vi "Main_Marvin Remake.vi"() -> ()   [LabVIEW 2017]
uses:
  PCAN_Driver/ControlCAN.llb/DevType.ctl
  PCAN_Driver/ControlCAN.llb/CAN Channel.ctl
  PCAN_Driver/ControlCAN.llb/VCI_INIT_CONFIG.ctl
  PCAN_Driver/ControlCAN.llb/InitFlag.ctl
  PCAN_Driver/ControlCAN.llb/Fliter.ctl
  PCAN_Driver/ControlCAN.llb/Mode.ctl
  <vilib>/Utility/miscctls.llb/LVRowAndColumnTypeDef.ctl
  <vilib>/Utility/sysdir.llb/System Directory Type.ctl
  <vilib>/Utility/config.llb/Read Key (String).vi
  <vilib>/Utility/config.llb/Write Key (String).vi
  <vilib>/Utility/cursorutil.llb/Set Cursor (Icon Pict).vi
  PCAN_Driver/ControlCAN.lvlib
  <vilib>/Utility/config.llb/NI_LVConfig.lvlib
panel:
  out "DSP Board S/N":string
  out "POWER Board S/N":string caption="DRIVER Board S/N"
  out "BurnInSpeed":u16
  out "SpeedCommandSpeed":u16
  out "VenableSpeed":u16
  out "CurrentTest":T1(ring)
  out "TesterVersion":string
  out "ClosePanel":bool=TRUE
  out "UUT SN Report":string
  out "Automation":bool
  out "Test Failed":bool
  out "AuxiOFFResult":bool
  out "AuxiONResult":bool
  out "SensCalResult":bool
  out "VisualInspectionResult":bool
  out "BurnResult":bool
  out "BurnSpeed":bool
  out "BurnTemp":bool
  out "BurnDC":bool
  out "TempControlResult":bool
  out "MotorTempResult":bool
  out "StopTimeResult":bool
  out "SpeedResult":bool=TRUE
  out "VenableDirectionResult":bool
  out "VenableResult":bool
  out "ComTestResult":bool=TRUE
  out "UUT SoftwareVer":string
  out "Next SN":i32
  in  "SetSN":bool
  out "Current SN":i32
  out "Cal":dbl
  out "AO[1]Meas":dbl
  out "FullSpeed2 Speed":dbl
  out "FullSpeed2 Current":dbl
  out "FullSpeed1 Current":dbl
  out "FullSpeed1 Speed":dbl
  out "MaxBurnInTempVal":dbl
  in  "Stop Burn-in":bool
  out "VISA Tester":refnum<visa-resource-name>
  out "UUT":u8
  out "CAN Status":bool
  in  "Channel 2":T2 caption="Channel" items=["Channel 1", "Channel 2"]
  out "Config_CANAT":T8 {"DevType" items=["USB-CAN"=3, "USB-CAN2"=4]; "CanIndex" items=["通道1", "通道2"]; "VCI_INIT_CONFIG"."Fliter" items=["接收所有类型"=3, "只接收标准帧"=4, "只接收扩展帧"=7]; "VCI_INIT_CONFIG"."Mode" items=["正常工作", "自测模式（环回）", "仅侦听模式"]; "VCI_INIT_CONFIG"."InitFlag" items=["使用Flash参数", "使用界面设置参数"]}
  out "Array":u64[][](array[numeric]) format="%016x"
  out "Motor Phase Current RMS":dbl
  out "Ambient Temperature":dbl
  out "Speed error":bool
  out "Commutation err":bool
  out "Under voltage/Over voltage":bool
  out "Derated drive temp":bool
  out "Motor Over temperature":bool
  out "Motor Sensor temp Fauilre":bool
  out "Drive Over temperature":bool
  out "Drive Sensor temp Failure":bool
  out "Ambient Over temp":bool
  out "Ambient Sensor temp":bool
  out "DC Voltage":dbl
  out "DC Current":dbl
  out "Power transistor Heat sink Temp.":dbl
  out "Motor Stator Temp.":dbl
  out "Motor Speed RPM":dbl
  out "ECS State":u16
  out "UUT":string="EBAY"
  in  "Logger Path":path
  in  "Report":bool
  in  "Start":bool
  in  "ATR":string[][](table)=[["Test Communication", "-", "-", "-", "-", ""], ["Set S/N", "-", "-", "-", "-", ""], ["Set Board Number", "-", "-", "-", "-", ""], [" ", "", "", "", "", ""], ["Test Communication", "-", "-", "-", "-", ""], ["Get S/N", "-", "-", "-", "", ""], ["Get Board Number", "-", "-", "-", "", ""], ["Get FW", "-", "-", "-", "", ""], ["Enable Motor", "", "", "", "", ""], ["Small position command", "", "", "", "", ""], ["Measure delta", "", "", "", "", ""], ["Velocity command", "", "", "", "", ""]]
  in  "Settings":bool
  in  "Refresh Button":bool
  out "Status":bool
  in  "VISA Marvin":refnum<visa-resource-name>="COM6"
  in  "Serial Com":bool
  in  "Help Button":bool
  out "Pannel User Message":string
  in  "Stop Button":bool
  # "Marvin"
  # "REDLER TECHNOLOGIES LTD"
  # "ver 1.2p"
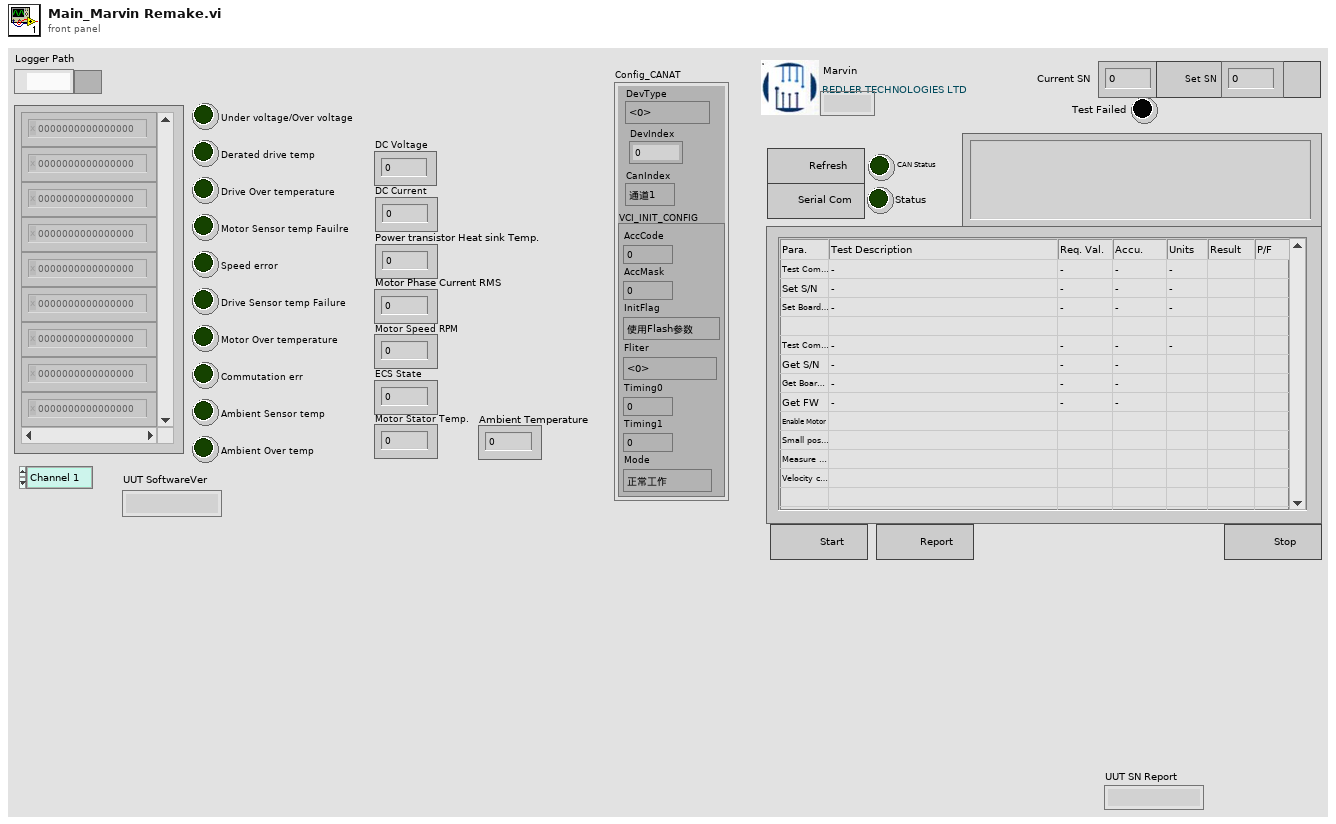
[diagram p1: front panel]
types:
  T1 = enum16{"Auxiliary", "Temp Sens Cal", "Com Test", "Enable Test", "Speed Command", "Stop Time", "Temp Control", "Burn in", "Visual Inspec", "Empty"}
  T2 = typedef "ControlCAN.lvlib/CAN Channel.ctl" = u32
  T3 = typedef "ControlCAN.lvlib/DevType.ctl" = u32
  T4 = typedef "ControlCAN.lvlib/VCI_INIT_CONFIG.ctl" = cluster{"AccCode":u32, "AccMask":u32, "InitFlag":T5, "Fliter":T6, "Timing0":u8, "Timing1":u8, "Mode":T7}
  T5 = typedef "ControlCAN.lvlib/InitFlag.ctl" = u32
  T6 = typedef "ControlCAN.lvlib/Fliter.ctl" = u8
  T7 = typedef "ControlCAN.lvlib/Mode.ctl" = u8
  T8 = cluster{"DevType":T3, "DevIndex":u32, "CanIndex":T2, "VCI_INIT_CONFIG":T4}
  T9 = cluster{"VISA":refnum<visa-resource-name>, "Array Test":enum16{"Auxiliary", "Temp Sens Cal", "Com Test", "Enable Test", "Speed Command", "Stop Time", "Temp Control", "Burn in", "Visual Inspec", "Empty"}[]}
  T10 = cluster{"ID":u32, "MSGTYPE":u8, "LEN":u8, "aDATA":u8[]}[]
  T11 = enum16{"Erase ATR Table", "Stop", "MainProgram", "Initialize"}
  T12 = typedef "NI_LVConfig.lvlib/Config Data RefNum.ctl" = refnum<k1>
  T13 = enum16{"K15", "K16", "K17", "Venable", "Firmeware", "Fan", "Power", "120C", "110C", "100C", "90C", "80C", "70C", "60C", "50C", "40C", "30C", "25C", "20C", "10C", "0C"}
  T14 = enum16{"Stop", "Result", "FullSpeed2", "MD[1]=1", "FullSpeed1", "MD[1]=0"}
  T15 = enum8{"Term1", "Term2", "Current", "Fan", "TempCPU"}
  T16 = enum16{"Stop", "AO[1]=Meas.", "TA[5]", "AO[1]=0", "Start"}
  T17 = enum16{"Stop", "BurnIn", "Ambient Temp", "MotorSpeed", "DC Current Measure", "Start"}
  T18 = enum16{"Auxiliary", "Temp Sens Cal", "Com Test", "Enable Test", "Speed Command", "Stop Time", "Temp Control", "Burn in", "Visual Inspec", "Empty"}[]
  T19 = enum16{"K15", "K16", "K17", "Venable", "Firmeware", "Fan", "Power", "120C", "110C", "100C", "90C", "80C", "70C", "60C", "50C", "40C", "30C", "25C", "20C", "10C", "0C"}[]
  T20 = enum32{"6000", "11500", "15100", "11500-2", "6000-2"}[]
  T21 = enum8{"Enabled", "Disabled", "Disabled and Grayed Out"}
  T22 = typedef "LVRowAndColumnTypeDef.ctl" = cluster{"Row":i32, "Column":i32}
  T23 = enum32{"Invalid", "Standard", "Closed", "Hidden", "Minimized", "Maximized"}
  T24 = cluster{"ID":u32, "MSGTYPE":u8, "LEN":u8, "aDATA":u8[]}
  T25 = enum16{"open", "replace", "create", "open or create", "replace or create", "replace or create with confirmation"}
  T26 = typedef "ControlCAN.lvlib/VCI_CAN_OBJ.ctl" = cluster{"ID":u32, "TimeStamp":u32, "TimeFlag":u8, "SendType":u8, "RemoteFlag":u8, "ExternFlag":u8, "DataLen":u8, "Data":u8[], "Reserved":u8[]}
  T27 = cluster{"Type":enum16{"接收", "发送"}, "Channel":T2, "Time":timestamp, "VCI_CAN_OBJ":T26}[]
  T28 = cluster{"Type":enum16{"接收", "发送"}, "Channel":T2, "Time":timestamp, "VCI_CAN_OBJ":T26}
  T29 = typedef "LVPoint32TypeDef.ctl" = cluster{"Horizontal":i32, "Vertical":i32}
  T30 = enum8{"Term1", "Term2", "Current", "Fan", "TempCPU"}[]
  T31 = typedef "System Directory Type.ctl" = i32
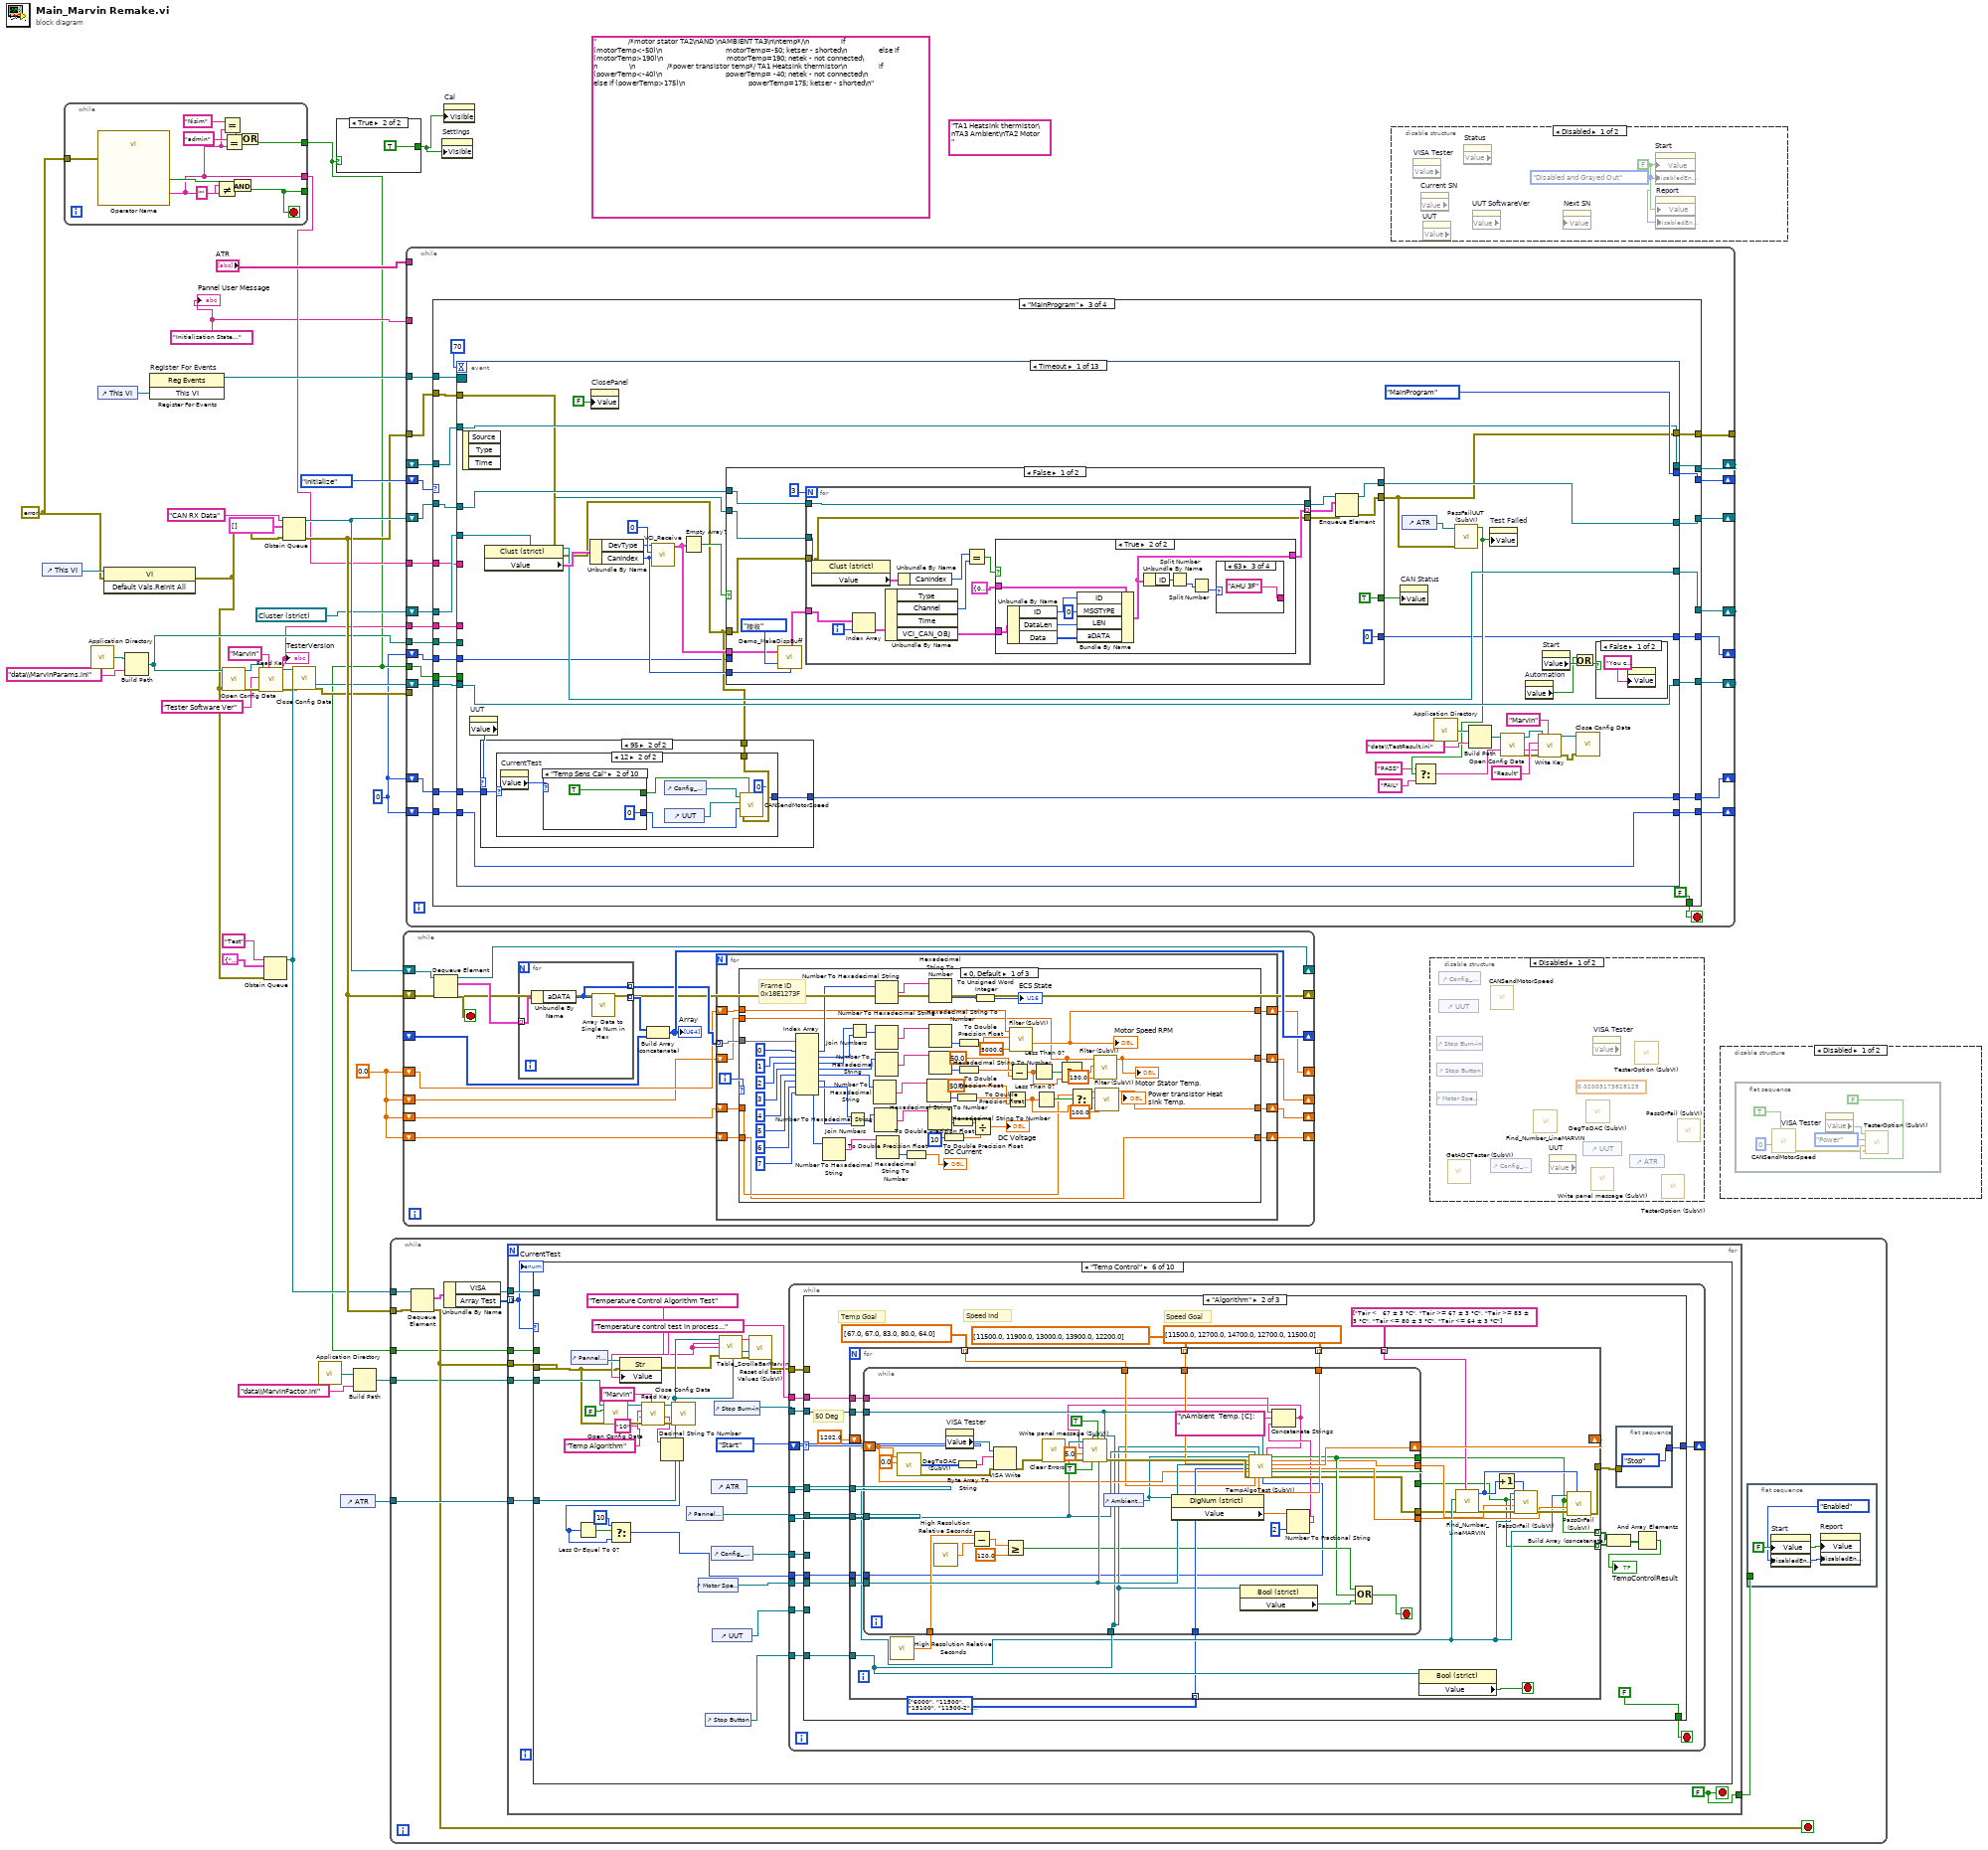
[diagram p0: block diagram]
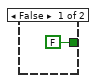
[diagram p2: hidden frame]
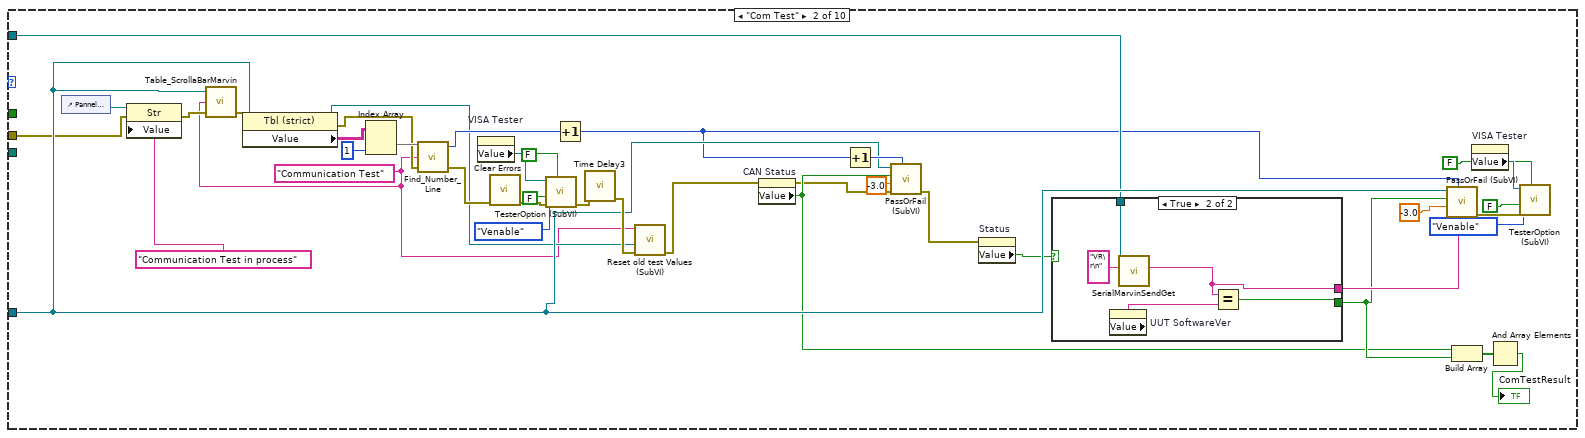
[diagram p7: hidden frame]
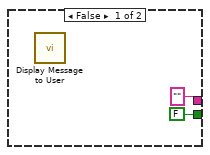
[diagram p8: hidden frame]
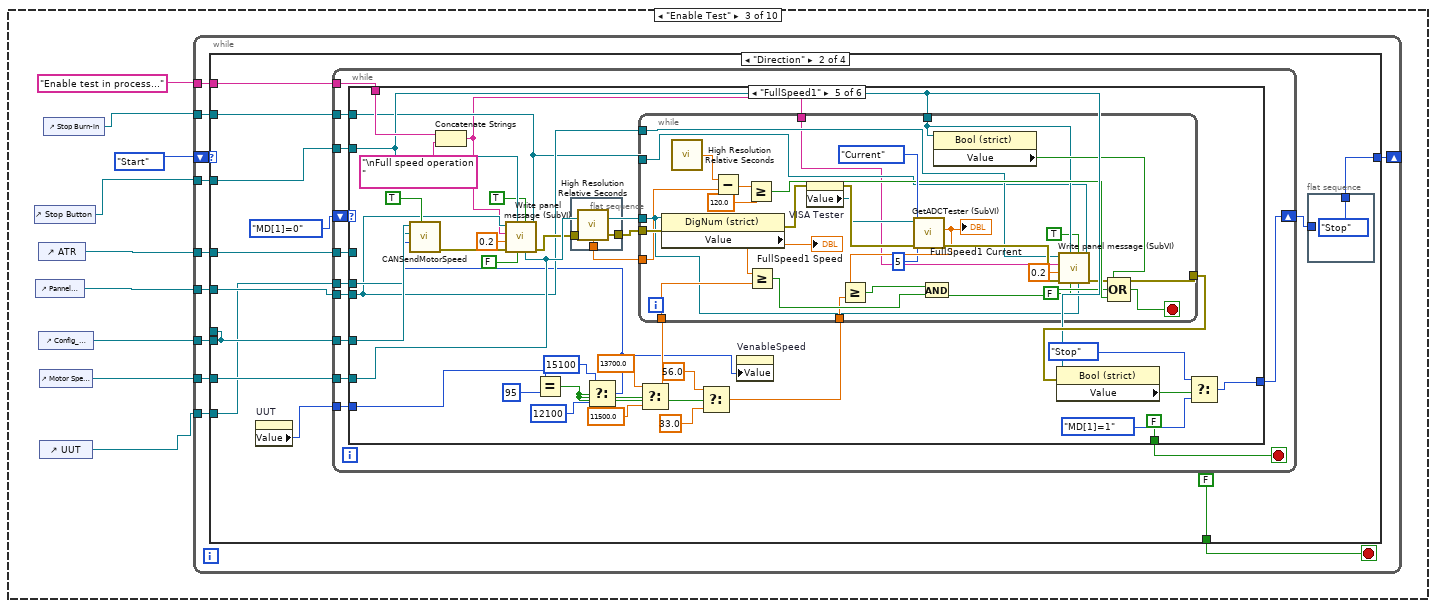
[diagram p9: hidden frame]
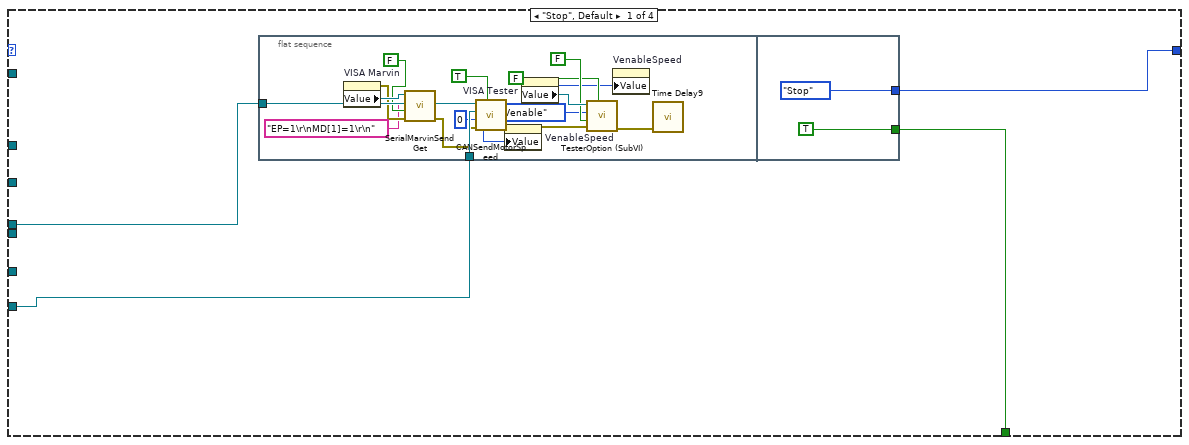
[diagram p10: hidden frame]
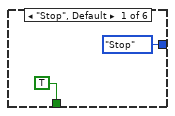
[diagram p11: hidden frame]
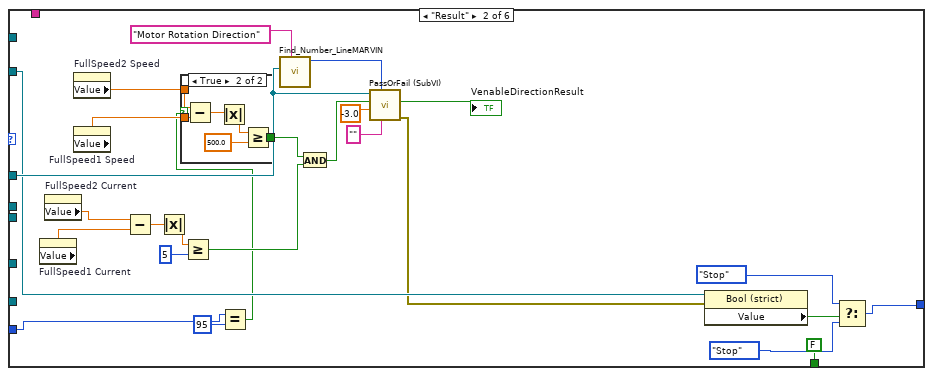
[diagram p12: hidden frame]
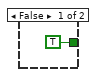
[diagram p13: hidden frame]
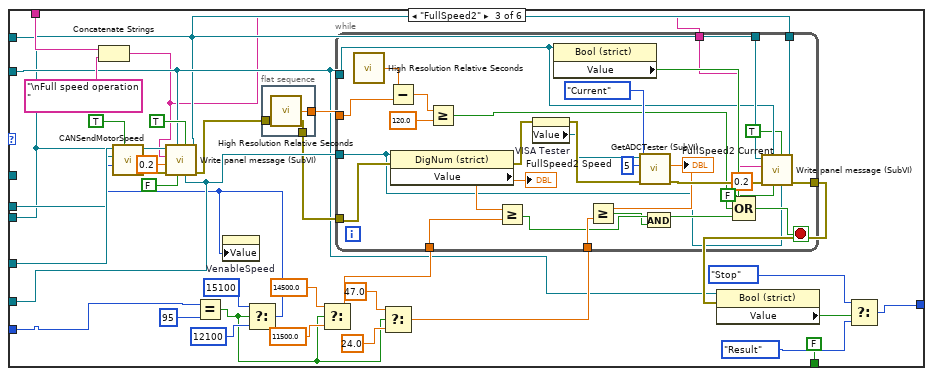
[diagram p14: hidden frame]
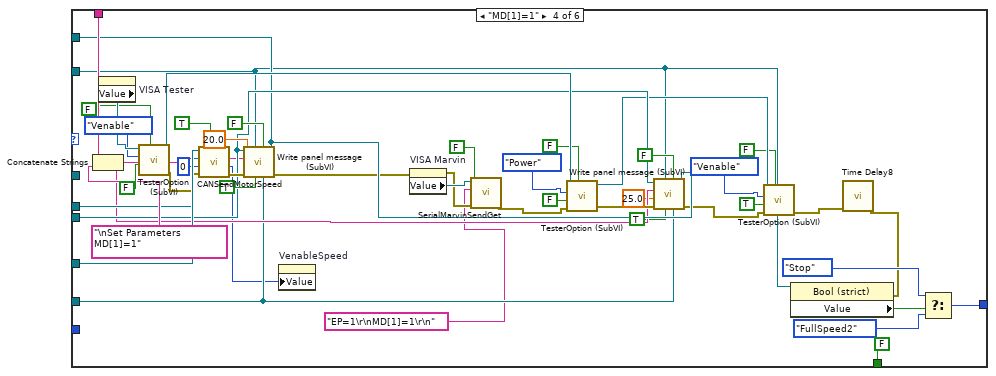
[diagram p15: hidden frame]
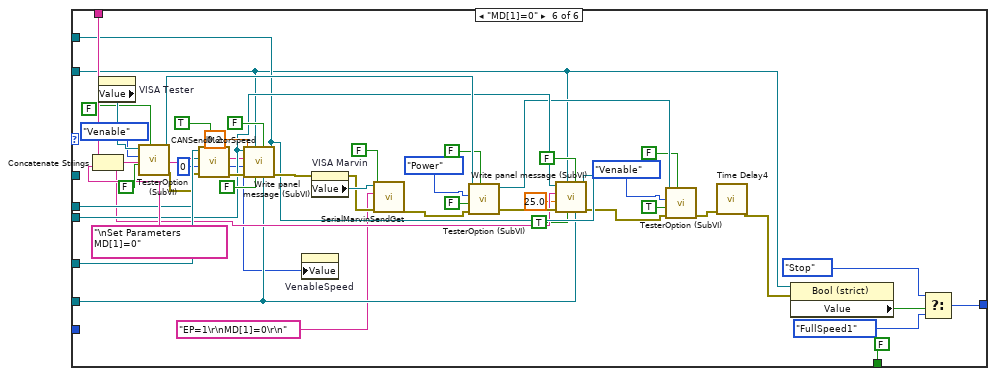
[diagram p16: hidden frame]
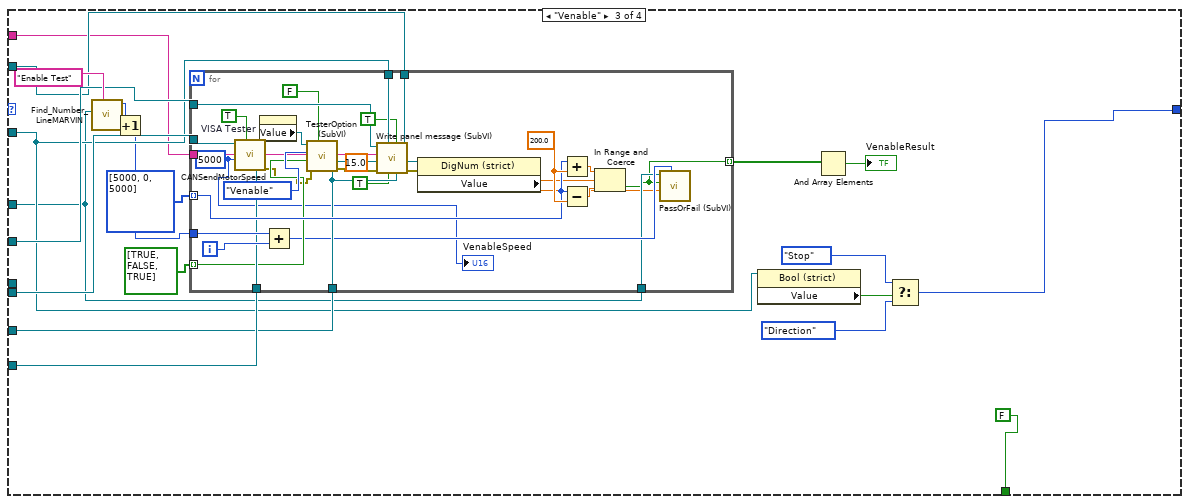
[diagram p17: hidden frame]
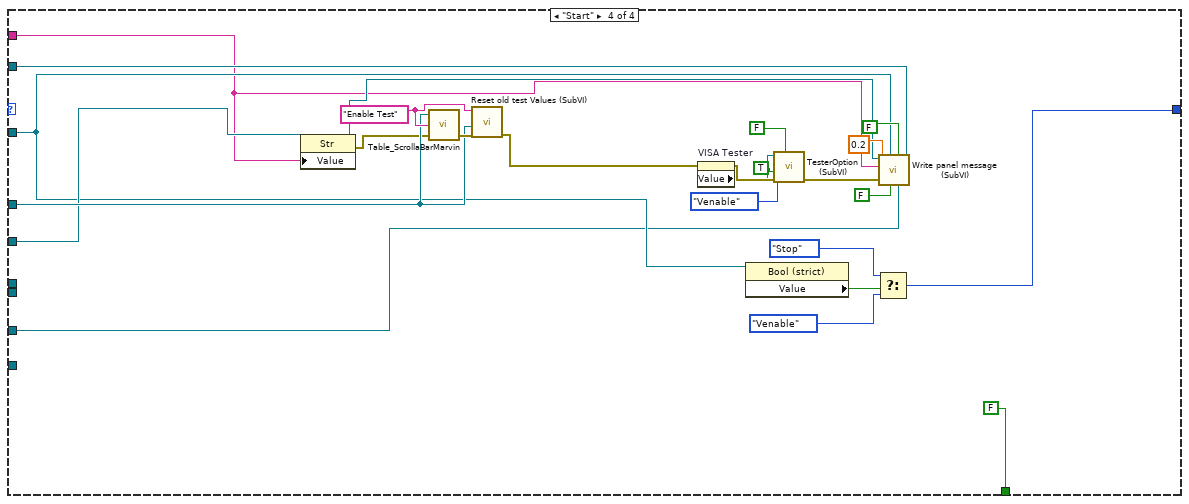
[diagram p18: hidden frame]
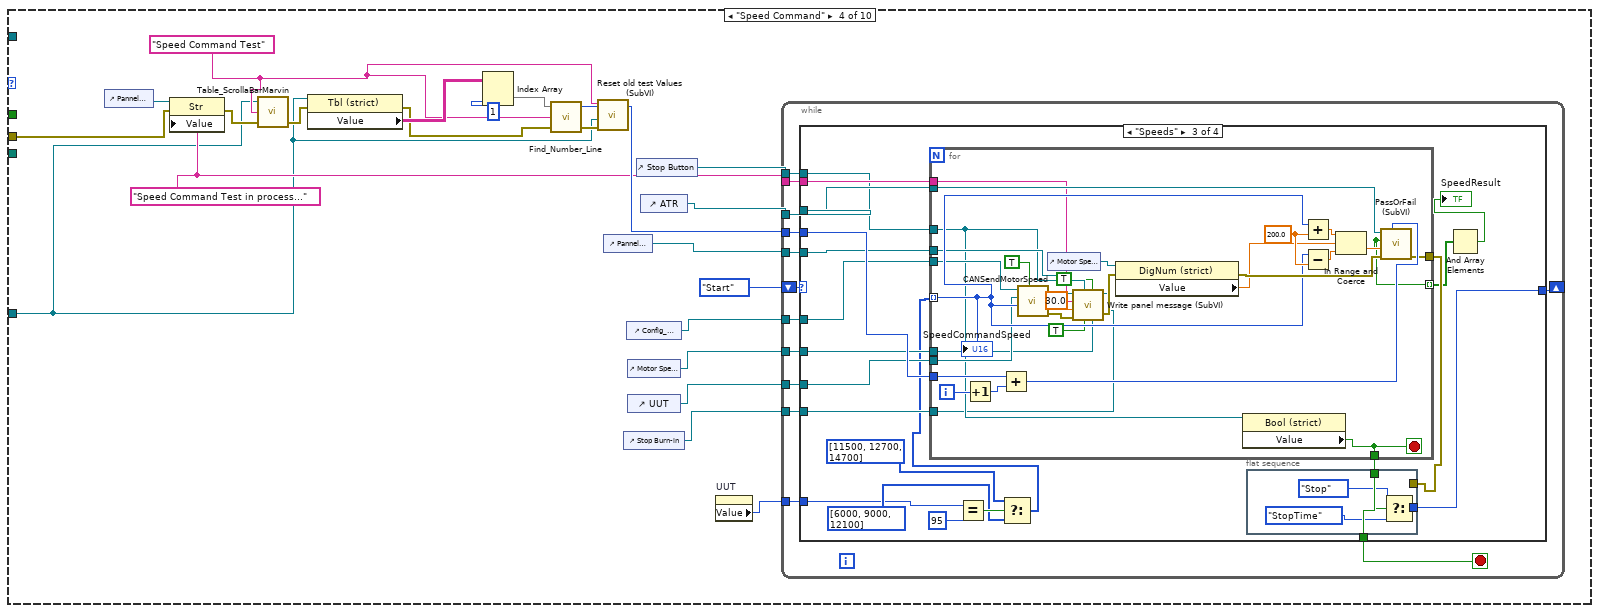
[diagram p19: hidden frame]
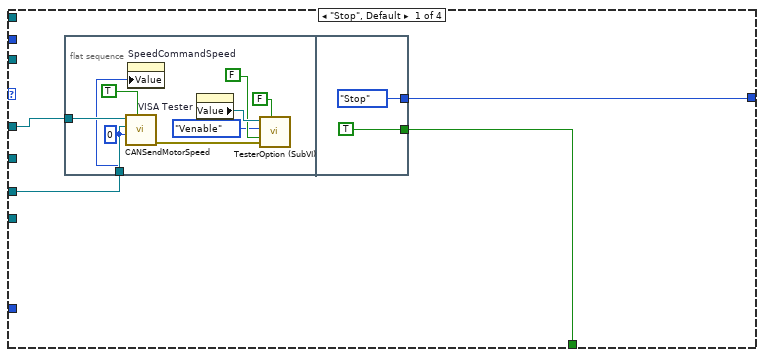
[diagram p20: hidden frame]
diagram:
  (unwired) "TA1 Heatsink thermistor\nTA3 Ambient\nTA2 Motor "
  (unwired) "                /*motor stator TA2\nAND \nAMBIENT TA3\n\ntemp*/\n                if (motorTemp<-50)\n                                motorTemp=-50; ketser - shorted\n                else if (motorTemp>190)\n                                motorTemp=190; netek - not connected\n                \n                /*power transistor temp*/ TA1 Heatsink thermistor\n                if (powerTemp<-40)\n                                powerTemp= -40; netek - not connected\n                else if (powerTemp>175)\n                                powerTemp=175; ketser - shorted\n"
  w19 = "Initialization State..."
  w1 = 0
  w26 = 0.0
  w4 = errorcluster {"status"=FALSE, "code"=0, "source"=""} ("error in (no error)")
  n1 = control-ref of="This VI"() -> (w5:refnum<vi>)
  n2 = while {
    tunnel: [w44] -> _
    tunnel: [w40] -> w21
    tunnel: [w41] -> w2
    tunnel: w4 -> [w37]
    stop <- w44 stop-if-true
    n3 = call "Operator Name"("error in (no error)"=w37) -> ("Operator Name"=w40:string, "OK"=w45:bool)  [unwired: 16 in, 1 out]
    n4 = Not Equal?(x=w40, y="") -> (x != y?=w46:bool)
    n5 = Equal?(x="Nisim", y=w40) -> (x = y?=w38:bool)
    n6 = Equal?(x="admin", y=w40) -> (x = y?=w42:bool)
    n7 = And(x=w45, y=w46) -> (x .and. y?=w44:bool)
    n8 = Or(x=w38, y=w42) -> (x .or. y?=w41:bool)
  }
  n9 = call <vilib>:"Application Directory.vi"() -> ("Application Directory"=w25:path)
  n10 = control-ref of="This VI"() -> (w23:refnum<vi>)
  n11 = invoke class="VI" method="Default Vals.Reinit All"(reference=w5, error in=w4) -> (error out=w3:errorcluster)  [unwired: 1 in, 2 out]
  n12 = Build Path(base path=w25, name or relative path="data\\MarvinParams.ini") -> (appended path=w8:path)
  n13 = register-events "Register For Events"(w23) -> (reference out=w22:refnum<event-registration>)  [unwired: 2 in, 1 out]
  n14 = call <vilib>:"Open Config Data.vi"("error in (no error)"=w3, "configuration file path"=w8) -> ("error out"=w14:errorcluster, "refnum"=w13:T12)  [unwired: 1 in, 7 out]
  n15 = call-poly <vilib>:"Read Key.vi"("section"="Marvin", "error in (no error)"=w14, "key"="Tester Software Ver", "refnum"=w13) -> ("error out"=w11:errorcluster, "value"=w6:string, "refnum out"=w10:T12)  [unwired: 2 in, 3 out]
  "TesterVersion" <- w6
  n16 = Obtain Queue(name (unnamed)="Test", element data type=T9 {"VISA"="COM1", "Array Test"=[]}, error in (no error)=w3) -> (queue out=w30:refnum<queue>)  [unwired: 2 in, 2 out]
  n17 = Obtain Queue(name (unnamed)="CAN RX Data", element data type=T10 [], error in (no error)=w3) -> (queue out=w33:refnum<queue>, error out=w31:errorcluster)  [unwired: 2 in, 1 out]
  n18 = call <vilib>:"Close Config Data.vi"("error in (no error)"=w11, "refnum"=w10) -> ("error out"=w9:errorcluster)  [unwired: 8 in, 1 out]
  n19 = call <vilib>:"Application Directory.vi"() -> ("Application Directory"=w16:path)
  n20 = case shown="True" w2 {
    tunnel: [FALSE TRUE] -> w20
    frame False {
    }
    frame True {
    }
  }
  n21 = control-ref of="ATR"() -> (w18:refnum<vi>)
  n22 = Build Path(base path=w16, name or relative path="data\\MarvinFactor.ini") -> (appended path=w15:path)
  n23 = while {
    tunnel: w18 -> [w59]
    tunnel: w31 -> [w57]
    tunnel: w30 -> [w58]
    tunnel: w15 -> [w51]
    tunnel: w2 -> [w50]
    stop <- w53 stop-if-true
    n24 = Dequeue Element(queue=w58, error in (no error)=w57) -> (element=w56:T9, error out=w53:errorcluster)  [unwired: 1 in, 2 out]
    n25 = Unbundle By Name(w56) -> ("VISA"=w55:refnum<visa-resource-name>, "Array Test"=w54:T18)
    n26 = for {
      tunnel: w54 -> [w65] mode=indexing
      tunnel: w55 -> [w68]
      tunnel: w59 -> [w67]
      tunnel: w53 -> [w66]
      tunnel: [w64] -> w52
      tunnel: w51 -> [w63]
      tunnel: w50 -> [w62]
      stop <- w64 stop-if-true
      w64 = FALSE
      n27 = case shown="\"Temp Control\"" w65 {
        tunnel: w68 -> [_ w93 _ _ w682 _ _ _ w1289 w1496]
        tunnel: w67 -> [_ w100 _ w517 w678 w855 _ w1249 w1296 w1509]
        tunnel: w66 -> [_ w97 _ w532 w688 w837 _ w1247 w1294 w1508]
        tunnel: w63 -> [_ _ _ _ _ w839 _ _ _ _]
        tunnel: w62 -> [_ _ _ _ _ _ w1007 _ _ _]
        frame "Empty", Default {
        }
        frame "Com Test" {
          w76 = "Communication Test" ("Test Paragraph")
          n28 = control-ref of="Pannel User Message"() -> (w98:refnum<vi>)
          n29 = property class="Str"(reference=w98, error in=w97, "Value"="Communication Test in process") -> (error out=w96:errorcluster)  [unwired: 1 out]
          n30 = call "Table_ScrollaBarMarvin.vi"("error in"=w96, "Line to focus"=w76, "reference in"=w100) -> ("error out"=w99:errorcluster)  [unwired: 2 out]
          n31 = property class="Tbl (strict)"(reference=w100, error in=w99) -> (reference out=w77:refnum<vi>, error out=w106:errorcluster, "Value"=w107:string[][])
          n32 = Index Array(array=w107, index (col)=1 ("disabled index (col)")) -> (element=w108:string[])  [unwired: 1 in]
          n33 = call "Find_Number_Line.vi"("error in"=w106, "Test Paragraph"=w76, "Row Headers[]"=w108) -> ("error out"=w104:errorcluster, "Line number"=w103:i32)  [unwired: 1 out]
          n34 = property on="VISA Tester" class="VISAName"() -> ("Value"=w87:refnum<visa-resource-name>)  [unwired: 2 in, 2 out]
          n35 = call <vilib>:"Clear Errors.vi"("error in (no error)"=w104) -> ("error out"=w89:errorcluster)  [unwired: 5 in, 1 out]
          n36 = call "TesterOption (SubVI).vi"("2 Options"=FALSE, "error in (no error)"=w89, "On/Off"=FALSE, "Tester Option"=T13."Venable", "VISA Refnum in"=w87) -> ("error out"=w88:errorcluster)  [unwired: 5 in, 1 out]
          n37 = Increment(x=w103) -> (x+1=w69:i32)
          n38 = call "Time Delay3"("error in (no error)"=w88) -> ("error out"=w101:errorcluster)  [unwired: 10 in]
          n39 = call "Reset old test Values (SubVI).vi"("error in"=w101, "Atr in"=w77, "Test Paragraph"=w76) -> ("error out"=w71:errorcluster)  [unwired: 8 in]
          n40 = property on="CAN Status" class="Bool (strict)"(error in=w71) -> (error out=w70:errorcluster, "Value"=w72:bool)  [unwired: 1 in, 1 out]
          n41 = Increment(x=w69) -> (x+1=w102:i32)
          n42 = call "PassOrFail (SubVI).vi"("index (row)"=w102, "error in (no error)"=w70, "Data in"=-3.0, "Pass?Fail"=w72, "Table in"=w100) -> ("error out"=w92:errorcluster)  [unwired: 6 in]
          n43 = property on="Status" class="Bool (strict)"(error in=w92) -> ("Value"=w94:bool)  [unwired: 1 in, 2 out]
          n44 = case shown="True" w94 {
            tunnel: w93 -> [_ w115]
            tunnel: [FALSE w112] -> w74
            tunnel: ["" ("read buffer") w111] -> w91
            frame False {
              n45 = call "Display Message to User"() -> ()  [unwired: 10 in, 2 out]
            }
            frame True {
              n46 = property on="UUT SoftwareVer" class="Str"() -> ("Value"=w113:string)  [unwired: 2 in, 2 out]
              n47 = call "SerialMarvinSendGet.vi"("write buffer"="VR\r\n", "VISA resource name"=w115) -> ("read buffer"=w111:string)  [unwired: 8 in, 1 out]
              n48 = Equal?(x=w111, y=w113) -> (x = y?=w112:bool)
            }
          }
          n49 = call "PassOrFail (SubVI).vi"("String Res"=w91, "index (row)"=w69, "Data in"=-3.0, "Pass?Fail"=w74, "Table in"=w100) -> ("error out"=w83:errorcluster)  [unwired: 6 in]
          n50 = Build Array(w72, w74) -> (w75:bool[])
          n51 = property on="VISA Tester" class="VISAName"() -> ("Value"=w82:refnum<visa-resource-name>)  [unwired: 2 in, 2 out]
          n52 = And Array Elements(Boolean array=w75) -> (logical AND=→"ComTestResult":bool)
          n53 = call "TesterOption (SubVI).vi"("2 Options"=FALSE, "error in (no error)"=w83, "On/Off"=FALSE, "Tester Option"=T13."Venable", "VISA Refnum in"=w82) -> ()  [unwired: 5 in, 2 out]
        }
        frame "Enable Test" {
          n54 = control-ref of="Stop Button"() -> (w118:refnum<vi>)
          n55 = control-ref of="Pannel User Message"() -> (w120:refnum<vi>)
          n56 = control-ref of="ATR"() -> (w119:refnum<vi>)
          n57 = control-ref of="Config_CANAT"() -> (w121:refnum<vi>)
          n58 = control-ref of="Motor Speed RPM"() -> (w122:refnum<vi>)
          n59 = control-ref of="UUT"() -> (w123:refnum<vi>)
          n60 = control-ref of="Stop Burn-in"() -> (w124:refnum<vi>)
          n61 = while {
            shift-right: [w129] -> _
            shift-left: enum16{"Stop", "Direction", "Venable", "Start"}."Start" -> [w135]
            tunnel: w118 -> [w134]
            tunnel: w119 -> [w133]
            tunnel: w120 -> [w132]
            tunnel: w121 -> [w125]
            tunnel: w122 -> [w131]
            tunnel: w123 -> [w126]
            tunnel: w124 -> [w128]
            tunnel: "Enable test in process..." ("Strin") -> [w127]
            stop <- w130 stop-if-true
            n62 = case shown="\"Direction\"" w135 {
              tunnel: w134 -> [_ w167 w449 w496]
              tunnel: w133 -> [_ w162 w447 w503]
              tunnel: w132 -> [_ w165 w451 w502]
              tunnel: w125 -> [_ w168 w454 _]
              tunnel: w131 -> [_ w164 w452 w494]
              tunnel: w126 -> [w136 w158 w453 _]
              tunnel: [w139 FALSE FALSE FALSE] -> w130
              tunnel: [w137 w161 w448 w500] -> w129
              tunnel: w128 -> [_ w166 w450 w495]
              tunnel: w127 -> [_ w163 w446 w493]
              tunnel: w125 -> [w138 _ _ _]
              frame "Stop", Default {
                n63 = flat-sequence {
                  tunnel: w136 -> [w151]
                  tunnel: w138 -> [w150]
                  tunnel: [TRUE] -> w139
                  tunnel: [enum16{"Stop", "Direction", "Venable", "Start"}."Stop"] -> w137
                  frame #0 {
                    w140 = u16 0 ("Motor Speed RPM")
                    n64 = property on="VISA Marvin" class="VISAName"() -> (error out=w144:errorcluster, "Value"=w145:refnum<visa-resource-name>)  [unwired: 2 in, 1 out]
                    n65 = call "SerialMarvinSendGet.vi"("error in (no error)"=w144, "Clear Log"=FALSE, "write buffer"="EP=1\r\nMD[1]=1\r\n", "VISA resource name"=w145) -> ("error out"=w141:errorcluster)  [unwired: 6 in, 1 out]
                    n66 = call "CANSendMotorSpeed.vi"("Remote"=TRUE, "error in (no error)"=w141, "Motor Speed RPM"=w140, "UUT"=w151, "CAN Cluster in"=w150) -> ("error out"=w153:errorcluster)  [unwired: 6 in]
                    n67 = property on="VenableSpeed" class="DigNum (strict)"("Value"=w140) -> ()  [unwired: 2 in, 2 out]
                    n68 = property on="VISA Tester" class="VISAName"() -> ("Value"=w154:refnum<visa-resource-name>)  [unwired: 2 in, 2 out]
                    n69 = call "TesterOption (SubVI).vi"("2 Options"=FALSE, "error in (no error)"=w153, "On/Off"=FALSE, "Tester Option"=T13."Venable", "VISA Refnum in"=w154) -> ("error out"=w146:errorcluster)  [unwired: 5 in, 1 out]
                    n70 = property on="VenableSpeed" class="DigNum (strict)"("Value"=w140) -> ()  [unwired: 2 in, 2 out]
                    n71 = call "Time Delay9"("error in (no error)"=w146) -> ()  [unwired: 10 in, 1 out]
                  }
                  frame #1 {
                  }
                }
              }
              frame "Direction" {
                n72 = property on="UUT" class="DigNum (strict)"() -> ("Value"=w157:u8)  [unwired: 2 in, 2 out]
                n73 = while {
                  shift-right: [w181] -> w160
                  shift-left: T14."MD[1]=0" -> [w182]
                  tunnel: w168 -> [w179]
                  tunnel: w158 -> [w178]
                  tunnel: w167 -> [w177]
                  tunnel: w166 -> [w176]
                  tunnel: w165 -> [w175]
                  tunnel: w164 -> [w174]
                  tunnel: w163 -> [w173]
                  tunnel: w162 -> [w172]
                  tunnel: w157 -> [w171]
                  stop <- w180 stop-if-true
                  n74 = case shown="\"FullSpeed1\"" w182 {
                    tunnel: [T14."Stop" w206 w248 w328 w361 w441] -> w181
                    tunnel: [TRUE FALSE FALSE FALSE FALSE FALSE] -> w180
                    tunnel: w179 -> [_ _ w246 w322 w359 w435]
                    tunnel: w178 -> [_ _ w242 w302 w355 w414]
                    tunnel: w177 -> [_ w193 w222 w293 w338 w404]
                    tunnel: w176 -> [_ _ w220 w303 w336 w415]
                    tunnel: w175 -> [_ _ w221 w304 w337 w416]
                    tunnel: w174 -> [_ _ w238 w291 w352 w410]
                    tunnel: w173 -> [_ _ w233 w312 w350 w424]
                    tunnel: w172 -> [_ w197 _ _ _ _]
                    tunnel: w171 -> [_ w185 w218 _ w331 _]
                    frame "Stop", Default {
                    }
                    frame "Result" {
                      n75 = property on="FullSpeed1 Current" class="DigNum (strict)"() -> ("Value"=w201:dbl)  [unwired: 2 in, 2 out]
                      n76 = property on="FullSpeed2 Current" class="DigNum (strict)"() -> ("Value"=w202:dbl)  [unwired: 2 in, 2 out]
                      n77 = property on="FullSpeed2 Speed" class="DigNum (strict)"() -> ("Value"=w204:dbl)  [unwired: 2 in, 2 out]
                      n78 = property on="FullSpeed1 Speed" class="DigNum (strict)"() -> ("Value"=w203:dbl)  [unwired: 2 in, 2 out]
                      n79 = Subtract(x=w202, y=w201) -> (x-y=w200:dbl)
                      n80 = Absolute Value(x=w200) -> (abs(x)=w189:dbl)
                      n81 = Greater Or Equal?(x=w189, y=u32 5) -> (x >= y?=w195:bool)
                      n82 = Equal?(x=w185, y=u8 95) -> (x = y?=w187:bool)
                      n83 = case shown="True" w187 {
                        tunnel: w204 -> [_ w215]
                        tunnel: w203 -> [_ w214]
                        tunnel: [TRUE w211] -> w196
                        frame False {
                        }
                        frame True {
                          n84 = Subtract(x=w215, y=w214) -> (x-y=w216:dbl)
                          n85 = Absolute Value(x=w216) -> (abs(x)=w213:dbl)
                          n86 = Greater Or Equal?(x=w213, y=500.0) -> (x >= y?=w211:bool)
                        }
                      }
                      n87 = call "Find_Number_LineMARVIN.vi"("Test Paragraph"="Motor Rotation Direction", "TableIn"=w197) -> ("Line number"=w194:i32)  [unwired: 3 in, 3 out]
                      n88 = And(x=w196, y=w195) -> (x .and. y?=w186:bool)
                      "VenableDirectionResult" <- w186
                      n89 = call "PassOrFail (SubVI).vi"("String Res"="", "index (row)"=w194, "Data in"=-3.0, "Pass?Fail"=w186, "Table in"=w197) -> ("error out"=w192:errorcluster)  [unwired: 6 in]
                      n90 = property class="Bool (strict)"(reference=w193, error in=w192) -> ("Value"=w209:bool)  [unwired: 2 out]
                      n91 = Select(t=T14."Stop", s=w209, f=T14."Stop") -> (s? t:f=w206:T14)
                    }
                    frame "FullSpeed2" {
                      n92 = Concatenate Strings(w233, "\nFull speed operation " ("string")) -> (w219:string)
                      n93 = Equal?(x=w218, y=u8 95) -> (x = y?=w228:bool)
                      n94 = Select(t=u16 15100, s=w228, f=u16 12100 ("y")) -> (s? t:f=w217:u16)
                      n95 = call "CANSendMotorSpeed.vi"("Remote"=TRUE, "Motor Speed RPM"=w217, "UUT"=w242, "CAN Cluster in"=w246) -> ("error out"=w240:errorcluster)  [unwired: 7 in]
                      n96 = call "Write panel message (SubVI).vi"("Stop BurnIn"=w220, 4:"rpm"=w238, 5:"rpm"=TRUE ("rpm"), "PrintTime"=FALSE, "Stop"=w222, "error in (no error)"=w240, "Time to wait"=0.2, "Strin"=w219, "String in"=w221) -> ("error out"=w225:errorcluster)  [unwired: 2 in]
                      n97 = property on="VenableSpeed" class="DigNum (strict)"("Value"=w217) -> ()  [unwired: 2 in, 2 out]
                      n98 = flat-sequence {
                        tunnel: w225 -> [w253]
                        tunnel: [w253] -> w224
                        tunnel: [w252] -> w223
                        frame #0 {
                          n99 = call <vilib>:"High Resolution Relative Seconds.vi"() -> ("relative seconds"=w252:dbl)
                        }
                      }
                      n100 = Select(t=14500.0, s=w228, f=11500.0) -> (s? t:f=w227:dbl)
                      n101 = Select(t=47.0, s=w228, f=24.0) -> (s? t:f=w226:dbl)
                      n102 = while {
                        tunnel: w238 -> [w255]
                        tunnel: w224 -> [w283]
                        tunnel: [w263] -> w235
                        tunnel: w227 -> [w276]
                        tunnel: w226 -> [w275]
                        tunnel: w223 -> [w271]
                        tunnel: w222 -> [w261]
                        tunnel: w221 -> [w262]
                        tunnel: w220 -> [w259]
                        tunnel: w219 -> [w258]
                        stop <- w273 stop-if-true
                        n103 = call <vilib>:"High Resolution Relative Seconds.vi"() -> ("relative seconds"=w272:dbl)
                        n104 = Subtract(x=w272, y=w271) -> (x-y=w270:dbl)
                        n105 = property class="DigNum (strict)"(reference=w255, error in=w283) -> (error out=w282:errorcluster, "Value"=w277:dbl)  [unwired: 1 out]
                        "FullSpeed2 Speed" <- w277
                        n106 = Greater Or Equal?(x=w270, y=120.0) -> (x >= y?=w268:bool)
                        n107 = Greater Or Equal?(x=w277, y=w276) -> (x >= y?=w267:bool)
                        n108 = property on="VISA Tester" class="VISAName"(error in=w282) -> (error out=w281:errorcluster, "Value"=w280:refnum<visa-resource-name>)  [unwired: 1 in, 1 out]
                        n109 = property class="Bool (strict)"(reference=w261) -> ("Value"=w266:bool)  [unwired: 1 in, 2 out]
                        n110 = call "GetADCTester (SubVI).vi"("error in (no error)"=w281, "GetADCTester"=T15."Current", "TimeToGet"=5, "VISA Refnum in"=w280) -> ("error out"=w278:errorcluster, "ADCValOutput Single"=w274:dbl)  [unwired: 5 in, 1 out]
                        "FullSpeed2 Current" <- w274
                        n111 = Greater Or Equal?(x=w274, y=w275) -> (x >= y?=w264:bool)
                        n112 = And(x=w267, y=w264) -> (x .and. y?=w265:bool)
                        n113 = Compound Arithmetic op=OR(w266, w268, w265) -> (w273:bool)
                        n114 = call "Write panel message (SubVI).vi"("Stop BurnIn"=w259, 4:"rpm"=w255, 5:"rpm"=TRUE ("rpm"), "PrintTime"=FALSE, "Stop"=w261, "error in (no error)"=w278, "Time to wait"=0.2, "Strin"=w258, "String in"=w262) -> ("error out"=w263:errorcluster)  [unwired: 2 in]
                      }
                      n115 = property class="Bool (strict)"(reference=w222, error in=w235) -> ("Value"=w251:bool)  [unwired: 2 out]
                      n116 = Select(t=T14."Stop", s=w251, f=T14."Result") -> (s? t:f=w248:T14)
                    }
                    frame "MD[1]=1" {
                      w284 = u16 0 ("Motor Speed RPM")
                      n117 = Concatenate Strings(w312, "\nSet Parameters MD[1]=1" ("Strin")) -> (w301:string)
                      n118 = property on="VISA Tester" class="VISAName"() -> ("Value"=w317:refnum<visa-resource-name>)  [unwired: 2 in, 2 out]
                      n119 = call "TesterOption (SubVI).vi"("2 Options"=FALSE, "On/Off"=FALSE, "Tester Option"=T13."Venable", "VISA Refnum in"=w317) -> ("error out"=w318:errorcluster, "VISA Refnum out"=w308:refnum<visa-resource-name>)  [unwired: 6 in]
                      n120 = call "CANSendMotorSpeed.vi"("Remote"=TRUE, "error in (no error)"=w318, "Motor Speed RPM"=w284, "UUT"=w302, "CAN Cluster in"=w322) -> ("error out"=w320:errorcluster)  [unwired: 6 in]
                      n121 = call "Write panel message (SubVI).vi"("Stop BurnIn"=w303, 4:"rpm"=w291, 5:"rpm"=FALSE ("rpm"), "PrintTime"=TRUE, "Stop"=w293, "error in (no error)"=w320, "Time to wait"=20.0, "Strin"=w301, "String in"=w304) -> ("error out"=w290:errorcluster)  [unwired: 2 in]
                      n122 = property on="VenableSpeed" class="DigNum (strict)"("Value"=w284) -> ()  [unwired: 2 in, 2 out]
                      n123 = property on="VISA Marvin" class="VISAName"(error in=w290) -> (error out=w319:errorcluster, "Value"=w324:refnum<visa-resource-name>)  [unwired: 1 in, 1 out]
                      n124 = call "SerialMarvinSendGet.vi"("error in (no error)"=w319, "Clear Log"=FALSE, "write buffer"="EP=1\r\nMD[1]=1\r\n", "VISA resource name"=w324) -> ("error out"=w307:errorcluster)  [unwired: 6 in, 1 out]
                      n125 = call "TesterOption (SubVI).vi"("2 Options"=FALSE, "error in (no error)"=w307, "On/Off"=FALSE, "Tester Option"=T13."Power", "VISA Refnum in"=w308) -> ("error out"=w305:errorcluster, "VISA Refnum out"=w294:refnum<visa-resource-name>)  [unwired: 5 in]
                      n126 = call "Write panel message (SubVI).vi"("Stop BurnIn"=w303, 4:"rpm"=w291, 5:"rpm"=FALSE ("rpm"), "PrintTime"=TRUE, "Stop"=w293, "error in (no error)"=w305, "Time to wait"=25.0, "Strin"=w301, "String in"=w304) -> ("error out"=w295:errorcluster)  [unwired: 2 in]
                      n127 = call "TesterOption (SubVI).vi"("2 Options"=FALSE, "error in (no error)"=w295, "On/Off"=TRUE, "Tester Option"=T13."Venable", "VISA Refnum in"=w294) -> ("error out"=w292:errorcluster)  [unwired: 5 in, 1 out]
                      n128 = call "Time Delay8"("error in (no error)"=w292) -> ("error out"=w288:errorcluster)  [unwired: 10 in]
                      n129 = property class="Bool (strict)"(reference=w293, error in=w288) -> ("Value"=w329:bool)  [unwired: 2 out]
                      n130 = Select(t=T14."Stop", s=w329, f=T14."FullSpeed2") -> (s? t:f=w328:T14)
                    }
                    frame "FullSpeed1" {
                      n131 = Concatenate Strings(w350, "\nFull speed operation " ("string")) -> (w335:string)
                      n132 = Equal?(x=w331, y=u8 95) -> (x = y?=w348:bool)
                      n133 = flat-sequence {
                        tunnel: w341 -> [w366]
                        tunnel: [w366] -> w340
                        tunnel: [w365] -> w339
                        frame #0 {
                          n134 = call <vilib>:"High Resolution Relative Seconds.vi"() -> ("relative seconds"=w365:dbl)
                        }
                      }
                      n135 = Select(t=u16 15100, s=w348, f=u16 12100 ("y")) -> (s? t:f=w330:u16)
                      n136 = call "CANSendMotorSpeed.vi"("Remote"=TRUE, "Motor Speed RPM"=w330, "UUT"=w355, "CAN Cluster in"=w359) -> ("error out"=w353:errorcluster)  [unwired: 7 in]
                      n137 = call "Write panel message (SubVI).vi"("Stop BurnIn"=w336, 4:"rpm"=w352, 5:"rpm"=TRUE ("rpm"), "PrintTime"=FALSE, "Stop"=w338, "error in (no error)"=w353, "Time to wait"=0.2, "Strin"=w335, "String in"=w337) -> ("error out"=w341:errorcluster)  [unwired: 2 in]
                      n138 = Select(t=13700.0, s=w348, f=11500.0) -> (s? t:f=w343:dbl)
                      n139 = Select(t=56.0, s=w348, f=33.0) -> (s? t:f=w342:dbl)
                      n140 = while {
                        tunnel: w352 -> [w368]
                        tunnel: w340 -> [w396]
                        tunnel: [w376] -> w351
                        tunnel: w343 -> [w388]
                        tunnel: w342 -> [w385]
                        tunnel: w339 -> [w383]
                        tunnel: w338 -> [w374]
                        tunnel: w337 -> [w375]
                        tunnel: w336 -> [w372]
                        tunnel: w335 -> [w371]
                        stop <- w390 stop-if-true
                        n141 = property class="DigNum (strict)"(reference=w368, error in=w396) -> (error out=w395:errorcluster, "Value"=w389:dbl)  [unwired: 1 out]
                        "FullSpeed1 Speed" <- w389
                        n142 = call <vilib>:"High Resolution Relative Seconds.vi"() -> ("relative seconds"=w384:dbl)
                        n143 = Subtract(x=w384, y=w383) -> (x-y=w382:dbl)
                        n144 = Greater Or Equal?(x=w382, y=120.0) -> (x >= y?=w380:bool)
                        n145 = Greater Or Equal?(x=w389, y=w388) -> (x >= y?=w387:bool)
                        n146 = property on="VISA Tester" class="VISAName"(error in=w395) -> (error out=w394:errorcluster, "Value"=w393:refnum<visa-resource-name>)  [unwired: 1 in, 1 out]
                        n147 = call "GetADCTester (SubVI).vi"("error in (no error)"=w394, "GetADCTester"=T15."Current", "TimeToGet"=5, "VISA Refnum in"=w393) -> ("error out"=w391:errorcluster, "ADCValOutput Single"=w386:dbl)  [unwired: 5 in, 1 out]
                        "FullSpeed1 Current" <- w386
                        n148 = Greater Or Equal?(x=w386, y=w385) -> (x >= y?=w377:bool)
                        n149 = And(x=w377, y=w387) -> (x .and. y?=w378:bool)
                        n150 = property class="Bool (strict)"(reference=w374) -> ("Value"=w379:bool)  [unwired: 1 in, 2 out]
                        n151 = call "Write panel message (SubVI).vi"("Stop BurnIn"=w372, 4:"rpm"=w368, 5:"rpm"=TRUE ("rpm"), "PrintTime"=FALSE, "Stop"=w374, "error in (no error)"=w391, "Time to wait"=0.2, "Strin"=w371, "String in"=w375) -> ("error out"=w376:errorcluster)  [unwired: 2 in]
                        n152 = Compound Arithmetic op=OR(w379, w378, w380) -> (w390:bool)
                      }
                      n153 = property on="VenableSpeed" class="DigNum (strict)"("Value"=w330) -> ()  [unwired: 2 in, 2 out]
                      n154 = property class="Bool (strict)"(reference=w338, error in=w351) -> ("Value"=w364:bool)  [unwired: 2 out]
                      n155 = Select(t=T14."Stop", s=w364, f=T14."MD[1]=1") -> (s? t:f=w361:T14)
                    }
                    frame "MD[1]=0" {
                      w397 = u16 0 ("Motor Speed RPM")
                      n156 = Concatenate Strings(w424, "\nSet Parameters MD[1]=0" ("Strin")) -> (w413:string)
                      n157 = property on="VISA Tester" class="VISAName"() -> ("Value"=w430:refnum<visa-resource-name>)  [unwired: 2 in, 2 out]
                      n158 = call "TesterOption (SubVI).vi"("2 Options"=FALSE, "On/Off"=FALSE, "Tester Option"=T13."Venable", "VISA Refnum in"=w430) -> ("error out"=w431:errorcluster, "VISA Refnum out"=w420:refnum<visa-resource-name>)  [unwired: 6 in]
                      n159 = call "CANSendMotorSpeed.vi"("Remote"=TRUE, "error in (no error)"=w431, "Motor Speed RPM"=w397, "UUT"=w414, "CAN Cluster in"=w435) -> ("error out"=w433:errorcluster)  [unwired: 6 in]
                      n160 = call "Write panel message (SubVI).vi"("Stop BurnIn"=w415, 4:"rpm"=w410, 5:"rpm"=FALSE ("rpm"), "PrintTime"=FALSE, "Stop"=w404, "error in (no error)"=w433, "Time to wait"=0.2, "Strin"=w413, "String in"=w416) -> ("error out"=w427:errorcluster)  [unwired: 2 in]
                      n161 = property on="VenableSpeed" class="DigNum (strict)"("Value"=w397) -> ()  [unwired: 2 in, 2 out]
                      n162 = property on="VISA Marvin" class="VISAName"(error in=w427) -> (error out=w432:errorcluster, "Value"=w437:refnum<visa-resource-name>)  [unwired: 1 in, 1 out]
                      n163 = call "SerialMarvinSendGet.vi"("error in (no error)"=w432, "Clear Log"=FALSE, "write buffer"="EP=1\r\nMD[1]=0\r\n", "VISA resource name"=w437) -> ("error out"=w419:errorcluster)  [unwired: 6 in, 1 out]
                      n164 = call "TesterOption (SubVI).vi"("2 Options"=FALSE, "error in (no error)"=w419, "On/Off"=FALSE, "Tester Option"=T13."Power", "VISA Refnum in"=w420) -> ("error out"=w417:errorcluster, "VISA Refnum out"=w405:refnum<visa-resource-name>)  [unwired: 5 in]
                      n165 = call "Write panel message (SubVI).vi"("Stop BurnIn"=w415, 4:"rpm"=w410, 5:"rpm"=FALSE ("rpm"), "PrintTime"=TRUE, "Stop"=w404, "error in (no error)"=w417, "Time to wait"=25.0, "Strin"=w413, "String in"=w416) -> ("error out"=w406:errorcluster)  [unwired: 2 in]
                      n166 = call "TesterOption (SubVI).vi"("2 Options"=FALSE, "error in (no error)"=w406, "On/Off"=TRUE, "Tester Option"=T13."Venable", "VISA Refnum in"=w405) -> ("error out"=w403:errorcluster)  [unwired: 5 in, 1 out]
                      n167 = call "Time Delay4"("error in (no error)"=w403) -> ("error out"=w399:errorcluster)  [unwired: 10 in]
                      n168 = property class="Bool (strict)"(reference=w404, error in=w399) -> ("Value"=w442:bool)  [unwired: 2 out]
                      n169 = Select(t=T14."Stop", s=w442, f=T14."FullSpeed1") -> (s? t:f=w441:T14)
                    }
                  }
                }
                n170 = flat-sequence {
                  tunnel: [enum16{"Stop", "Direction", "Venable", "Start"}."Stop"] -> w161
                  tunnel: w160 -> [_]
                  frame #0 {
                  }
                }
              }
              frame "Venable" {
                n171 = call "Find_Number_LineMARVIN.vi"("Test Paragraph"="Enable Test", "TableIn"=w447) -> ("Line number"=w455:i32)  [unwired: 3 in, 3 out]
                n172 = Increment(x=w455) -> (x+1=w443:i32)
                n173 = for {
                  tunnel: u16[] [5000, 0, 5000] -> [w485] mode=indexing
                  tunnel: bool[] [TRUE, FALSE, TRUE] -> [w481] mode=indexing
                  tunnel: w443 -> [w486]
                  tunnel: w454 -> [w484]
                  tunnel: w453 -> [w483]
                  tunnel: w452 -> [w472]
                  tunnel: w451 -> [w476]
                  tunnel: w449 -> [w475]
                  tunnel: w450 -> [w474]
                  tunnel: w447 -> [w468]
                  tunnel: w446 -> [w466]
                  tunnel: [w465] -> w445 mode=indexing
                  i -> [w487]
                  w463 = u16 5000 ("Motor Speed RPM")
                  w489 = 200.0 ("y")
                  n174 = call "CANSendMotorSpeed.vi"("Remote"=TRUE, "Motor Speed RPM"=w463, "UUT"=w483, "CAN Cluster in"=w484) -> ("error out"=w480:errorcluster)  [unwired: 7 in]
                  n175 = property on="VISA Tester" class="VISAName"() -> ("Value"=w479:refnum<visa-resource-name>)  [unwired: 2 in, 2 out]
                  n176 = Add(x=w486, y=w487) -> (x+y=w469:i32)
                  n177 = call "TesterOption (SubVI).vi"("2 Options"=FALSE, "error in (no error)"=w480, "On/Off"=w481, "Tester Option"=T13."Venable", "VISA Refnum in"=w479) -> ("error out"=w478:errorcluster)  [unwired: 5 in, 1 out]
                  n178 = call "Write panel message (SubVI).vi"("Stop BurnIn"=w474, 4:"rpm"=w472, 5:"rpm"=TRUE ("rpm"), "PrintTime"=TRUE, "Stop"=w475, "error in (no error)"=w478, "Time to wait"=15.0, "Strin"=w466, "String in"=w476) -> ("error out"=w477:errorcluster)  [unwired: 2 in]
                  n179 = property class="DigNum (strict)"(reference=w472, error in=w477) -> ("Value"=w467:dbl)  [unwired: 2 out]
                  n180 = Add(x=w485, y=w489) -> (x+y=w491:dbl)
                  n181 = Subtract(x=w485, y=w489) -> (x-y=w490:dbl)
                  n182 = In Range and Coerce(upper limit=w491, x=w467, lower limit=w490) -> (In Range?=w465:bool)  [unwired: 1 out]
                  n183 = call "PassOrFail (SubVI).vi"("index (row)"=w469, "Data in"=w467, "Pass?Fail"=w465, "Table in"=w468) -> ()  [unwired: 7 in, 1 out]
                  "VenableSpeed" <- w463
                }
                n184 = property class="Bool (strict)"(reference=w449) -> ("Value"=w462:bool)  [unwired: 1 in, 2 out]
                n185 = And Array Elements(Boolean array=w445) -> (logical AND=→"VenableResult":bool)
                n186 = Select(t=enum16{"Stop", "Direction", "Venable", "Start"}."Stop", s=w462, f=enum16{"Stop", "Direction", "Venable", "Start"}."Direction") -> (s? t:f=w448:enum16{"Stop", "Direction", "Venable", "Start"})
              }
              frame "Start" {
                w511 = "Enable Test" ("Test Paragraph")
                n187 = property class="Str"(reference=w502, "Value"=w493) -> (reference out=w512:refnum<vi>, error out=w499:errorcluster)  [unwired: 1 in]
                n188 = call "Table_ScrollaBarMarvin.vi"("error in"=w499, "Line to focus"=w511, "reference in"=w503) -> ("error out"=w508:errorcluster)  [unwired: 2 out]
                n189 = call "Reset old test Values (SubVI).vi"("error in"=w508, "Atr in"=w503, "Test Paragraph"=w511) -> ("error out"=w507:errorcluster)  [unwired: 8 in]
                n190 = property on="VISA Tester" class="VISAName"(error in=w507) -> (error out=w506:errorcluster, "Value"=w505:refnum<visa-resource-name>)  [unwired: 1 in, 1 out]
                n191 = property class="Bool (strict)"(reference=w496) -> ("Value"=w516:bool)  [unwired: 1 in, 2 out]
                n192 = call "TesterOption (SubVI).vi"("2 Options"=FALSE, "error in (no error)"=w506, "On/Off"=TRUE, "Tester Option"=T13."Venable", "VISA Refnum in"=w505) -> ("error out"=w504:errorcluster)  [unwired: 5 in, 1 out]
                n193 = Select(t=enum16{"Stop", "Direction", "Venable", "Start"}."Stop", s=w516, f=enum16{"Stop", "Direction", "Venable", "Start"}."Venable") -> (s? t:f=w500:enum16{"Stop", "Direction", "Venable", "Start"})
                n194 = call "Write panel message (SubVI).vi"("Stop BurnIn"=w495, 4:"rpm"=w494, 5:"rpm"=FALSE ("rpm"), "PrintTime"=FALSE, "Stop"=w496, "error in (no error)"=w504, "Time to wait"=0.2, "Strin"=w493, "String in"=w512) -> ()  [unwired: 2 in, 1 out]
              }
            }
          }
        }
        frame "Speed Command" {
          w521 = "Speed Command Test in process..." ("Value")
          w518 = "Speed Command Test" ("Test Paragraph")
          n195 = control-ref of="Pannel User Message"() -> (w533:refnum<vi>)
          n196 = property class="Str"(reference=w533, error in=w532, "Value"=w521) -> (error out=w531:errorcluster)  [unwired: 1 out]
          n197 = call "Table_ScrollaBarMarvin.vi"("error in"=w531, "Line to focus"=w518, "reference in"=w517) -> ("error out"=w534:errorcluster)  [unwired: 2 out]
          n198 = property class="Tbl (strict)"(reference=w517, error in=w534) -> (error out=w536:errorcluster, "Value"=w537:string[][])  [unwired: 1 out]
          n199 = Index Array(array=w537, index (col)=1 ("disabled index (col)")) -> (element=w538:string[])  [unwired: 1 in]
          n200 = call "Find_Number_Line.vi"("error in"=w536, "Test Paragraph"=w518, "Row Headers[]"=w538) -> ("error out"=w519:errorcluster, "Line number"=w522:i32)  [unwired: 1 out]
          n201 = call "Reset old test Values (SubVI).vi"("error in"=w519, "Atr in"=w517, "Test Paragraph"=w518) -> ()  [unwired: 8 in, 1 out]
          n202 = control-ref of="Pannel User Message"() -> (w526:refnum<vi>)
          n203 = control-ref of="Stop Burn-in"() -> (w530:refnum<vi>)
          n204 = control-ref of="Config_CANAT"() -> (w527:refnum<vi>)
          n205 = control-ref of="Motor Speed RPM"() -> (w528:refnum<vi>)
          n206 = control-ref of="UUT"() -> (w529:refnum<vi>)
          n207 = control-ref of="Stop Button"() -> (w524:refnum<vi>)
          n208 = control-ref of="ATR"() -> (w525:refnum<vi>)
          n209 = property on="UUT" class="DigNum (strict)"() -> ("Value"=w520:u8)  [unwired: 2 in, 2 out]
          n210 = while {
            shift-right: [w550] -> _
            shift-left: enum16{"Stop", "StopTime", "Speeds", "Start"}."Start" -> [w551]
            tunnel: w524 -> [w549]
            tunnel: w525 -> [w548]
            tunnel: w526 -> [w547]
            tunnel: w527 -> [w546]
            tunnel: w528 -> [w545]
            tunnel: w529 -> [w544]
            tunnel: w530 -> [w543]
            tunnel: w522 -> [w542]
            tunnel: w521 -> [w541]
            tunnel: w520 -> [w539]
            stop <- w540 stop-if-true
            n211 = case shown="\"Speeds\"" w551 {
              tunnel: [w555 w585 w625 w669] -> w550
              tunnel: w549 -> [_ w580 w629 w667]
              tunnel: w548 -> [_ w570 w633 _]
              tunnel: w547 -> [_ w581 w630 _]
              tunnel: w546 -> [w553 w583 w632 _]
              tunnel: w545 -> [_ w578 w627 _]
              tunnel: w544 -> [w554 w582 w624 _]
              tunnel: w543 -> [_ w579 w628 _]
              tunnel: w542 -> [_ _ w634 _]
              tunnel: w541 -> [_ _ w631 _]
              tunnel: [w552 w584 w626 FALSE ("Value")] -> w540
              tunnel: w539 -> [_ _ w617 _]
              frame "Stop", Default {
                n212 = flat-sequence {
                  tunnel: w554 -> [w559]
                  tunnel: w553 -> [w558]
                  tunnel: [enum16{"Stop", "StopTime", "Speeds", "Start"}."Stop"] -> w555
                  tunnel: [TRUE] -> w552
                  frame #0 {
                    w556 = u16 0 ("Motor Speed RPM")
                    n213 = call "CANSendMotorSpeed.vi"("Remote"=TRUE, "Motor Speed RPM"=w556, "UUT"=w559, "CAN Cluster in"=w558) -> ("error out"=w563:errorcluster)  [unwired: 7 in]
                    n214 = property on="SpeedCommandSpeed" class="DigNum (strict)"("Value"=w556) -> ()  [unwired: 2 in, 2 out]
                    n215 = property on="VISA Tester" class="VISAName"() -> ("Value"=w564:refnum<visa-resource-name>)  [unwired: 2 in, 2 out]
                    n216 = call "TesterOption (SubVI).vi"("2 Options"=FALSE, "error in (no error)"=w563, "On/Off"=FALSE, "Tester Option"=T13."Venable", "VISA Refnum in"=w564) -> ()  [unwired: 5 in, 2 out]
                  }
                  frame #1 {
                  }
                }
              }
              frame "StopTime" {
                w567 = u16 0 ("Motor Speed RPM")
                n217 = call "Table_ScrollaBarMarvin.vi"("Line to focus"="Motor Stop time", "reference in"=w570) -> ("error out"=w571:errorcluster)  [unwired: 1 in, 2 out]
                n218 = property on="SpeedCommandSpeed" class="DigNum (strict)"("Value"=w567) -> ()  [unwired: 2 in, 2 out]
                n219 = call "CANSendMotorSpeed.vi"("Remote"=TRUE, "error in (no error)"=w571, "Motor Speed RPM"=w567, "UUT"=w582, "CAN Cluster in"=w583) -> ("error out"=w588:errorcluster)  [unwired: 6 in]
                n220 = flat-sequence {
                  tunnel: [w614] -> w587
                  tunnel: w588 -> [w613]
                  tunnel: [w613] -> w589
                  frame #0 {
                    n221 = call <vilib>:"High Resolution Relative Seconds.vi"() -> ("relative seconds"=w614:dbl)
                  }
                }
                n222 = while {
                  tunnel: [w609] -> w584
                  tunnel: w581 -> [w607]
                  tunnel: w580 -> [w606]
                  tunnel: w579 -> [w604]
                  tunnel: w578 -> [w603]
                  tunnel: "Stop Time Test in process..." ("Value") -> [w591]
                  tunnel: [w599] -> w568
                  tunnel: w589 -> [w611]
                  tunnel: [w600] -> w576
                  tunnel: w587 -> [w610]
                  tunnel: [w598] -> w572
                  stop <- w590 stop-if-true
                  n223 = call "Write panel message (SubVI).vi"("Stop BurnIn"=w604, 4:"rpm"=w603, 5:"rpm"=TRUE ("rpm"), "PrintTime"=FALSE, "Stop"=w606, "error in (no error)"=w611, "Time to wait"=0.1, "Strin"=w591, "String in"=w607) -> ("error out"=w608:errorcluster)  [unwired: 2 in]
                  n224 = control-ref of="Motor Speed RPM"() -> (w597:refnum<vi>)
                  n225 = property class="DigNum (strict)"(reference=w597, error in=w608) -> (error out=w600:errorcluster, "Value"=w596:dbl)  [unwired: 1 out]
                  n226 = call <vilib>:"High Resolution Relative Seconds.vi"() -> ("relative seconds"=w594:dbl)
                  n227 = property class="Bool (strict)"(reference=w606) -> ("Value"=w609:bool)  [unwired: 1 in, 2 out]
                  n228 = Subtract(x=w594, y=w610) -> (x-y=w598:dbl)
                  n229 = Greater Or Equal?(x=w598, y=50.0) -> (x >= y?=w592:bool)
                  n230 = Less Or Equal?(x=w596, y=0.0) -> (x <= y?=w599:bool)
                  n231 = Compound Arithmetic op=OR(w599, w592, w609) -> (w590:bool)
                }
                "StopTimeResult" <- w568
                n232 = call "Find_Number_LineMARVIN.vi"("Test Paragraph"="Motor Stop time", "TableIn"=w570) -> ("Line number"=w573:i32)  [unwired: 3 in, 3 out]
                n233 = call "PassOrFail (SubVI).vi"("index (row)"=w573, "error in (no error)"=w576, "Data in"=w572, "Pass?Fail"=w568, "Table in"=w570) -> ("error out"=w575:errorcluster)  [unwired: 6 in]
                n234 = flat-sequence {
                  tunnel: [enum16{"Stop", "StopTime", "Speeds", "Start"}."Stop"] -> w585
                  tunnel: w575 -> [_]
                  frame #0 {
                  }
                }
              }
              frame "Speeds" {
                n235 = Equal?(x=w617, y=u8 95) -> (x = y?=w622:bool)
                n236 = Select(t=u16[] [11500, 12700, 14700], s=w622, f=u16[] [6000, 9000, 12100]) -> (s? t:f=w619:u16[])
                n237 = for {
                  tunnel: w619 -> [w660] mode=indexing
                  tunnel: w634 -> [w653]
                  tunnel: w633 -> [w652]
                  tunnel: w624 -> [w651]
                  tunnel: w632 -> [w650]
                  tunnel: w631 -> [w649]
                  tunnel: w630 -> [w648]
                  tunnel: w629 -> [w647]
                  tunnel: w628 -> [w645]
                  tunnel: w627 -> [w643]
                  tunnel: [w641] -> w626
                  tunnel: [w640] -> w618
                  tunnel: [w639] -> w616 mode=indexing
                  i -> [w659]
                  stop <- w641 stop-if-true
                  w661 = 200.0 ("y")
                  n238 = Increment(x=w659) -> (x+1=w658:i32)
                  n239 = Add(x=w653, y=w658) -> (x+y=w654:i32)
                  n240 = call "CANSendMotorSpeed.vi"("Remote"=TRUE, "Motor Speed RPM"=w660, "UUT"=w651, "CAN Cluster in"=w650) -> ("error out"=w665:errorcluster)  [unwired: 7 in]
                  n241 = control-ref of="Motor Speed RPM"() -> (w666:refnum<vi>)
                  n242 = call "Write panel message (SubVI).vi"("Stop BurnIn"=w645, 4:"rpm"=w643, 5:"rpm"=TRUE ("rpm"), "PrintTime"=TRUE, "Stop"=w647, "error in (no error)"=w665, "Time to wait"=30.0 ("Delay Time (sec)"), "Strin"=w649, "String in"=w648) -> ("error out"=w657:errorcluster)  [unwired: 2 in]
                  n243 = property class="DigNum (strict)"(reference=w666, error in=w657) -> (error out=w664:errorcluster, "Value"=w642:dbl)  [unwired: 1 out]
                  n244 = property class="Bool (strict)"(reference=w647) -> ("Value"=w641:bool)  [unwired: 1 in, 2 out]
                  n245 = Add(x=w660, y=w661) -> (x+y=w663:dbl)
                  n246 = Subtract(x=w660, y=w661) -> (x-y=w662:dbl)
                  n247 = In Range and Coerce(upper limit=w663, x=w642, lower limit=w662) -> (In Range?=w639:bool)  [unwired: 1 out]
                  n248 = call "PassOrFail (SubVI).vi"("index (row)"=w654, "error in (no error)"=w664, "Data in"=w642, "Pass?Fail"=w639, "Table in"=w652) -> ("error out"=w640:errorcluster)  [unwired: 6 in]
                  "SpeedCommandSpeed" <- w660
                }
                n249 = flat-sequence {
                  tunnel: w626 -> [w638]
                  tunnel: [w636] -> w625
                  tunnel: w618 -> [_]
                  frame #0 {
                    n250 = Select(t=enum16{"Stop", "StopTime", "Speeds", "Start"}."Stop", s=w638, f=enum16{"Stop", "StopTime", "Speeds", "Start"}."StopTime") -> (s? t:f=w636:enum16{"Stop", "StopTime", "Speeds", "Start"})
                  }
                }
                n251 = And Array Elements(Boolean array=w616) -> (logical AND=→"SpeedResult":bool)
              }
              frame "Start" {
                n252 = property on="VISA Tester" class="VISAName"() -> ("Value"=w677:refnum<visa-resource-name>)  [unwired: 2 in, 2 out]
                n253 = call "TesterOption (SubVI).vi"("2 Options"=FALSE, "On/Off"=TRUE, "Tester Option"=T13."Venable", "VISA Refnum in"=w677) -> ("error out"=w668:errorcluster)  [unwired: 6 in, 1 out]
                n254 = property class="Bool (strict)"(reference=w667, error in=w668) -> ("Value"=w673:bool)  [unwired: 2 out]
                n255 = Select(t=enum16{"Stop", "StopTime", "Speeds", "Start"}."Stop", s=w673, f=enum16{"Stop", "StopTime", "Speeds", "Start"}."Speeds") -> (s? t:f=w669:enum16{"Stop", "StopTime", "Speeds", "Start"})
              }
            }
          }
        }
        frame "Stop Time" {
          w681 = "Motor Temperature test in process..." ("Value")
          w679 = "Motor Termistor Input Test" ("Test Paragraph")
          n256 = control-ref of="Pannel User Message"() -> (w689:refnum<vi>)
          n257 = property class="Str"(reference=w689, error in=w688, "Value"=w681) -> (error out=w687:errorcluster)  [unwired: 1 out]
          n258 = call "Table_ScrollaBarMarvin.vi"("error in"=w687, "Line to focus"=w679, "reference in"=w678) -> ("error out"=w691:errorcluster)  [unwired: 2 out]
          n259 = property class="Tbl (strict)"(reference=w678, error in=w691) -> (reference out=w684:refnum<vi>, error out=w693:errorcluster, "Value"=w694:string[][])
          n260 = Index Array(array=w694, index (col)=1 ("disabled index (col)")) -> (element=w695:string[])  [unwired: 1 in]
          n261 = call "Find_Number_LineMARVIN.vi"("Test Paragraph"=w679, "error in"=w693, "TableIn"=w678, "Row Headers[]"=w695) -> ("error out"=w690:errorcluster, "Line number"=w683:i32)  [unwired: 1 in, 2 out]
          n262 = call "Reset old test Values (SubVI).vi"("error in"=w690, "Atr in"=w678, "Test Paragraph"=w679) -> ("error out"=w680:errorcluster)  [unwired: 8 in]
          n263 = property on="Status" class="Bool (strict)"(error in=w680) -> (error out=w685:errorcluster, "Value"=w686:bool)  [unwired: 1 in, 1 out]
          n264 = case shown="True" w686 {
            selector: w686 -> [w699 _]
            tunnel: w685 -> [w701 _]
            tunnel: w684 -> [w698 _]
            tunnel: w683 -> [w697 w704]
            tunnel: w682 -> [_ w709]
            tunnel: w681 -> [_ w705]
            frame False {
              n265 = flat-sequence {
                tunnel: w701 -> [w702]
                tunnel: [w702] -> w700
                frame #0 {
                  n266 = One Button Dialog(message="Please establish RS connection.") -> ()  [unwired: 1 in, 1 out]
                }
              }
              n267 = Increment(x=w697) -> (x+1=w696:i32)
              n268 = call "PassOrFail (SubVI).vi"("index (row)"=w696, "error in (no error)"=w700, "Pass?Fail"=w699, "Table in"=w698) -> ()  [unwired: 7 in, 1 out]
            }
            frame True {
              n269 = control-ref of="Stop Burn-in"() -> (w711:refnum<vi>)
              n270 = control-ref of="Pannel User Message"() -> (w713:refnum<vi>)
              n271 = control-ref of="Config_CANAT"() -> (w707:refnum<vi>)
              n272 = control-ref of="ATR"() -> (w714:refnum<vi>)
              n273 = control-ref of="Motor Speed RPM"() -> (w715:refnum<vi>)
              n274 = control-ref of="UUT"() -> (w706:refnum<vi>)
              n275 = control-ref of="Stop Button"() -> (w712:refnum<vi>)
              n276 = property on="VISA Tester" class="VISAName"() -> ("Value"=w708:refnum<visa-resource-name>)  [unwired: 2 in, 2 out]
              n277 = while {
                shift-right: [w719] -> _
                shift-left: T16."Start" -> [w729]
                tunnel: w711 -> [w728]
                tunnel: w712 -> [w727]
                tunnel: w713 -> [w726]
                tunnel: w714 -> [w725]
                tunnel: w715 -> [w724]
                tunnel: w709 -> [w723]
                tunnel: w708 -> [w722]
                tunnel: w707 -> [w721]
                tunnel: w706 -> [w720]
                tunnel: w705 -> [w717]
                tunnel: w704 -> [w716]
                stop <- w718 stop-if-true
                n278 = case shown="\"Start\"" w729 {
                  tunnel: w728 -> [_ w752 w811]
                  tunnel: w727 -> [_ w744 w813]
                  tunnel: w726 -> [_ w753 w815]
                  tunnel: w725 -> [_ w742 _]
                  tunnel: w724 -> [_ w751 w810]
                  tunnel: w723 -> [_ w756 _]
                  tunnel: w722 -> [w732 w755 w804]
                  tunnel: w721 -> [_ _ w821]
                  tunnel: w720 -> [_ _ w820]
                  tunnel: [w730 w745 w806] -> w719
                  tunnel: [w731 FALSE FALSE] -> w718
                  tunnel: w717 -> [_ w754 _]
                  tunnel: w716 -> [_ w741 _]
                  frame "Stop", Default {
                    n279 = flat-sequence {
                      tunnel: w732 -> [w733]
                      tunnel: [TRUE] -> w731
                      tunnel: [T16."Stop"] -> w730
                      frame #0 {
                        n280 = call "TesterOption (SubVI).vi"("2 Options"=FALSE, "On/Off"=FALSE, "Tester Option"=T13."Venable", "VISA Refnum in"=w733) -> ()  [unwired: 6 in, 2 out]
                      }
                      frame #1 {
                      }
                    }
                  }
                  frame "TA[5]" {
                    w757 = T19 [enum."60C", enum."90C", enum."120C"] items=["K15", "K16", "K17", "Venable", "Firmeware", "Fan", "Power", "120C", "110C", "100C", "90C", "80C", "70C", "60C", "50C", "40C", "30C", "25C", "20C", "10C", "0C"]
                    n281 = for {
                      tunnel: w757 -> [w781] mode=indexing
                      tunnel: w756 -> [w780]
                      tunnel: w755 -> [w779]
                      tunnel: w754 -> [w778]
                      tunnel: w753 -> [w777]
                      tunnel: w744 -> [w776]
                      tunnel: w752 -> [w775]
                      tunnel: w751 -> [w774]
                      tunnel: dbl[] [60.0, 90.0, 120.0] -> [w764] mode=indexing
                      tunnel: [w763] -> w743
                      tunnel: w742 -> [w770]
                      tunnel: w741 -> [w769]
                      tunnel: [w758] -> w740 mode=indexing
                      i -> [w767]
                      w762 = 3.0 ("y")
                      n282 = for {
                        N: 5 -> [_]
                        tunnel: w781 -> [w783]
                        tunnel: w780 -> [w799]
                        tunnel: w779 -> [w795]
                        tunnel: w778 -> [w793]
                        tunnel: w777 -> [w792]
                        tunnel: w776 -> [w791]
                        tunnel: w775 -> [w789]
                        tunnel: w774 -> [w786]
                        tunnel: [w785] -> w773 mode=indexing
                        tunnel: [w784] -> w771
                        n283 = call "TesterOption (SubVI).vi"("2 Options"=FALSE, "On/Off"=TRUE, "Tester Option"=w783, "VISA Refnum in"=w795) -> ("error out"=w796:errorcluster)  [unwired: 6 in, 1 out]
                        n284 = call "Write panel message (SubVI).vi"("Stop BurnIn"=w789, 4:"rpm"=w786, 5:"rpm"=FALSE ("rpm"), "PrintTime"=FALSE, "Stop"=w791, "error in (no error)"=w796, "Time to wait"=1.0, "Strin"=w793, "String in"=w792) -> ("error out"=w794:errorcluster)  [unwired: 2 in]
                        n285 = call "SerialMarvinSendGet.vi"("error in (no error)"=w794, "write buffer"="TA[2]\r\n", "VISA resource name"=w799) -> ("error out"=w784:errorcluster, "read buffer"=w797:string)  [unwired: 7 in]
                        n286 = Fract/Exp String To Number(string=w797) -> (number=w785:dbl)  [unwired: 3 in, 1 out]
                      }
                      n287 = Increment(x=w767) -> (x+1=w766:i32)
                      n288 = Add Array Elements(numeric array=w773) -> (sum=w772:dbl)
                      n289 = Add(x=w764, y=w762) -> (x+y=w761:dbl)
                      n290 = Subtract(x=w764, y=w762) -> (x-y=w760:dbl)
                      n291 = Divide(x=w772, y=5.0) -> (x/y=w759:dbl)
                      n292 = In Range and Coerce(upper limit=w761, x=w759, lower limit=w760) -> (In Range?=w758:bool)  [unwired: 1 out]
                      n293 = Add(x=w769, y=w766) -> (x+y=w768:i32)
                      n294 = call "PassOrFail (SubVI).vi"("index (row)"=w768, "error in (no error)"=w771, "Data in"=w759, "Pass?Fail"=w758, "Table in"=w770) -> ("error out"=w763:errorcluster)  [unwired: 6 in]
                    }
                    n295 = property class="Bool (strict)"(reference=w744, error in=w743) -> ("Value"=w749:bool)  [unwired: 2 out]
                    n296 = Select(t=T16."Stop", s=w749, f=T16."Stop") -> (s? t:f=w745:T16)
                    n297 = And Array Elements(Boolean array=w740) -> (logical AND=→"MotorTempResult":bool)
                  }
                  frame "Start" {
                    n298 = call "Write panel message (SubVI).vi"("Stop BurnIn"=w811, 4:"rpm"=w810, 5:"rpm"=FALSE ("rpm"), "PrintTime"=FALSE, "Stop"=w813, "Time to wait"=0.1, "Strin"="Motor Temperature test in process...\nInitialization state...", "String in"=w815) -> ("error out"=w816:errorcluster)  [unwired: 3 in]
                    n299 = call "TesterOption (SubVI).vi"("2 Options"=FALSE, "error in (no error)"=w816, "On/Off"=FALSE, "Tester Option"=T13."Venable", "VISA Refnum in"=w804) -> ("error out"=w818:errorcluster)  [unwired: 5 in, 1 out]
                    n300 = call "CANSendMotorSpeed.vi"("Remote"=TRUE, "error in (no error)"=w818, "Motor Speed RPM"=u16 0, "UUT"=w820, "CAN Cluster in"=w821) -> ("error out"=w803:errorcluster)  [unwired: 6 in]
                    n301 = property class="Bool (strict)"(reference=w813, error in=w803) -> ("Value"=w825:bool)  [unwired: 2 out]
                    n302 = Select(t=T16."Stop", s=w825, f=T16."TA[5]") -> (s? t:f=w806:T16)
                  }
                }
              }
            }
          }
        }
        frame "Temp Control" {
          w843 = "Temperature control test in process..." ("Value")
          w841 = "Temperature Control Algorithm Test" ("Test Paragraph")
          n303 = control-ref of="Pannel User Message"() -> (w854:refnum<vi>)
          n304 = call <vilib>:"Open Config Data.vi"("error in (no error)"=w837, "create file if necessary (T)"=FALSE, "configuration file path"=w839) -> ("error out"=w840:errorcluster, "refnum"=w836:T12)  [unwired: 7 out]
          n305 = property class="Str"(reference=w854, error in=w837, "Value"=w843) -> (error out=w853:errorcluster)  [unwired: 1 out]
          n306 = call-poly <vilib>:"Read Key.vi"("section"="Marvin", "error in (no error)"=w840, "default value"="10", "key"="Temp Algorithm", "refnum"=w836) -> ("error out"=w832:errorcluster, "value"=w830:string, "refnum out"=w831:T12)  [unwired: 1 in, 3 out]
          n307 = Decimal String To Number(string=w830) -> (number=w828:i32)  [unwired: 2 in, 1 out]
          n308 = Less Or Equal To 0?(x=w828) -> (x <= 0?=w829:bool)
          n309 = Select(t=10, s=w829, f=w828) -> (s? t:f=w827:i32)
          n310 = call <vilib>:"Close Config Data.vi"("error in (no error)"=w832, "refnum"=w831) -> ()  [unwired: 8 in, 2 out]
          n311 = control-ref of="Pannel User Message"() -> (w848:refnum<vi>)
          n312 = control-ref of="Motor Speed RPM"() -> (w846:refnum<vi>)
          n313 = control-ref of="Stop Button"() -> (w850:refnum<vi>)
          n314 = control-ref of="ATR"() -> (w849:refnum<vi>)
          n315 = control-ref of="Config_CANAT"() -> (w847:refnum<vi>)
          n316 = control-ref of="UUT"() -> (w845:refnum<vi>)
          n317 = control-ref of="Stop Burn-in"() -> (w844:refnum<vi>)
          n318 = call "Table_ScrollaBarMarvin.vi"("error in"=w853, "Line to focus"=w841, "reference in"=w855) -> ("error out"=w852:errorcluster)  [unwired: 2 out]
          n319 = call "Reset old test Values (SubVI).vi"("error in"=w852, "Atr in"=w855, "Test Paragraph"=w841) -> ("error out"=w842:errorcluster)  [unwired: 8 in]
          n320 = while {
            tunnel: w842 -> [w868]
            shift-right: [w866] -> _
            shift-left: enum16{"Stop", "Algorithm", "Start"}."Start" -> [w867]
            tunnel: w850 -> [w865]
            tunnel: w849 -> [w864]
            tunnel: w848 -> [w863]
            tunnel: w847 -> [w862]
            tunnel: w846 -> [w861]
            tunnel: w845 -> [w860]
            tunnel: w844 -> [w858]
            tunnel: w843 -> [w857]
            tunnel: w827 -> [w856]
            stop <- w859 stop-if-true
            n321 = case shown="\"Algorithm\"" w867 {
              tunnel: w868 -> [_ _ w1005]
              tunnel: [w869 w890 w994] -> w866
              tunnel: w865 -> [_ w901 w998]
              tunnel: w864 -> [_ w897 _]
              tunnel: w863 -> [_ w902 _]
              tunnel: w862 -> [w872 _ w979]
              tunnel: w861 -> [_ w898 _]
              tunnel: w860 -> [w871 _ w978]
              tunnel: [w870 FALSE FALSE] -> w859
              tunnel: w858 -> [_ w900 _]
              tunnel: w857 -> [_ w899 _]
              tunnel: w856 -> [_ w884 _]
              frame "Stop", Default {
                n322 = flat-sequence {
                  tunnel: w872 -> [w877]
                  tunnel: w871 -> [w875]
                  tunnel: [TRUE] -> w870
                  tunnel: [enum16{"Stop", "Algorithm", "Start"}."Stop"] -> w869
                  frame #0 {
                    n323 = call "CANSendMotorSpeed.vi"("Remote"=TRUE, "Motor Speed RPM"=u16 0, "UUT"=w875, "CAN Cluster in"=w877) -> ("error out"=w873:errorcluster)  [unwired: 7 in]
                    n324 = property on="VISA Tester" class="VISAName"() -> ("Value"=w881:refnum<visa-resource-name>)  [unwired: 2 in, 2 out]
                    n325 = call "TesterOption (SubVI).vi"("2 Options"=FALSE, "error in (no error)"=w873, "On/Off"=FALSE, "Tester Option"=T13."Venable", "VISA Refnum in"=w881) -> ()  [unwired: 5 in, 2 out]
                  }
                  frame #1 {
                  }
                  frame #2 {
                  }
                }
              }
              frame "Algorithm" {
                w885 = T20 [enum."6000", enum."11500", enum."15100", enum."11500-2", enum."6000-2"] items=["6000", "11500", "15100", "11500-2", "6000-2"]
                # "Speed Goal"
                # "Speed Ind"
                # "Temp Goal"
                # "50 Deg"
                n326 = for {
                  tunnel: w902 -> [w930]
                  tunnel: w901 -> [w929]
                  tunnel: w900 -> [w928]
                  tunnel: w899 -> [w927]
                  tunnel: w898 -> [w926]
                  tunnel: w897 -> [w913]
                  tunnel: string[] ["Tair <   67 ± 3 °C", "Tair >= 67 ± 3 °C", "Tair >= 83 ± 3 °C", "Tair <= 80 ± 3 °C", "Tair <= 64 ± 3 °C"] -> [w911] mode=indexing
                  shift-right: [w923] -> _
                  shift-left: 1202.0 ("Rt") -> [w924]
                  tunnel: dbl[] [67.0, 67.0, 83.0, 80.0, 64.0] -> [w922] mode=indexing
                  tunnel: dbl[] [11500.0, 12700.0, 14700.0, 12700.0, 11500.0] -> [w921] mode=indexing
                  tunnel: dbl[] [11500.0, 11900.0, 13000.0, 13900.0, 12200.0] -> [w920] mode=indexing
                  tunnel: [w909] -> w891
                  tunnel: [w908] -> w887 mode=indexing
                  tunnel: [w907] -> w888 mode=indexing
                  tunnel: w885 -> [w906] mode=indexing
                  tunnel: w884 -> [w905]
                  stop <- w925 stop-if-true
                  n327 = call <vilib>:"High Resolution Relative Seconds.vi"() -> ("relative seconds"=w919:dbl)
                  n328 = while {
                    tunnel: w930 -> [w959]
                    tunnel: w929 -> [w951]
                    tunnel: w928 -> [w958]
                    tunnel: w927 -> [w937]
                    tunnel: w926 -> [w960]
                    shift-right: [w956] -> w923
                    shift-left: w924 -> [w955]
                    tunnel: w906 -> [w957]
                    tunnel: w922 -> [w954]
                    tunnel: w921 -> [w953]
                    tunnel: w920 -> [w952]
                    tunnel: w919 -> [w948]
                    tunnel: [w943] -> w914
                    tunnel: [w942] -> w907
                    tunnel: [w941] -> w912
                    tunnel: [w940] -> w908
                    tunnel: [w939] -> w910
                    tunnel: w905 -> [w931]
                    stop <- w949 stop-if-true
                    n329 = call "DegToDAC (SubVI).vi"("R2"=0.0, "Rt"=w955) -> ("error out"=w967:errorcluster, "output array"=w968:u8[])  [unwired: 8 in]
                    n330 = call <vilib>:"High Resolution Relative Seconds.vi"() -> ("relative seconds"=w947:dbl)
                    n331 = property on="VISA Tester" class="VISAName"() -> ("Value"=w970:refnum<visa-resource-name>)  [unwired: 2 in, 2 out]
                    n332 = Byte Array To String(unsigned byte array=w968) -> (string=w969:string)
                    n333 = Subtract(x=w948, y=w947) -> (x-y=w946:dbl)
                    n334 = VISA Write(VISA resource name=w970, write buffer=w969, error in (no error)=w967) -> (error out=w966:errorcluster)  [unwired: 2 out]
                    n335 = Greater Or Equal?(x=w946, y=120.0) -> (x >= y?=w944:bool)
                    n336 = call <vilib>:"Clear Errors.vi"("error in (no error)"=w966) -> ("error out"=w965:errorcluster)  [unwired: 5 in, 1 out]
                    n337 = control-ref of="Ambient Temperature"() -> (w938:refnum<vi>)
                    n338 = property class="DigNum (strict)"(reference=w938) -> ("Value"=w936:dbl)  [unwired: 1 in, 2 out]
                    n339 = property class="Bool (strict)"(reference=w951) -> ("Value"=w950:bool)  [unwired: 1 in, 2 out]
                    n340 = Number To Fractional String(number=w936, precision (6)=i16 2) -> (F-format string=w933:string)  [unwired: 2 in]
                    n341 = Concatenate Strings(w937, "\nAmbient  Temp. [C]: " ("string"), w933) -> (w932:string)
                    n342 = call "Write panel message (SubVI).vi"("Stop BurnIn"=w958, 4:"rpm"=w960, 5:"rpm"=TRUE ("rpm"), "PrintTime"=TRUE, "Stop"=w951, "error in (no error)"=w965, "Time to wait"=5.0, "Strin"=w932, "String in"=w959) -> ("error out"=w964:errorcluster)  [unwired: 2 in]
                    n343 = call "TempAlgoTest (SubVI).vi"("Temp"=w938, "Speed Ind"=w952, "Motor Speed RPM"=w960, "Round"=w957, "Temp Up In"=w955, "error in (no error)"=w964, "String in"=w959, "Temp Goal"=w954, "Stop"=w951, "Speed Goal"=w953, "Stop BurnIn"=w958, "AD Resistor Step"=w931, "Strin"=w932) -> (14:"Speed Pass/Fail"=w942:bool, "Temp  Pass/Fail"=w941:dbl, "Temp Up Out"=w956:dbl, 17:"Speed Pass/Fail"=w943:dbl, "Temp Pass/Fail"=w940:bool, "error out"=w939:errorcluster)  [unwired: 1 in]
                    n344 = Compound Arithmetic op=OR(w944, w942, w950) -> (w949:bool)
                  }
                  n345 = property class="Bool (strict)"(reference=w929) -> ("Value"=w925:bool)  [unwired: 1 in, 2 out]
                  n346 = call "Find_Number_LineMARVIN.vi"("Test Paragraph"=w911, "error in"=w910, "TableIn"=w913) -> ("error out"=w915:errorcluster, "Line number"=w918:i32)  [unwired: 2 in, 2 out]
                  n347 = Increment(x=w918) -> (x+1=w917:i32)
                  n348 = call "PassOrFail (SubVI).vi"("index (row)"=w917, "error in (no error)"=w915, "Data in"=w912, "Pass?Fail"=w908, "Table in"=w913) -> ("error out"=w916:errorcluster)  [unwired: 6 in]
                  n349 = call "PassOrFail (SubVI).vi"("index (row)"=w918, "error in (no error)"=w916, "Data in"=w914, "Pass?Fail"=w907, "Table in"=w913) -> ("error out"=w909:errorcluster)  [unwired: 6 in]
                }
                n350 = Build Array (concatenate)(w888, w887) -> (w889:bool[])
                n351 = flat-sequence {
                  tunnel: w891 -> [_]
                  tunnel: [enum16{"Stop", "Algorithm", "Start"}."Stop"] -> w890
                  frame #0 {
                  }
                }
                n352 = And Array Elements(Boolean array=w889) -> (logical AND=→"TempControlResult":bool)
              }
              frame "Start" {
                n353 = call <vilib>:"Clear Errors.vi"("error in (no error)"=w1005) -> ("error out"=w980:errorcluster)  [unwired: 5 in, 1 out]
                n354 = call "CANSendMotorSpeed.vi"("Remote"=TRUE, "error in (no error)"=w980, "Motor Speed RPM"=u16 0, "UUT"=w978, "CAN Cluster in"=w979) -> ("error out"=w975:errorcluster)  [unwired: 6 in]
                n355 = call "Time Delay15"("error in (no error)"=w975) -> ("error out"=w974:errorcluster)  [unwired: 10 in]
                n356 = call "DegToDAC (SubVI).vi"("error in (no error)"=w974, "R2"=0.0, "Rt"=1202.0) -> ("error out"=w985:errorcluster, "output array"=w986:u8[])  [unwired: 7 in]
                n357 = property on="VISA Tester" class="VISAName"() -> ("Value"=w988:refnum<visa-resource-name>)  [unwired: 2 in, 2 out]
                n358 = Byte Array To String(unsigned byte array=w986) -> (string=w987:string)
                n359 = VISA Write(VISA resource name=w988, write buffer=w987, error in (no error)=w985) -> (error out=w977:errorcluster)  [unwired: 2 out]
                n360 = call "Time Delay16"("error in (no error)"=w977) -> ("error out"=w976:errorcluster)  [unwired: 10 in]
                n361 = property on="VISA Tester" class="VISAName"() -> ("Value"=w1004:refnum<visa-resource-name>)  [unwired: 2 in, 2 out]
                n362 = call "TesterOption (SubVI).vi"("On/Off 2"=TRUE, "Tester Option 2"=T13."Venable", "2 Options"=TRUE, "error in (no error)"=w976, "On/Off"=TRUE, "Tester Option"=T13."K16", "VISA Refnum in"=w1004) -> ("error out"=w990:errorcluster)  [unwired: 3 in, 1 out]
                n363 = call "Time Delay12"("error in (no error)"=w990) -> ("error out"=w989:errorcluster)  [unwired: 10 in]
                n364 = call "CANSendMotorSpeed.vi"("Remote"=FALSE, "error in (no error)"=w989, "Motor Speed RPM"=u16 0, "UUT"=w978, "CAN Cluster in"=w979) -> ("error out"=w973:errorcluster)  [unwired: 6 in]
                n365 = call "Time Delay17"("error in (no error)"=w973) -> ("error out"=w972:errorcluster)  [unwired: 10 in]
                n366 = property class="Bool (strict)"(reference=w998, error in=w972) -> ("Value"=w997:bool)  [unwired: 2 out]
                n367 = Select(t=enum16{"Stop", "Algorithm", "Start"}."Stop", s=w997, f=enum16{"Stop", "Algorithm", "Start"}."Algorithm") -> (s? t:f=w994:enum16{"Stop", "Algorithm", "Start"})
              }
            }
          }
        }
        frame "Burn in" {
          n368 = control-ref of="Stop Button"() -> (w1011:refnum<vi>)
          n369 = control-ref of="Pannel User Message"() -> (w1014:refnum<vi>)
          n370 = control-ref of="ATR"() -> (w1010:refnum<vi>)
          n371 = control-ref of="Config_CANAT"() -> (w1013:refnum<vi>)
          n372 = control-ref of="UUT"() -> (w1012:refnum<vi>)
          n373 = control-ref of="Stop Burn-in"() -> (w1009:refnum<vi>)
          n374 = property on="UUT" class="DigNum (strict)"() -> ("Value"=w1008:u8)  [unwired: 2 in, 2 out]
          n375 = while {
            tunnel: w1014 -> [w1028]
            tunnel: w1010 -> [w1027]
            tunnel: w1013 -> [w1026]
            tunnel: w1012 -> [w1025]
            tunnel: w1011 -> [w1024]
            shift-right: [w1023] -> _
            shift-left: T17."Start" -> [w1030]
            shift-right: [w1029] -> _
            shift-left: _ -> [w1021]
            tunnel: w1009 -> [w1020]
            tunnel: w1008 -> [w1019]
            tunnel: w1007 -> [w1018]
            shift-right: [w1017] -> _
            shift-left: FALSE -> [w1016]
            stop <- w1022 stop-if-true
            n376 = case shown="\"DC Current Measure\"" w1030 {
              tunnel: [w1036 w1072 w1140 w1167 w1197 w1231] -> w1029
              tunnel: w1028 -> [_ w1064 _ _ _ w1230]
              tunnel: w1027 -> [_ w1067 w1113 w1154 w1183 w1217]
              tunnel: w1026 -> [w1032 w1063 _ _ _ w1229]
              tunnel: w1025 -> [w1031 w1060 _ _ _ w1210]
              tunnel: w1024 -> [_ _ w1142 w1169 w1201 w1223]
              tunnel: [w1034 T17."Stop" w1143 w1170 w1202 w1219] -> w1023
              tunnel: [w1035 FALSE FALSE FALSE FALSE FALSE] -> w1022
              tunnel: w1021 -> [w1036 w1072 w1140 w1167 w1197 _]
              tunnel: w1020 -> [_ _ _ _ _ w1213]
              tunnel: w1019 -> [_ w1056 w1107 w1149 w1178 w1209]
              tunnel: w1018 -> [_ w1052 _ _ _ _]
              tunnel: [FALSE ("Stop Burn-in") w1051 FALSE w1147 w1175 FALSE ("Stop Burn-in")] -> w1017
              tunnel: w1016 -> [_ _ w1102 _ _ _]
              frame "Stop", Default {
                n377 = flat-sequence {
                  tunnel: w1032 -> [w1039]
                  tunnel: w1031 -> [w1038]
                  tunnel: [TRUE] -> w1035
                  tunnel: [T17."Stop"] -> w1034
                  frame #0 {
                    w1037 = u16 0 ("Motor Speed RPM")
                    n378 = call "CANSendMotorSpeed.vi"("Remote"=TRUE, "Motor Speed RPM"=w1037, "UUT"=w1038, "CAN Cluster in"=w1039) -> ("error out"=w1041:errorcluster)  [unwired: 7 in]
                    n379 = property on="BurnInSpeed" class="DigNum (strict)"("Value"=w1037) -> ()  [unwired: 2 in, 2 out]
                    n380 = property on="VISA Tester" class="VISAName"() -> ("Value"=w1046:refnum<visa-resource-name>)  [unwired: 2 in, 2 out]
                    n381 = call "TesterOption (SubVI).vi"("2 Options"=FALSE, "error in (no error)"=w1041, "On/Off"=FALSE, "Tester Option"=T13."Venable", "VISA Refnum in"=w1046) -> ("error out"=w1043:errorcluster)  [unwired: 5 in, 1 out]
                    n382 = property on="Stop Burn-in" class="Bool (strict)"(error in=w1043, "Visible"=FALSE) -> ()  [unwired: 1 in, 2 out]
                  }
                  frame #1 {
                  }
                }
              }
              frame "BurnIn" {
                w1051 = FALSE ("Stop Burn-in")
                n383 = control-ref of="Motor Speed RPM"() -> (w1066:refnum<vi>)
                n384 = control-ref of="Stop Button"() -> (w1065:refnum<vi>)
                n385 = property on="Stop Burn-in" class="Bool (strict)"("Visible"=w1052) -> (error out=w1068:errorcluster)  [unwired: 2 in, 1 out]
                n386 = Equal?(x=w1056, y=u8 95) -> (x = y?=w1055:bool)
                n387 = call "Find_Number_LineMARVIN.vi"("Test Paragraph"="After 10 min of operation", "error in"=w1068, "TableIn"=w1067) -> ("error out"=w1070:errorcluster, "Line number"=w1071:i32)  [unwired: 2 in, 2 out]
                n388 = Select(t=u16 14700, s=w1055, f=u16 12100 ("y")) -> (s? t:f=w1058:u16)
                n389 = for {
                  tunnel: w1070 -> [w1089]
                  tunnel: dbl[] [600.0, 600.0, 600.0] -> [w1093] mode=indexing
                  tunnel: w1071 -> [w1098]
                  tunnel: w1067 -> [w1088]
                  tunnel: w1066 -> [w1087]
                  tunnel: w1065 -> [w1086]
                  tunnel: w1064 -> [w1085]
                  tunnel: w1063 -> [w1081]
                  tunnel: w1060 -> [w1080]
                  tunnel: w1058 -> [w1076]
                  tunnel: [w1078] -> w1057
                  tunnel: [w1077] -> w1054 mode=indexing
                  i -> [w1095]
                  n390 = call "CANSendMotorSpeed.vi"("Remote"=TRUE, "error in (no error)"=w1089, "Motor Speed RPM"=w1076, "UUT"=w1080, "CAN Cluster in"=w1081) -> ("error out"=w1083:errorcluster)  [unwired: 6 in]
                  n391 = control-ref of="Stop Burn-in"() -> (w1084:refnum<vi>)
                  n392 = Add(x=w1098, y=w1095) -> (x+y=w1094:i32)
                  n393 = call "Write panel message (SubVI).vi"("Stop BurnIn"=w1084, 4:"rpm"=w1087, 5:"rpm"=TRUE ("rpm"), "PrintTime"=TRUE, "Stop"=w1086, "error in (no error)"=w1083, "Time to wait"=w1093, "Strin"="Burn-in test in process...", "String in"=w1085) -> ("error out"=w1090:errorcluster)  [unwired: 2 in]
                  n394 = control-ref of="Power transistor Heat sink Temp."() -> (w1099:refnum<vi>)
                  n395 = property on="MaxBurnInTempVal" class="DigNum (strict)"() -> ("Value"=w1097:dbl)  [unwired: 2 in, 2 out]
                  n396 = property class="DigNum (strict)"(reference=w1099, error in=w1090) -> (error out=w1079:errorcluster, "Value"=w1096:dbl)  [unwired: 1 out]
                  n397 = property on="BurnInSpeed" class="DigNum (strict)"("Value"=w1076) -> ()  [unwired: 2 in, 2 out]
                  n398 = Less Or Equal?(x=w1096, y=w1097) -> (x <= y?=w1077:bool)
                  n399 = call "PassOrFail (SubVI).vi"("index (row)"=w1094, "error in (no error)"=w1079, "Data in"=w1096, "Pass?Fail"=w1077, "Table in"=w1088) -> ("error out"=w1078:errorcluster)  [unwired: 6 in]
                }
                n400 = And Array Elements(Boolean array=w1054) -> (logical AND=→"BurnResult":bool)
                n401 = property on="Stop Burn-in" class="Bool (strict)"(error in=w1057, "Value"=w1051, "Visible"=w1051) -> ()  [unwired: 1 in, 2 out]
              }
              frame "Ambient Temp" {
                w1118 = 2 ("disabled index (col)")
                n402 = control-ref of="Power transistor Heat sink Temp."() -> (w1128:refnum<vi>)
                n403 = call "Find_Number_LineMARVIN.vi"("Test Paragraph"="Ambient Temperature", "TableIn"=w1113) -> ("error out"=w1139:errorcluster, "Line number"=w1119:i32)  [unwired: 3 in, 2 out]
                n404 = Equal?(x=w1107, y=u8 95) -> (x = y?=w1108:bool)
                n405 = property class="DigNum (strict)"(reference=w1128, error in=w1139) -> (error out=w1130:errorcluster, "Value"=w1120:dbl)  [unwired: 1 out]
                n406 = Select(t=25.0 ("y"), s=w1108, f=25.0 ("y")) -> (s? t:f=w1129:dbl)
                n407 = Select(t=13.0 ("y"), s=w1108, f=13.0) -> (s? t:f=w1131:dbl)
                n408 = Add(x=w1129, y=w1131) -> (x+y=w1138:dbl)
                n409 = Subtract(x=w1129, y=w1131) -> (x-y=w1137:dbl)
                n410 = In Range and Coerce(upper limit=w1138, x=w1120, lower limit=w1137) -> (In Range?=w1104:bool)  [unwired: 1 out]
                "BurnTemp" <- w1104
                n411 = call "PassOrFail (SubVI).vi"("index (row)"=w1119, "error in (no error)"=w1130, "Data in"=w1120, "Pass?Fail"=w1104, "Table in"=w1113) -> ("error out"=w1110:errorcluster)  [unwired: 6 in]
                n412 = property class="Tbl (strict)"(reference=w1113, error in=w1110) -> (reference out=w1112:refnum<vi>, error out=w1127:errorcluster, "Value"=w1126:string[][])
                n413 = Add(x=w1120, y=25.0) -> (x+y=w1111:dbl)
                "MaxBurnInTempVal" <- w1111
                n414 = Number To Fractional String(number=w1111, precision (6)=i16 0) -> (F-format string=w1125:string)  [unwired: 2 in]
                n415 = Concatenate Strings("< " ("string"), w1125) -> (w1114:string)
                n416 = Increment(x=w1119) -> (x+1=w1117:i32)
                n417 = Increment(x=w1117) -> (x+1=w1116:i32)
                n418 = Increment(x=w1116) -> (x+1=w1115:i32)
                n419 = Replace Array Subset(array=w1126, new element #1=w1114, index (row) #1=w1117, index (col) #1=w1118, new element #2=w1114, index (row) #2=w1116, index (col) #2=w1118, new element #3=w1114, index (row) #3=w1115, index (col) #3=w1118) -> (w1124:string[][])
                n420 = Not(x=w1104) -> (.not. x?=w1103:bool)
                n421 = property class="Tbl (strict)"(reference=w1112, error in=w1127, "Value"=w1124) -> (error out=w1109:errorcluster)  [unwired: 1 out]
                n422 = property class="Bool (strict)"(reference=w1142, error in=w1109) -> ("Value"=w1105:bool)  [unwired: 2 out]
                n423 = Compound Arithmetic op=OR(w1103, w1102, w1105) -> (w1106:bool)
                n424 = Select(t=T17."Stop", s=w1106, f=T17."BurnIn") -> (s? t:f=w1143:T17)
              }
              frame "MotorSpeed" {
                n425 = control-ref of="Motor Speed RPM"() -> (w1152:refnum<vi>)
                n426 = Equal?(x=w1149, y=u8 95) -> (x = y?=w1150:bool)
                n427 = call "Find_Number_LineMARVIN.vi"("Test Paragraph"="Fan speed", "TableIn"=w1154) -> ("error out"=w1166:errorcluster, "Line number"=w1157:i32)  [unwired: 3 in, 2 out]
                n428 = property class="DigNum (strict)"(reference=w1152, error in=w1166) -> (error out=w1155:errorcluster, "Value"=w1156:dbl)  [unwired: 1 out]
                n429 = Select(t=14700.0 ("y"), s=w1150, f=12100.0 ("y")) -> (s? t:f=w1153:dbl)
                n430 = Select(t=200.0 ("y"), s=w1150, f=200.0) -> (s? t:f=w1158:dbl)
                n431 = Add(x=w1153, y=w1158) -> (x+y=w1165:dbl)
                n432 = Subtract(x=w1153, y=w1158) -> (x-y=w1164:dbl)
                n433 = In Range and Coerce(upper limit=w1165, x=w1156, lower limit=w1164) -> (In Range?=w1148:bool)  [unwired: 1 out]
                "BurnSpeed" <- w1148
                n434 = call "PassOrFail (SubVI).vi"("index (row)"=w1157, "error in (no error)"=w1155, "Data in"=w1156, "Pass?Fail"=w1148, "Table in"=w1154) -> ("error out"=w1151:errorcluster)  [unwired: 6 in]
                n435 = property class="Bool (strict)"(reference=w1169, error in=w1151) -> ("Value"=w1173:bool)  [unwired: 2 out]
                n436 = Select(t=T17."Stop", s=w1173, f=T17."Ambient Temp") -> (s? t:f=w1170:T17)
                n437 = Not(x=w1148) -> (.not. x?=w1147:bool)
              }
              frame "DC Current Measure" {
                n438 = property on="VISA Tester" class="VISAName"() -> (error out=w1195:errorcluster, "Value"=w1199:refnum<visa-resource-name>)  [unwired: 2 in, 1 out]
                n439 = call "GetADCTester (SubVI).vi"("error in (no error)"=w1195, "GetADCTester"=T15."Current", "TimeToGet"=10, "VISA Refnum in"=w1199) -> ("error out"=w1196:errorcluster, "ADCValOutput Single"=w1182:dbl)  [unwired: 5 in, 1 out]
                n440 = Equal?(x=w1178, y=u8 95) -> (x = y?=w1179:bool)
                n441 = call "Find_Number_LineMARVIN.vi"("Test Paragraph"="DC Input Current", "error in"=w1196, "TableIn"=w1183) -> ("error out"=w1194:errorcluster, "Line number"=w1184:i32)  [unwired: 2 in, 2 out]
                n442 = Select(t=45.0 ("y"), s=w1179, f=28.0 ("y")) -> (s? t:f=w1186:dbl)
                n443 = Select(t=5.0 ("y"), s=w1179, f=3.0) -> (s? t:f=w1185:dbl)
                n444 = Add(x=w1186, y=w1185) -> (x+y=w1193:dbl)
                n445 = Subtract(x=w1186, y=w1185) -> (x-y=w1192:dbl)
                n446 = In Range and Coerce(upper limit=w1193, x=w1182, lower limit=w1192) -> (In Range?=w1177:bool)  [unwired: 1 out]
                "BurnDC" <- w1177
                n447 = call "PassOrFail (SubVI).vi"("index (row)"=w1184, "error in (no error)"=w1194, "Data in"=w1182, "Pass?Fail"=w1177, "Table in"=w1183) -> ("error out"=w1181:errorcluster)  [unwired: 6 in]
                n448 = property class="Bool (strict)"(reference=w1201, error in=w1181) -> ("Value"=w1176:bool)  [unwired: 2 out]
                n449 = Not(x=w1177) -> (.not. x?=w1175:bool)
                n450 = Select(t=T17."Stop", s=w1176, f=T17."MotorSpeed") -> (s? t:f=w1202:T17)
              }
              frame "Start" {
                w1205 = "Burn-in Test" ("Line to focus")
                w1207 = "Burn-in test in process...\nFull Speed Operation" ("Value")
                n451 = Equal?(x=w1209, y=u8 95) -> (x = y?=w1211:bool)
                n452 = property class="Str"(reference=w1230, "Value"=w1207) -> (reference out=w1227:refnum<vi>, error out=w1212:errorcluster)  [unwired: 1 in]
                n453 = call "Find_Number_LineMARVIN.vi"("Test Paragraph"=w1205, "error in"=w1212, "TableIn"=w1217) -> ("error out"=w1237:errorcluster, "Line number"=w1238:i32)  [unwired: 2 in, 2 out]
                n454 = Select(t=u16 14700 ("y"), s=w1211, f=u16 12100 ("y")) -> (s? t:f=w1244:u16)
                "BurnInSpeed" <- w1244
                n455 = call "Table_ScrollaBarMarvin.vi"("error in"=w1237, "Line to focus"=w1205, "reference in"=w1217) -> ("error out"=w1239:errorcluster)  [unwired: 2 out]
                n456 = call "Reset old test Values (SubVI).vi"("error in"=w1239, "Atr in"=w1217, "Test Paragraph"=w1205) -> ("error out"=w1240:errorcluster)  [unwired: 8 in]
                n457 = Increment(x=w1238) -> (x+1=w1231:i32)
                n458 = property on="VISA Tester" class="VISAName"(error in=w1240) -> (error out=w1241:errorcluster, "Value"=w1242:refnum<visa-resource-name>)  [unwired: 1 in, 1 out]
                n459 = call "TesterOption (SubVI).vi"("2 Options"=FALSE, "error in (no error)"=w1241, "On/Off"=TRUE, "Tester Option"=T13."Venable", "VISA Refnum in"=w1242) -> ("error out"=w1243:errorcluster)  [unwired: 5 in, 1 out]
                n460 = call "CANSendMotorSpeed.vi"("Remote"=TRUE, "error in (no error)"=w1243, "Motor Speed RPM"=w1244, "UUT"=w1210, "CAN Cluster in"=w1229) -> ("error out"=w1228:errorcluster)  [unwired: 6 in]
                n461 = control-ref of="Motor Speed RPM"() -> (w1216:refnum<vi>)
                n462 = call "Write panel message (SubVI).vi"("Stop BurnIn"=w1213, 4:"rpm"=w1216, 5:"rpm"=TRUE ("rpm"), "PrintTime"=TRUE, "Stop"=w1223, "error in (no error)"=w1228, "Time to wait"=50.0, "Strin"=w1207, "String in"=w1227) -> ("error out"=w1215:errorcluster)  [unwired: 2 in]
                n463 = property class="Bool (strict)"(reference=w1223, error in=w1215) -> ("Value"=w1222:bool)  [unwired: 2 out]
                n464 = Select(t=T17."Stop", s=w1222, f=T17."DC Current Measure") -> (s? t:f=w1219:T17)
              }
            }
          }
        }
        frame "Visual Inspec" {
          n465 = control-ref of="Stop Button"() -> (w1248:refnum<vi>)
          n466 = property class="Bool (strict)"(reference=w1248, error in=w1247) -> (error out=w1246:errorcluster, "Value"=w1245:bool)  [unwired: 1 out]
          n467 = case shown="False" w1245 {
            tunnel: w1249 -> [w1263 _]
            tunnel: w1246 -> [w1250 _]
            frame False {
              n468 = property on="VISA Tester" class="VISAName"() -> ("Value"=w1262:refnum<visa-resource-name>)  [unwired: 2 in, 2 out]
              n469 = call "TesterOption (SubVI).vi"("2 Options"=FALSE, "error in (no error)"=w1250, "On/Off"=FALSE, "Tester Option"=T13."Venable", "VISA Refnum in"=w1262) -> ("error out"=w1258:errorcluster)  [unwired: 5 in, 1 out]
              n470 = local read "UUT"() -> (w1254:u8)
              n471 = Equal?(x=w1254, y=u8 95) -> (x = y?=w1255:bool)
              n472 = case shown="True" w1255 {
                tunnel: w1263 -> [w1267 w1277]
                tunnel: w1258 -> [w1266 w1276]
                tunnel: [w1268 w1279] -> w1257
                tunnel: [w1269 w1278] -> w1253
                tunnel: string[] ["Verification of Components Not Installed", "Manufacturing Defects", "DC Input Current Drawn", "12V", "5V", "3.3V", "1.8V", "Reverse Polarity Test - DC Input Current", "Weight Check", "J3.B to Chassis", "J1.16 to Chassis", "J1 Body to Chassis", "J2  Body to Chassis", "J3  Body to Chassis", "J1.17 to J1.18", "Sealing Test", "Mounting Holes Test - Jig Fit"] ("deleted portion 3") -> [w1264 w1274]
                frame False {
                  # "AHU"
                  n473 = for {
                    tunnel: w1264 -> [w1273] mode=indexing
                    tunnel: w1267 -> [w1272]
                    tunnel: w1266 -> [w1271]
                    tunnel: [w1270] -> w1265
                    n474 = call "Reset old test Values (SubVI).vi"("error in"=w1271, "Atr in"=w1272, "Test Paragraph"=w1273) -> ("error out"=w1270:errorcluster)  [unwired: 8 in]
                  }
                  n475 = call "VisualInspectionAHUold.vi"("error in (no error)"=w1265, "TableRef"=w1267) -> ("error out"=w1269:errorcluster, "VisualInspectionResult"=w1268:bool)  [unwired: 8 in]
                }
                frame True {
                  # "EBAY"
                  n476 = for {
                    tunnel: w1277 -> [w1283]
                    tunnel: w1276 -> [w1282]
                    tunnel: [w1281] -> w1275
                    tunnel: w1274 -> [w1280] mode=indexing
                    n477 = call "Reset old test Values (SubVI).vi"("error in"=w1282, "Atr in"=w1283, "Test Paragraph"=w1280) -> ("error out"=w1281:errorcluster)  [unwired: 8 in]
                  }
                  n478 = call "VisualInspectionEBAYold.vi"("error in (no error)"=w1275, "TableRef"=w1277) -> ("error out"=w1278:errorcluster, "VisualInspectionResult"=w1279:bool)  [unwired: 8 in]
                }
              }
              "VisualInspectionResult" <- w1257
              n479 = property on="Automation" class="Bool (strict)"(error in=w1253) -> ("Value"=w1252:bool)  [unwired: 1 in, 2 out]
              n480 = case shown="True" w1252 {
                frame False {
                }
                frame True {
                  w1284 = TRUE ("Value (Signaling)")
                  n481 = property on="SetSN" class="Bool (strict)"("Val(Sgnl)"=w1284, "Value"=w1284) -> ()  [unwired: 2 in, 2 out]
                }
              }
            }
            frame True {
            }
          }
        }
        frame "Temp Sens Cal" {
          w1288 = "Temperature sensor calibration test in process..." ("Value")
          w1286 = "Temperature Sensor Calibration" ("Test Paragraph")
          n482 = control-ref of="Pannel User Message"() -> (w1295:refnum<vi>)
          n483 = property class="Str"(reference=w1295, error in=w1294, "Value"=w1288) -> (error out=w1293:errorcluster)  [unwired: 1 out]
          n484 = call "Table_ScrollaBarMarvin.vi"("error in"=w1293, "Line to focus"=w1286, "reference in"=w1296) -> ("error out"=w1298:errorcluster)  [unwired: 2 out]
          n485 = property class="Tbl (strict)"(reference=w1296, error in=w1298) -> (reference out=w1285:refnum<vi>, error out=w1300:errorcluster, "Value"=w1301:string[][])
          n486 = Index Array(array=w1301, index (col)=1 ("disabled index (col)")) -> (element=w1302:string[])  [unwired: 1 in]
          n487 = call "Find_Number_Line.vi"("error in"=w1300, "Test Paragraph"=w1286, "Row Headers[]"=w1302) -> ("error out"=w1297:errorcluster, "Line number"=w1290:i32)  [unwired: 1 out]
          n488 = property on="Status" class="Bool (strict)"(error in=w1297) -> (error out=w1291:errorcluster, "Value"=w1292:bool)  [unwired: 1 in, 1 out]
          n489 = call "Reset old test Values (SubVI).vi"("error in"=w1291, "Atr in"=w1285, "Test Paragraph"=w1286) -> ("error out"=w1287:errorcluster)  [unwired: 8 in]
          n490 = case shown="True" w1292 {
            selector: w1292 -> [w1306 _]
            tunnel: w1287 -> [w1308 _]
            tunnel: w1285 -> [w1305 _]
            tunnel: w1290 -> [w1304 _]
            tunnel: w1289 -> [_ w1315]
            tunnel: w1288 -> [_ w1311]
            frame False {
              n491 = flat-sequence {
                tunnel: w1308 -> [w1309]
                tunnel: [w1309] -> w1307
                frame #0 {
                  n492 = One Button Dialog(message="Please establish RS connection.") -> ()  [unwired: 1 in, 1 out]
                }
              }
              n493 = Increment(x=w1304) -> (x+1=w1303:i32)
              n494 = call "PassOrFail (SubVI).vi"("index (row)"=w1303, "error in (no error)"=w1307, "Pass?Fail"=w1306, "Table in"=w1305) -> ()  [unwired: 7 in, 1 out]
            }
            frame True {
              n495 = control-ref of="Stop Burn-in"() -> (w1317:refnum<vi>)
              n496 = control-ref of="Pannel User Message"() -> (w1319:refnum<vi>)
              n497 = control-ref of="Config_CANAT"() -> (w1313:refnum<vi>)
              n498 = control-ref of="ATR"() -> (w1320:refnum<vi>)
              n499 = control-ref of="Motor Speed RPM"() -> (w1321:refnum<vi>)
              n500 = control-ref of="UUT"() -> (w1312:refnum<vi>)
              n501 = control-ref of="Stop Button"() -> (w1318:refnum<vi>)
              n502 = property on="VISA Tester" class="VISAName"() -> ("Value"=w1314:refnum<visa-resource-name>)  [unwired: 2 in, 2 out]
              n503 = while {
                shift-right: [w1324] -> _
                shift-left: T16."Start" -> [w1334]
                tunnel: w1317 -> [w1333]
                tunnel: w1318 -> [w1332]
                tunnel: w1319 -> [w1331]
                tunnel: w1320 -> [w1330]
                tunnel: w1321 -> [w1329]
                tunnel: w1315 -> [w1328]
                tunnel: w1314 -> [w1327]
                tunnel: w1313 -> [w1326]
                tunnel: w1312 -> [w1325]
                tunnel: w1311 -> [w1322]
                stop <- w1323 stop-if-true
                n504 = case shown="\"Stop\", Default" w1334 {
                  tunnel: w1333 -> [_ w1369 w1396 w1451 w1481]
                  tunnel: w1332 -> [_ w1370 w1388 w1437 w1483]
                  tunnel: w1331 -> [_ w1367 w1397 w1449 w1485]
                  tunnel: w1330 -> [_ w1347 _ _ _]
                  tunnel: w1329 -> [_ w1371 w1395 w1452 w1480]
                  tunnel: w1328 -> [_ w1380 w1400 w1461 w1477]
                  tunnel: w1327 -> [w1337 w1376 w1399 w1457 w1465]
                  tunnel: w1326 -> [_ _ _ _ w1491]
                  tunnel: w1325 -> [_ _ _ _ w1490]
                  tunnel: [w1335 w1356 w1389 w1440 w1468] -> w1324
                  tunnel: [w1336 FALSE FALSE FALSE FALSE] -> w1323
                  tunnel: w1322 -> [_ _ w1398 _ _]
                  frame "Stop", Default {
                    n505 = flat-sequence {
                      tunnel: w1337 -> [w1338]
                      tunnel: [TRUE] -> w1336
                      tunnel: [T16."Stop"] -> w1335
                      frame #0 {
                        n506 = call "TesterOption (SubVI).vi"("2 Options"=FALSE, "On/Off"=FALSE, "Tester Option"=T13."Venable", "VISA Refnum in"=w1338) -> ()  [unwired: 6 in, 2 out]
                      }
                      frame #1 {
                      }
                    }
                  }
                  frame "AO[1]=Meas." {
                    n507 = property on="AO[1]Meas" class="DigNum (strict)"() -> ("Value"=w1350:dbl)  [unwired: 2 in, 2 out]
                    n508 = Number To Fractional String(number=w1350) -> (F-format string=w1358:string)  [unwired: 3 in]
                    n509 = Search and Replace String(input string="EP=1\r\nAO[1]=0\r\n" ("write buffer"), search string="0", replace string=w1358) -> (result string=w1357:string)  [unwired: 5 in, 3 out]
                    n510 = call "SerialMarvinSendGet.vi"("Clear Log"=FALSE, "write buffer"=w1357, "VISA resource name"=w1380) -> ("error out"=w1375:errorcluster)  [unwired: 7 in, 1 out]
                    n511 = call "TesterOption (SubVI).vi"("2 Options"=FALSE, "error in (no error)"=w1375, "On/Off"=FALSE, "Tester Option"=T13."Power", "VISA Refnum in"=w1376) -> ("error out"=w1374:errorcluster, "VISA Refnum out"=w1361:refnum<visa-resource-name>)  [unwired: 5 in]
                    n512 = call "Write panel message (SubVI).vi"("Stop BurnIn"=w1369, 4:"rpm"=w1371, 5:"rpm"=FALSE ("rpm"), "PrintTime"=TRUE, "Stop"=w1370, "error in (no error)"=w1374, "Time to wait"=20.0, "Strin"="Temperature sensor calibration test in process...\nSet Parameters...", "String in"=w1367) -> ("error out"=w1362:errorcluster)  [unwired: 2 in]
                    n513 = call "TesterOption (SubVI).vi"("2 Options"=FALSE, "error in (no error)"=w1362, "On/Off"=FALSE, "Tester Option"=T13."Venable", "VISA Refnum in"=w1361) -> ("error out"=w1355:errorcluster)  [unwired: 5 in, 1 out]
                    n514 = flat-sequence {
                      tunnel: [T16."Stop"] -> w1356
                      tunnel: w1348 -> [_]
                      frame #0 {
                      }
                    }
                    n515 = In Range and Coerce(upper limit=0.1, x=w1350, lower limit=-0.1) -> (In Range?=w1345:bool)  [unwired: 1 out]
                    "SensCalResult" <- w1345
                    n516 = call "Find_Number_LineMARVIN.vi"("Test Paragraph"="Sensor Reading Analog Offset", "error in"=w1355, "TableIn"=w1347) -> ("error out"=w1349:errorcluster, "Line number"=w1353:i32)  [unwired: 2 in, 2 out]
                    n517 = call "PassOrFail (SubVI).vi"("Test#"="2", "index (row)"=w1353, "error in (no error)"=w1349, "Data in"=w1350, "Pass?Fail"=w1345, "Table in"=w1347) -> ("error out"=w1348:errorcluster)  [unwired: 5 in]
                  }
                  frame "TA[5]" {
                    w1401 = T19 [enum."50C", enum."80C", enum."100C", enum."120C"] items=["K15", "K16", "K17", "Venable", "Firmeware", "Fan", "Power", "120C", "110C", "100C", "90C", "80C", "70C", "60C", "50C", "40C", "30C", "25C", "20C", "10C", "0C"]
                    n518 = for {
                      tunnel: w1401 -> [w1416] mode=indexing
                      tunnel: w1400 -> [w1415]
                      tunnel: w1399 -> [w1414]
                      tunnel: w1398 -> [w1413]
                      tunnel: w1397 -> [w1412]
                      tunnel: w1388 -> [w1411]
                      tunnel: w1396 -> [w1410]
                      tunnel: w1395 -> [w1409]
                      tunnel: dbl[] [0.59774, 0.65238, 0.68545, 0.71584] -> [w1404] mode=indexing
                      tunnel: [w1403] -> w1384 mode=indexing
                      tunnel: [w1402] -> w1387
                      n519 = for {
                        N: 5 -> [_]
                        tunnel: w1416 -> [w1434]
                        tunnel: w1415 -> [w1433]
                        tunnel: w1414 -> [w1429]
                        tunnel: w1413 -> [w1427]
                        tunnel: w1412 -> [w1426]
                        tunnel: w1411 -> [w1425]
                        tunnel: w1410 -> [w1423]
                        tunnel: w1409 -> [w1420]
                        tunnel: [w1419] -> w1408 mode=indexing
                        tunnel: [w1418] -> w1402
                        n520 = call "TesterOption (SubVI).vi"("2 Options"=FALSE, "On/Off"=TRUE, "Tester Option"=w1434, "VISA Refnum in"=w1429) -> ("error out"=w1430:errorcluster)  [unwired: 6 in, 1 out]
                        n521 = call "Write panel message (SubVI).vi"("Stop BurnIn"=w1423, 4:"rpm"=w1420, 5:"rpm"=FALSE ("rpm"), "PrintTime"=FALSE, "Stop"=w1425, "error in (no error)"=w1430, "Time to wait"=1.0, "Strin"=w1427, "String in"=w1426) -> ("error out"=w1428:errorcluster)  [unwired: 2 in]
                        n522 = call "SerialMarvinSendGet.vi"("error in (no error)"=w1428, "write buffer"="TA[5]\r\n", "VISA resource name"=w1433) -> ("error out"=w1418:errorcluster, "read buffer"=w1431:string)  [unwired: 7 in]
                        n523 = Fract/Exp String To Number(string=w1431) -> (number=w1419:dbl)  [unwired: 3 in, 1 out]
                      }
                      n524 = Add Array Elements(numeric array=w1408) -> (sum=w1407:dbl)
                      n525 = Divide(x=w1407, y=5.0) -> (x/y=w1405:dbl)
                      n526 = Subtract(x=w1405, y=w1404) -> (x-y=w1403:dbl)
                    }
                    n527 = property class="Bool (strict)"(reference=w1388, error in=w1387) -> ("Value"=w1393:bool)  [unwired: 2 out]
                    n528 = Select(t=T16."Stop", s=w1393, f=T16."AO[1]=Meas.") -> (s? t:f=w1389:T16)
                    n529 = Array Size(array=w1384) -> (size(s)=w1383:i32)
                    n530 = Add Array Elements(numeric array=w1384) -> (sum=w1386:dbl)
                    n531 = Divide(x=w1386, y=w1383) -> (x/y=→"AO[1]Meas":dbl)
                  }
                  frame "AO[1]=0" {
                    n532 = call "SerialMarvinSendGet.vi"("write buffer"="EP=1\r\nAO[1]=0\r\n", "VISA resource name"=w1461) -> ("error out"=w1456:errorcluster)  [unwired: 8 in, 1 out]
                    n533 = call "TesterOption (SubVI).vi"("2 Options"=FALSE, "error in (no error)"=w1456, "On/Off"=FALSE, "Tester Option"=T13."Power", "VISA Refnum in"=w1457) -> ("error out"=w1455:errorcluster, "VISA Refnum out"=w1443:refnum<visa-resource-name>)  [unwired: 5 in]
                    n534 = call "Write panel message (SubVI).vi"("Stop BurnIn"=w1451, 4:"rpm"=w1452, 5:"rpm"=FALSE ("rpm"), "PrintTime"=TRUE, "Stop"=w1437, "error in (no error)"=w1455, "Time to wait"=20.0, "Strin"="Temperature sensor calibration test in process...\nSet Parameters...", "String in"=w1449) -> ("error out"=w1444:errorcluster)  [unwired: 2 in]
                    n535 = call "TesterOption (SubVI).vi"("2 Options"=FALSE, "error in (no error)"=w1444, "On/Off"=FALSE, "Tester Option"=T13."Venable", "VISA Refnum in"=w1443) -> ("error out"=w1438:errorcluster)  [unwired: 5 in, 1 out]
                    n536 = property class="Bool (strict)"(reference=w1437, error in=w1438) -> ("Value"=w1442:bool)  [unwired: 2 out]
                    n537 = Select(t=T16."Stop", s=w1442, f=T16."TA[5]") -> (s? t:f=w1440:T16)
                  }
                  frame "Start" {
                    n538 = call "Write panel message (SubVI).vi"("Stop BurnIn"=w1481, 4:"rpm"=w1480, 5:"rpm"=FALSE ("rpm"), "PrintTime"=FALSE, "Stop"=w1483, "Time to wait"=0.1, "Strin"="Temperature sensor calibration test in process...\nInitialization state...", "String in"=w1485) -> ("error out"=w1486:errorcluster)  [unwired: 3 in]
                    n539 = call "TesterOption (SubVI).vi"("2 Options"=FALSE, "error in (no error)"=w1486, "On/Off"=FALSE, "Tester Option"=T13."Venable", "VISA Refnum in"=w1465) -> ("error out"=w1488:errorcluster)  [unwired: 5 in, 1 out]
                    n540 = call "CANSendMotorSpeed.vi"("Remote"=TRUE, "error in (no error)"=w1488, "Motor Speed RPM"=u16 0, "UUT"=w1490, "CAN Cluster in"=w1491) -> ("error out"=w1475:errorcluster)  [unwired: 6 in]
                    n541 = call "SerialMarvinSendGet.vi"("error in (no error)"=w1475, "write buffer"="AO[1]\r\n", "VISA resource name"=w1477) -> ("error out"=w1464:errorcluster, "read buffer"=w1474:string)  [unwired: 7 in]
                    n542 = Equal?(x=w1474, y="0.0") -> (x = y?=w1466:bool)
                    n543 = property class="Bool (strict)"(reference=w1483, error in=w1464) -> ("Value"=w1495:bool)  [unwired: 2 out]
                    n544 = Select(t=T16."TA[5]", s=w1466, f=T16."AO[1]=0") -> (s? t:f=w1470:T16)
                    n545 = Select(t=T16."Stop", s=w1495, f=w1470) -> (s? t:f=w1468:T16)
                  }
                }
              }
            }
          }
        }
        frame "Auxiliary" {
          w1500 = "Auxiliary test in process..." ("Value")
          w1512 = "Auxiliary Fan Test" ("Test Paragraph")
          n546 = control-ref of="Pannel User Message"() -> (w1511:refnum<vi>)
          n547 = property class="Str"(reference=w1511, error in=w1508, "Value"=w1500) -> (error out=w1510:errorcluster)  [unwired: 1 out]
          n548 = call "Table_ScrollaBarMarvin.vi"("error in"=w1510, "Line to focus"=w1512, "reference in"=w1509) -> ("error out"=w1518:errorcluster)  [unwired: 2 out]
          n549 = property class="Tbl (strict)"(reference=w1509, error in=w1518) -> (reference out=w1507:refnum<vi>, error out=w1517:errorcluster, "Value"=w1516:string[][])
          n550 = Index Array(array=w1516, index (col)=1 ("disabled index (col)")) -> (element=w1515:string[])  [unwired: 1 in]
          n551 = call "Find_Number_Line.vi"("error in"=w1517, "Test Paragraph"=w1512, "Row Headers[]"=w1515) -> ("error out"=w1513:errorcluster, "Line number"=w1498:i32)  [unwired: 1 out]
          n552 = call "Reset old test Values (SubVI).vi"("error in"=w1513, "Atr in"=w1507, "Test Paragraph"=w1512) -> ("error out"=w1505:errorcluster)  [unwired: 8 in]
          n553 = property on="VISA Tester" class="VISAName"() -> ("Value"=w1499:refnum<visa-resource-name>)  [unwired: 2 in, 2 out]
          n554 = control-ref of="Stop Burn-in"() -> (w1502:refnum<vi>)
          n555 = control-ref of="Stop Button"() -> (w1503:refnum<vi>)
          n556 = control-ref of="Pannel User Message"() -> (w1504:refnum<vi>)
          n557 = control-ref of="ATR"() -> (w1497:refnum<vi>)
          n558 = control-ref of="Config_CANAT"() -> ()  [unwired: 1 out]
          n559 = control-ref of="Motor Speed RPM"() -> (w1501:refnum<vi>)
          n560 = while {
            shift-right: [w1524] -> _
            shift-left: enum16{"Stop", "CoolingON", "HotGunON", "Start"}."Start" -> [w1531]
            tunnel: w1505 -> [w1522]
            tunnel: w1504 -> [w1530]
            tunnel: w1503 -> [w1529]
            tunnel: w1502 -> [w1528]
            tunnel: w1501 -> [w1527]
            tunnel: w1500 -> [w1526]
            tunnel: w1499 -> [w1525]
            tunnel: w1498 -> [w1521]
            tunnel: w1497 -> [w1520]
            tunnel: w1496 -> [w1519]
            stop <- w1523 stop-if-true
            n561 = case shown="\"Start\"" w1531 {
              tunnel: w1530 -> [_ w1576 w1671 w1723]
              tunnel: w1529 -> [_ w1571 w1666 w1721]
              tunnel: w1528 -> [_ w1575 w1670 w1722]
              tunnel: w1527 -> [_ w1574 w1669 w1719]
              tunnel: w1526 -> [_ w1565 w1660 w1720]
              tunnel: w1525 -> [_ w1566 w1661 w1717]
              tunnel: [w1533 w1568 w1663 w1712] -> w1524
              tunnel: [w1532 FALSE FALSE FALSE] -> w1523
              tunnel: w1522 -> [_ w1564 w1659 _]
              tunnel: w1521 -> [_ w1559 w1654 w1713]
              tunnel: w1520 -> [_ w1555 w1651 w1715]
              tunnel: w1519 -> [_ _ _ w1724]
              frame "Stop", Default {
                n562 = flat-sequence {
                  tunnel: [enum16{"Stop", "CoolingON", "HotGunON", "Start"}."Stop"] -> w1533
                  tunnel: [TRUE] -> w1532
                  frame #0 {
                    n563 = property on="VISA Tester" class="VISAName"() -> ("Value"=w1537:refnum<visa-resource-name>)  [unwired: 2 in, 2 out]
                    n564 = call "TesterOption (SubVI).vi"("2 Options"=FALSE, "On/Off"=FALSE, "Tester Option"=T13."Venable", "VISA Refnum in"=w1537) -> ()  [unwired: 6 in, 2 out]
                  }
                  frame #1 {
                  }
                }
              }
              frame "CoolingON" {
                n565 = while {
                  tunnel: w1576 -> [w1611]
                  tunnel: w1575 -> [w1610]
                  tunnel: w1574 -> [w1606]
                  tunnel: [w1603] -> w1544
                  tunnel: w1571 -> [w1594]
                  tunnel: w1566 -> [w1580]
                  tunnel: w1565 -> [w1598]
                  tunnel: w1564 -> [w1595]
                  shift-right: [w1587] -> _
                  shift-left: 0.0 -> [w1588]
                  shift-right: [w1583] -> w1543
                  shift-left: 0.0 ("Value") -> [w1585]
                  tunnel: [w1578] -> w1547
                  stop <- w1592 stop-if-true
                  n566 = control-ref of="Power transistor Heat sink Temp."() -> (w1604:refnum<vi>)
                  n567 = property class="DigNum (strict)"(reference=w1604, error in=w1595) -> (error out=w1601:errorcluster, "Value"=w1583:dbl)  [unwired: 1 out]
                  n568 = Equal?(x=w1583, y=w1585) -> (x = y?=w1584:bool)
                  n569 = Number To Fractional String(number=w1583, precision (6)=i16 2) -> (F-format string=w1597:string)  [unwired: 2 in]
                  n570 = case shown="True" w1584 {
                    tunnel: w1588 -> [_ w1631]
                    tunnel: [0.0 w1629] -> w1587
                    tunnel: [FALSE w1628] -> w1586
                    frame False {
                    }
                    frame True {
                      n571 = Increment(x=w1631) -> (x+1=w1629:dbl)
                      n572 = Greater Or Equal?(x=w1629, y=300.0) -> (x >= y?=w1628:bool)
                    }
                  }
                  n573 = Concatenate Strings(w1598, "\nPCB Temperature [C]: " ("string"), w1597) -> (w1596:string)
                  n574 = call "Write panel message (SubVI).vi"("Stop BurnIn"=w1610, 4:"rpm"=w1606, 5:"rpm"=FALSE ("rpm"), "PrintTime"=FALSE, "Stop"=w1594, "error in (no error)"=w1601, "Time to wait"=0.2, "Strin"=w1596, "String in"=w1611) -> ("error out"=w1600:errorcluster)  [unwired: 2 in]
                  n575 = property class="Bool (strict)"(reference=w1594) -> ("Value"=w1593:bool)  [unwired: 1 in, 2 out]
                  n576 = Less Or Equal?(x=w1583, y=52.0) -> (x <= y?=w1582:bool)
                  n577 = call "GetADCTester (SubVI).vi"("error in (no error)"=w1600, "GetADCTester"=T15."Fan", "VISA Refnum in"=w1580) -> ("error out"=w1603:errorcluster, "ADCValOutput Single"=w1590:dbl)  [unwired: 6 in, 1 out]
                  n578 = Greater?(x=w1590, y=u32 2400) -> (0:w1579:bool)
                  n579 = case shown="True" w1582 {
                    tunnel: [w1618 w1625] -> w1581
                    tunnel: w1582 -> [w1618 w1625]
                    tunnel: w1580 -> [w1616 w1623]
                    tunnel: [w1612 w1619] -> w1578
                    frame False {
                      n580 = call "Time Delay11"() -> ("error out"=w1615:errorcluster)  [unwired: 11 in]
                      n581 = call "GetADCTester (SubVI).vi"("error in (no error)"=w1615, "GetADCTester"=T15."Fan", "VISA Refnum in"=w1616) -> ("ADCValOutput Single"=w1614:dbl)  [unwired: 6 in, 2 out]
                      n582 = Greater?(x=w1614, y=2400.0) -> (0:w1612:bool)
                    }
                    frame True {
                      n583 = call "Time Delay10"() -> ("error out"=w1622:errorcluster)  [unwired: 11 in]
                      n584 = call "GetADCTester (SubVI).vi"("error in (no error)"=w1622, "GetADCTester"=T15."Fan", "VISA Refnum in"=w1623) -> ("ADCValOutput Single"=w1621:dbl)  [unwired: 6 in, 2 out]
                      n585 = Greater?(x=w1621, y=2400.0) -> (0:w1619:bool)
                    }
                  }
                  n586 = Compound Arithmetic op=OR(w1579, w1593, w1581, w1586) -> (w1592:bool)
                }
                n587 = In Range and Coerce(upper limit=58.0, x=w1543, lower limit=52.0) -> (In Range?=w1546:bool)  [unwired: 1 out]
                n588 = Build Array(w1547, w1546) -> (w1548:bool[])
                n589 = And Array Elements(Boolean array=w1548) -> (logical AND=→"AuxiOFFResult":bool)
                n590 = Add(x=w1559, y=3) -> (x+y=w1557:i32)
                n591 = call "PassOrFail (SubVI).vi"("index (row)"=w1557, "error in (no error)"=w1544, "Data in"=w1543, "Pass?Fail"=w1546, "Table in"=w1555) -> ("error out"=w1561:errorcluster)  [unwired: 6 in]
                n592 = Select(t="OFF", s=w1547, f="ON") -> (s? t:f=w1551:string)
                n593 = Increment(x=w1557) -> (x+1=w1556:i32)
                n594 = call "PassOrFail (SubVI).vi"("String Res"=w1551, "index (row)"=w1556, "error in (no error)"=w1561, "Data in"=-3.0, "Pass?Fail"=w1547, "Table in"=w1555) -> ("error out"=w1560:errorcluster)  [unwired: 5 in]
                n595 = call "TesterOption (SubVI).vi"("2 Options"=FALSE, "error in (no error)"=w1560, "On/Off"=FALSE, "Tester Option"=T13."Venable" ("Tester Option 2"), "VISA Refnum in"=w1566) -> ("error out"=w1541:errorcluster)  [unwired: 5 in, 1 out]
                n596 = call "Time Delay14"("error in (no error)"=w1541) -> ("error out"=w1540:errorcluster)  [unwired: 10 in]
                n597 = property class="Bool (strict)"(reference=w1571, error in=w1540) -> ("Value"=w1577:bool)  [unwired: 2 out]
                n598 = Select(t=enum16{"Stop", "CoolingON", "HotGunON", "Start"}."Stop", s=w1577, f=enum16{"Stop", "CoolingON", "HotGunON", "Start"}."Stop") -> (s? t:f=w1568:enum16{"Stop", "CoolingON", "HotGunON", "Start"})
              }
              frame "HotGunON" {
                n599 = while {
                  tunnel: w1671 -> [w1704]
                  tunnel: w1670 -> [w1703]
                  tunnel: w1669 -> [w1699]
                  tunnel: [w1695] -> w1641
                  tunnel: w1666 -> [w1686]
                  tunnel: w1661 -> [w1696]
                  tunnel: w1660 -> [w1690]
                  tunnel: w1659 -> [w1687]
                  shift-right: [w1679] -> _
                  shift-left: 0.0 -> [w1680]
                  shift-right: [w1676] -> _
                  shift-left: 0.0 ("Value") -> [w1677]
                  tunnel: [w1674] -> w1639
                  stop <- w1684 stop-if-true
                  n600 = control-ref of="Power transistor Heat sink Temp."() -> (w1697:refnum<vi>)
                  n601 = property class="DigNum (strict)"(reference=w1697, error in=w1687) -> (error out=w1693:errorcluster, "Value"=w1676:dbl)  [unwired: 1 out]
                  n602 = Equal?(x=w1676, y=w1677) -> (x = y?=w1675:bool)
                  n603 = Number To Fractional String(number=w1676, precision (6)=i16 2) -> (F-format string=w1689:string)  [unwired: 2 in]
                  n604 = case shown="True" w1675 {
                    tunnel: w1680 -> [_ w1710]
                    tunnel: [0.0 w1708] -> w1679
                    tunnel: [FALSE w1707] -> w1678
                    frame False {
                    }
                    frame True {
                      n605 = Increment(x=w1710) -> (x+1=w1708:dbl)
                      n606 = Greater Or Equal?(x=w1708, y=300.0) -> (x >= y?=w1707:bool)
                    }
                  }
                  n607 = Concatenate Strings(w1690, "\nPCB Temperature [C]: " ("string"), w1689) -> (w1688:string)
                  n608 = call "Write panel message (SubVI).vi"("Stop BurnIn"=w1703, 4:"rpm"=w1699, 5:"rpm"=FALSE ("rpm"), "PrintTime"=FALSE, "Stop"=w1686, "error in (no error)"=w1693, "Time to wait"=0.2, "Strin"=w1688, "String in"=w1704) -> ("error out"=w1692:errorcluster)  [unwired: 2 in]
                  n609 = property class="Bool (strict)"(reference=w1686) -> ("Value"=w1685:bool)  [unwired: 1 in, 2 out]
                  n610 = call "GetADCTester (SubVI).vi"("error in (no error)"=w1692, "GetADCTester"=T15."Fan", "VISA Refnum in"=w1696) -> ("error out"=w1695:errorcluster, "ADCValOutput Single"=w1682:dbl)  [unwired: 6 in, 1 out]
                  n611 = Greater Or Equal?(x=w1676, y=61.0) -> (x >= y?=w1673:bool)
                  n612 = Less?(x=w1682, y=u32 100) -> (x < y?=w1674:bool)
                  n613 = Compound Arithmetic op=OR(w1674, w1685, w1673, w1678) -> (w1684:bool)
                }
                n614 = control-ref of="Power transistor Heat sink Temp."() -> (w1644:refnum<vi>)
                n615 = property class="DigNum (strict)"(reference=w1644, error in=w1641) -> (error out=w1643:errorcluster, "Value"=w1642:dbl)  [unwired: 1 out]
                n616 = In Range and Coerce(upper limit=62.0, x=w1642, lower limit=58.0) -> (In Range?=w1638:bool)  [unwired: 1 out]
                n617 = Build Array(w1639, w1638) -> (w1640:bool[])
                n618 = Increment(x=w1654) -> (x+1=w1653:i32)
                n619 = call "PassOrFail (SubVI).vi"("index (row)"=w1653, "error in (no error)"=w1643, "Data in"=w1642, "Pass?Fail"=w1638, "Table in"=w1651) -> ("error out"=w1656:errorcluster)  [unwired: 6 in]
                n620 = And Array Elements(Boolean array=w1640) -> (logical AND=→"AuxiONResult":bool)
                n621 = Increment(x=w1653) -> (x+1=w1652:i32)
                n622 = Select(t="ON", s=w1639, f="OFF") -> (s? t:f=w1649:string)
                n623 = call "PassOrFail (SubVI).vi"("String Res"=w1649, "index (row)"=w1652, "error in (no error)"=w1656, "Data in"=-3.0, "Pass?Fail"=w1639, "Table in"=w1651) -> ("error out"=w1655:errorcluster)  [unwired: 5 in]
                n624 = call "TesterOption (SubVI).vi"("On/Off 2"=FALSE, "Tester Option 2"=T13."Venable", "2 Options"=TRUE, "error in (no error)"=w1655, "On/Off"=FALSE, "Tester Option"=T13."Fan", "VISA Refnum in"=w1661) -> ("error out"=w1633:errorcluster)  [unwired: 3 in, 1 out]
                n625 = call "Time Delay13"("error in (no error)"=w1633) -> ("error out"=w1632:errorcluster)  [unwired: 10 in]
                n626 = property class="Bool (strict)"(reference=w1666, error in=w1632) -> ("Value"=w1672:bool)  [unwired: 2 out]
                n627 = Select(t=enum16{"Stop", "CoolingON", "HotGunON", "Start"}."Stop", s=w1672, f=enum16{"Stop", "CoolingON", "HotGunON", "Start"}."CoolingON") -> (s? t:f=w1663:enum16{"Stop", "CoolingON", "HotGunON", "Start"})
              }
              frame "Start" {
                n628 = call "Write panel message (SubVI).vi"("Stop BurnIn"=w1722, 4:"rpm"=w1719, 5:"rpm"=FALSE ("rpm"), "PrintTime"=FALSE, "Stop"=w1721, "Time to wait"=1.0, "Strin"=w1720, "String in"=w1723) -> ("error out"=w1730:errorcluster)  [unwired: 3 in]
                n629 = call "TesterOption (SubVI).vi"("2 Options"=FALSE, "error in (no error)"=w1730, "On/Off"=FALSE, "Tester Option"=T13."Venable", "VISA Refnum in"=w1717) -> ("error out"=w1725:errorcluster)  [unwired: 5 in, 1 out]
                n630 = while {
                  tunnel: w1725 -> [w1751]
                  tunnel: w1724 -> [w1750]
                  tunnel: w1723 -> [w1749]
                  tunnel: w1722 -> [w1748]
                  tunnel: w1721 -> [w1747]
                  tunnel: w1720 -> [w1746]
                  tunnel: w1719 -> [w1745]
                  shift-right: [w1742] -> _
                  shift-left: enum16{"Wait", "OFF", "ON", "Start"}."Start" -> [w1744]
                  tunnel: w1717 -> [w1743]
                  shift-right: [w1740] -> _
                  shift-left: 0 -> [w1741]
                  tunnel: w1715 -> [w1738]
                  shift-right: [w1737] -> w1711
                  shift-left: TRUE -> [w1736]
                  tunnel: w1713 -> [w1735]
                  stop <- w1739 stop-if-true
                  n631 = case shown="\"Start\"" w1744 {
                    tunnel: w1751 -> [_ w1798 _ w1861]
                    tunnel: w1750 -> [w1766 w1797 _ w1860]
                    tunnel: w1749 -> [_ w1795 _ w1858]
                    tunnel: w1748 -> [_ w1794 _ w1857]
                    tunnel: w1747 -> [_ w1773 _ w1841]
                    tunnel: w1746 -> [_ w1793 _ w1856]
                    tunnel: w1745 -> [_ w1792 _ w1855]
                    tunnel: w1743 -> [_ w1785 _ w1848]
                    tunnel: [w1769 w1775 enum16{"Wait", "OFF", "ON", "Start"}."OFF" w1838] -> w1742
                    tunnel: w1741 -> [w1770 w1783 _ w1846]
                    tunnel: [w1770 w1782 0 w1845] -> w1740
                    tunnel: [w1768 FALSE FALSE FALSE] -> w1739
                    tunnel: w1738 -> [w1754 _ w1834 _]
                    tunnel: [FALSE w1779 TRUE w1842] -> w1737
                    tunnel: w1736 -> [w1757 _ w1835 _]
                    tunnel: w1735 -> [w1756 _ w1833 _]
                    frame "Wait", Default {
                      n632 = call "SerialMarvinSendGet.vi"("write buffer"="EP=1\r\nAU=0\r\n", "VISA resource name"=w1766) -> ("error out"=w1765:errorcluster)  [unwired: 8 in, 1 out]
                      n633 = call "Time Delay19"("error in (no error)"=w1765) -> ("error out"=w1753:errorcluster)  [unwired: 10 in]
                      n634 = Not(x=w1757) -> (.not. x?=w1759:bool)
                      n635 = Select(t="OFF", s=w1759, f="ON") -> (s? t:f=w1758:string)
                      n636 = Add(x=2, y=w1756) -> (x+y=w1763:i32)
                      n637 = call "PassOrFail (SubVI).vi"("String Res"=w1758, "index (row)"=w1763, "error in (no error)"=w1753, "Data in"=-3.0, "Pass?Fail"=w1759, "Table in"=w1754) -> ("error out"=w1752:errorcluster)  [unwired: 5 in]
                      n638 = flat-sequence {
                        tunnel: [enum16{"Wait", "OFF", "ON", "Start"}."Wait"] -> w1769
                        tunnel: [TRUE] -> w1768
                        tunnel: w1752 -> [_]
                        frame #0 {
                        }
                      }
                    }
                    frame "OFF" {
                      n639 = call "SerialMarvinSendGet.vi"("error in (no error)"=w1798, "write buffer"="EP=1\r\nAU=0\r\n", "VISA resource name"=w1797) -> ("error out"=w1787:errorcluster)  [unwired: 7 in, 1 out]
                      n640 = call "Time Delay"("error in (no error)"=w1787) -> ("error out"=w1781:errorcluster)  [unwired: 10 in]
                      n641 = call "GetADCTester (SubVI).vi"("error in (no error)"=w1781, "GetADCTester"=T15."Fan", "TimeToGet"=5, "VISA Refnum in"=w1785) -> ("error out"=w1786:errorcluster, "ADCValOutput Single"=w1789:dbl)  [unwired: 5 in, 1 out]
                      n642 = Greater?(x=w1789, y=2400.0) -> (0:w1784:bool)
                      n643 = case shown="True" w1784 {
                        tunnel: w1795 -> [_ w1817]
                        tunnel: w1794 -> [_ w1816]
                        tunnel: w1773 -> [_ w1815]
                        tunnel: w1793 -> [_ w1814]
                        tunnel: w1792 -> [_ w1813]
                        tunnel: w1786 -> [w1800 w1812]
                        tunnel: [w1801 w1810] -> w1774
                        tunnel: w1783 -> [w1805 _]
                        tunnel: [w1806 0] -> w1782
                        tunnel: [w1800 w1808] -> w1776
                        tunnel: [w1799 FALSE] -> w1779
                        frame False {
                          n644 = Increment(x=w1805) -> (x+1=w1806:i32)
                          n645 = Greater Or Equal?(x=w1805, y=10) -> (x >= y?=w1799:bool)
                          n646 = Select(t=enum16{"Wait", "OFF", "ON", "Start"}."Wait", s=w1799, f=enum16{"Wait", "OFF", "ON", "Start"}."OFF") -> (s? t:f=w1801:enum16{"Wait", "OFF", "ON", "Start"})
                        }
                        frame True {
                          n647 = call "Write panel message (SubVI).vi"("Stop BurnIn"=w1816, 4:"rpm"=w1813, 5:"rpm"=FALSE ("rpm"), "PrintTime"=TRUE, "Stop"=w1815, "error in (no error)"=w1812, "Time to wait"=5.0, "Strin"=w1814, "String in"=w1817) -> ("error out"=w1811:errorcluster)  [unwired: 2 in]
                          n648 = flat-sequence {
                            tunnel: w1811 -> [w1821]
                            tunnel: [enum16{"Wait", "OFF", "ON", "Start"}."Wait"] -> w1810
                            tunnel: [w1821] -> w1808
                            frame #0 {
                            }
                          }
                        }
                      }
                      n649 = property class="Bool (strict)"(reference=w1773, error in=w1776) -> ("Value"=w1778:bool)  [unwired: 2 out]
                      n650 = Select(t=enum16{"Wait", "OFF", "ON", "Start"}."Wait", s=w1778, f=w1774) -> (s? t:f=w1775:enum16{"Wait", "OFF", "ON", "Start"})
                    }
                    frame "ON" {
                      n651 = Not(x=w1835) -> (.not. x?=w1828:bool)
                      n652 = Select(t="ON", s=w1828, f="OFF") -> (s? t:f=w1827:string)
                      n653 = Increment(x=w1833) -> (x+1=w1832:i32)
                      n654 = call "PassOrFail (SubVI).vi"("String Res"=w1827, "index (row)"=w1832, "Data in"=-3.0, "Pass?Fail"=w1828, "Table in"=w1834) -> ()  [unwired: 6 in, 1 out]
                    }
                    frame "Start" {
                      n655 = call "SerialMarvinSendGet.vi"("error in (no error)"=w1861, "write buffer"="EP=1\r\nAU=1\r\n", "VISA resource name"=w1860) -> ("error out"=w1850:errorcluster)  [unwired: 7 in, 1 out]
                      n656 = call "Time Delay18"("error in (no error)"=w1850) -> ("error out"=w1844:errorcluster)  [unwired: 10 in]
                      n657 = call "GetADCTester (SubVI).vi"("error in (no error)"=w1844, "GetADCTester"=T15."Fan", "TimeToGet"=5, "VISA Refnum in"=w1848) -> ("error out"=w1849:errorcluster, "ADCValOutput Single"=w1852:dbl)  [unwired: 5 in, 1 out]
                      n658 = Less?(x=w1852, y=100.0) -> (x < y?=w1847:bool)
                      n659 = case shown="False" w1847 {
                        tunnel: w1858 -> [_ w1880]
                        tunnel: w1857 -> [_ w1879]
                        tunnel: w1841 -> [_ w1878]
                        tunnel: w1856 -> [_ w1877]
                        tunnel: w1855 -> [_ w1876]
                        tunnel: w1849 -> [w1863 w1875]
                        tunnel: [w1864 w1873] -> w1839
                        tunnel: w1846 -> [w1868 _]
                        tunnel: [w1869 0] -> w1845
                        tunnel: [w1863 w1871] -> w1836
                        tunnel: [w1862 FALSE] -> w1842
                        frame False {
                          n660 = Increment(x=w1868) -> (x+1=w1869:i32)
                          n661 = Greater Or Equal?(x=w1868, y=5) -> (x >= y?=w1862:bool)
                          n662 = Select(t=enum16{"Wait", "OFF", "ON", "Start"}."ON", s=w1862, f=enum16{"Wait", "OFF", "ON", "Start"}."Start") -> (s? t:f=w1864:enum16{"Wait", "OFF", "ON", "Start"})
                        }
                        frame True {
                          n663 = call "Write panel message (SubVI).vi"("Stop BurnIn"=w1879, 4:"rpm"=w1876, 5:"rpm"=FALSE ("rpm"), "PrintTime"=TRUE, "Stop"=w1878, "error in (no error)"=w1875, "Time to wait"=60.0, "Strin"=w1877, "String in"=w1880) -> ("error out"=w1874:errorcluster)  [unwired: 2 in]
                          n664 = flat-sequence {
                            tunnel: w1874 -> [w1884]
                            tunnel: [enum16{"Wait", "OFF", "ON", "Start"}."ON"] -> w1873
                            tunnel: [w1884] -> w1871
                            frame #0 {
                            }
                          }
                        }
                      }
                      n665 = property class="Bool (strict)"(reference=w1841, error in=w1836) -> ("Value"=w1840:bool)  [unwired: 2 out]
                      n666 = Select(t=enum16{"Wait", "OFF", "ON", "Start"}."Wait", s=w1840, f=w1839) -> (s? t:f=w1838:enum16{"Wait", "OFF", "ON", "Start"})
                    }
                  }
                }
                n667 = flat-sequence {
                  tunnel: [enum16{"Stop", "CoolingON", "HotGunON", "Start"}."Stop"] -> w1712
                  tunnel: w1711 -> [_]
                  frame #0 {
                  }
                }
              }
            }
          }
        }
      }
      "CurrentTest" <- w65
    }
    n668 = flat-sequence {
      tunnel: w52 -> [_]
      frame #0 {
        w60 = T21."Enabled" ("Disabled")
        w61 = FALSE ("Start")
        n669 = property on="Start" class="Bool (strict)"("Value"=w61, "DisabledEnum"=w60) -> ()  [unwired: 2 in, 2 out]
        n670 = property on="Report" class="Bool (strict)"("Value"=w61, "DisabledEnum"=w60) -> ()  [unwired: 2 in, 2 out]
      }
    }
  }
  n671 = while {
    shift-right: [w1900] -> _
    shift-left: w33 -> [w1902]
    shift-right: [w1898] -> _
    shift-left: _ -> [w1899]
    shift-right: [w1894] -> _
    shift-left: w31 -> [w1894]
    shift-right: [w1892] -> _
    shift-left: w26 -> [w1893]
    shift-right: [w1891] -> _
    shift-left: w26 -> [w1890]
    shift-right: [w1889] -> _
    shift-left: w26 -> [w1888]
    shift-right: [w1887] -> _
    shift-left: w26 -> [w1886]
    stop <- w1901 stop-if-true
    n672 = Dequeue Element(queue=w1902, error in (no error)=w1894) -> (queue out=w1900:refnum<queue>, element=w1895:T10, error out=w1901:errorcluster)  [unwired: 1 in, 1 out]
    n673 = for {
      tunnel: [w2031] -> w1897 mode=indexing
      tunnel: w1895 -> [w2030] mode=indexing
      tunnel: [w2029] -> w1896 mode=indexing
      n674 = Unbundle By Name(w2030) -> ("aDATA"=w2029:u8[])
      n675 = call "Array Data to Single Num in Hex.vi"("aDATA"=w2029) -> ("Numeric"=w2031:u64)  [unwired: 10 in]
    }
    n676 = Build Array (concatenate)(w1897, w1899) -> (w1898:u64[][])
    "Array" <- w1898
    n677 = for {
      tunnel: w1896 -> [w1912] mode=indexing
      shift-right: [w1909] -> w1892
      shift-left: w1893 -> [w1910]
      shift-right: [w1908] -> w1891
      shift-left: w1890 -> [w1907]
      shift-right: [w1906] -> w1889
      shift-left: w1888 -> [w1905]
      shift-right: [w1904] -> w1887
      shift-left: w1886 -> [w1903]
      i -> [w1911]
      n678 = case shown="0, Default" w1911 {
        tunnel: w1912 -> [w1952 w1985 w2024]
        tunnel: w1910 -> [w1926 w1974 w2013]
        tunnel: [w1924 w1974 w2013] -> w1909
        tunnel: [w1921 w1973 w2012] -> w1908
        tunnel: w1907 -> [w1920 w1973 w2012]
        tunnel: [w1915 w1972 w2011] -> w1906
        tunnel: w1905 -> [w1914 w1972 w2011]
        tunnel: [w1913 w1971 w2006] -> w1904
        tunnel: w1903 -> [w1913 w1971 w2005]
        frame 0, Default {
          # "Frame ID\n0x18E1273F"
          n679 = Index Array(array=w1952, index #1=0 ("index"), index #2=1 ("index"), index #3=2 ("index"), index #4=3 ("index"), index #5=4 ("index"), index #6=5 ("index"), index #7=6 ("index"), index #8=7 ("index")) -> (element #1=w1936:u8, element #2=w1938:u8, element #3=w1939:u8, element #4=w1943:u8, element #5=w1946:u8, element #6=w1950:u8, element #7=w1951:u8, element #8=w1949:u8)
          n680 = Number To Hexadecimal String(2:w1949) -> (0:w1963:string)  [unwired: 1 in]
          n681 = Join Numbers(hi=w1951, lo=w1950) -> ((hi.lo)=w1970:u16)
          n682 = Join Numbers(hi=w1939, lo=w1938) -> ((hi.lo)=w1940:u16)
          n683 = Number To Hexadecimal String(2:w1946) -> (0:w1947:string)  [unwired: 1 in]
          n684 = Number To Hexadecimal String(2:w1970) -> (0:w1969:string)  [unwired: 1 in]
          n685 = Number To Hexadecimal String(2:w1936) -> (0:w1937:string)  [unwired: 1 in]
          n686 = Number To Hexadecimal String(2:w1940) -> (0:w1941:string)  [unwired: 1 in]
          n687 = Number To Hexadecimal String(2:w1943) -> (0:w1944:string)  [unwired: 1 in]
          n688 = Hexadecimal String To Number(string=w1963) -> (number=w1962:u32)  [unwired: 2 in, 1 out]
          n689 = To Double Precision Float(number=w1962) -> (double precision float=→"DC Current":dbl)
          n690 = Hexadecimal String To Number(string=w1947) -> (number=w1948:u32)  [unwired: 2 in, 1 out]
          n691 = Hexadecimal String To Number(string=w1969) -> (number=w1968:u32)  [unwired: 2 in, 1 out]
          n692 = Hexadecimal String To Number(string=w1937) -> (number=w1934:u32)  [unwired: 2 in, 1 out]
          n693 = Hexadecimal String To Number(string=w1941) -> (number=w1942:u32)  [unwired: 2 in, 1 out]
          n694 = Hexadecimal String To Number(string=w1944) -> (number=w1945:u32)  [unwired: 2 in, 1 out]
          n695 = To Double Precision Float(number=u32 10 ("y")) -> (double precision float=w1966:dbl)
          n696 = To Double Precision Float(number=w1968) -> (double precision float=w1965:dbl)
          n697 = To Double Precision Float(number=w1948) -> (double precision float=w1931:dbl)
          n698 = To Double Precision Float(number=w1942) -> (double precision float=w1927:dbl)
          n699 = To Double Precision Float(number=w1945) -> (double precision float=w1933:dbl)
          n700 = Divide(x=w1965, y=w1966) -> (x/y=→"DC Voltage":dbl)
          n701 = To Unsigned Word Integer(number=w1934) -> (unsigned 16bit integer=→"ECS State":u16)
          n702 = Subtract(x=w1931, y=50.0 ("x")) -> (x-y=w1919:dbl)
          n703 = Subtract(x=w1933, y=50.0 ("x")) -> (x-y=w1922:dbl)
          n704 = call "Filter (SubVI).vi"("Delta"=5000.0, "NewVal"=w1927, "OldVal"=w1926) -> ("Val"=w1924:dbl)  [unwired: 8 in]
          "Motor Speed RPM" <- w1924
          n705 = Less Than 0?(x=w1922) -> (x < 0?=w1929:bool)
          n706 = Less Than 0?(x=w1919) -> (x < 0?=w1928:bool)
          n707 = Select(t=w1920, s=w1929, f=w1922) -> (s? t:f=w1923:dbl)
          n708 = Select(t=w1914, s=w1928, f=w1919) -> (s? t:f=w1918:dbl)
          n709 = call "Filter (SubVI).vi"("Delta"=130.0, "NewVal"=w1923, "OldVal"=w1920) -> ("Val"=w1921:dbl)  [unwired: 8 in]
          "Motor Stator Temp." <- w1921
          n710 = call "Filter (SubVI).vi"("Delta"=100.0, "NewVal"=w1918, "OldVal"=w1914) -> ("Val"=w1915:dbl)  [unwired: 8 in]
          "Power transistor Heat sink Temp." <- w1915
        }
        frame 1 {
          # "Framde ID\n0x18E3273F"
          n711 = control-ref of="UUT"() -> (w1975:refnum<vi>)
          n712 = property on="Property Node" class="DigNum (strict)"(reference=w1975) -> ("Value"=w1976:u8)  [unwired: 1 in, 2 out]
          n713 = Index Array(array=w1985, index #1=0 ("index"), index #2=1 ("index")) -> (element #1=w1983:u8, element #2=w1978:u8)
          n714 = Number To Boolean Array(number=w1983) -> (Boolean array=w1982:bool[])
          n715 = Number To Boolean Array(number=w1978) -> (Boolean array=w1980:bool[])
          n716 = Boolean To (0,1)(Boolean=w1980) -> (0, 1=w1977:i16[])
          n717 = Boolean To (0,1)(Boolean=w1982) -> (0, 1=w1981:i16[])
          n718 = case shown="95" w1976 {
            tunnel: w1977 -> [_ w1986]
            frame 0, Default {
            }
            frame 95 {
              n719 = for {
                tunnel: w1986 -> [w1991] mode=indexing
                i -> [w1987]
                stop <- w1989 stop-if-true
                n720 = Not Equal To 0?(x=w1991) -> (x != 0?=w1990:bool)
                n721 = case shown="0, Default" w1987 {
                  tunnel: w1990 -> [w1992 w1993]
                  frame 0, Default {
                    "Ambient Sensor temp" <- w1992
                  }
                  frame 1 {
                    "Ambient Over temp" <- w1993
                  }
                }
                n722 = Equal?(x=w1987, y=1.0) -> (x = y?=w1989:bool)
              }
            }
          }
          n723 = for {
            tunnel: w1981 -> [w1995] mode=indexing
            i -> [w1996]
            n724 = Not Equal To 0?(x=w1995) -> (x != 0?=w1994:bool)
            n725 = case shown="1" w1996 {
              tunnel: w1994 -> [w1997 w1998 w1999 w2000 w2001 w2002 w2003 w2004]
              frame 0, Default {
                "Drive Sensor temp Failure" <- w1997
              }
              frame 1 {
                "Drive Over temperature" <- w1998
              }
              frame 2 {
                "Motor Sensor temp Fauilre" <- w1999
              }
              frame 3 {
                "Motor Over temperature" <- w2000
              }
              frame 4 {
                "Derated drive temp" <- w2001
              }
              frame 5 {
                "Under voltage/Over voltage" <- w2002
              }
              frame 6 {
                "Commutation err" <- w2003
              }
              frame 7 {
                "Speed error" <- w2004
              }
            }
          }
        }
        frame 2 {
          # "Frame ID\n0x18E2273F"
          n726 = Index Array(array=w2024, index #1=0 ("index"), index #2=1 ("index")) -> (element #1=w2021:u8, element #2=w2018:u8)
          n727 = disable-structure shown="Enabled" {
            disable-tunnel: [w2027 w2028] -> w2022
            disable-tunnel: w2021 -> [w2026 w2028]
            frame Disabled {
              n728 = Number To Hexadecimal String(2:w2026) -> (0:w2025:string)  [unwired: 1 in]
              n729 = Hexadecimal String To Number(string=w2025) -> (number=w2027:u32)  [unwired: 2 in, 1 out]
            }
            frame Enabled {
            }
          }
          n730 = Number To Hexadecimal String(2:w2018) -> (0:w2016:string)  [unwired: 1 in]
          n731 = Hexadecimal String To Number(string=w2016) -> (number=w2017:u32)  [unwired: 2 in, 1 out]
          n732 = To Double Precision Float(number=w2017) -> (double precision float=w2015:dbl)
          n733 = To Double Precision Float(number=w2022) -> (double precision float=→"Motor Phase Current RMS":dbl)
          n734 = Subtract(x=w2015, y=50.0) -> (x-y=w2009:dbl)
          n735 = Less Than 0?(x=w2009) -> (x < 0?=w2010:bool)
          n736 = Select(t=w2005, s=w2010, f=w2009) -> (s? t:f=w2008:dbl)
          n737 = call "Filter (SubVI).vi"("Delta"=65.0, "NewVal"=w2008, "OldVal"=w2005) -> ("Val"=w2006:dbl)  [unwired: 8 in]
          "Ambient Temperature" <- w2006
        }
      }
    }
  }
  n738 = while {
    shift-right: [w2036] -> _
    shift-left: T11."Initialize" -> [w2055]
    shift-right: [w2052] -> _
    shift-left: _ -> [w2051]
    shift-right: [w2050] -> _
    shift-left: w33 -> [w2048]
    shift-right: [w2049] -> _
    shift-left: refnum<vi> refnum ("Config_CANAT") -> [w2047]
    shift-right: [w2045] -> _
    shift-left: w30 -> [w2046]
    tunnel: "ATR" -> [_]
    tunnel: w22 -> [w2044]
    tunnel: w21 -> [w2043]
    shift-right: [w2041] -> _
    shift-left: w1 -> [w2042]
    tunnel: w8 -> [w2040]
    tunnel: w2 -> [w2039]
    tunnel: w19 -> [_]
    tunnel: w31 -> [w2054]
    tunnel: [w2053] -> _
    tunnel: w9 -> [_]
    tunnel: w6 -> [w2037]
    shift-right: [w2034] -> _
    shift-left: w1 -> [w2035]
    shift-right: [w2032] -> _
    shift-left: w1 -> [w2033]
    stop <- w2038 stop-if-true
    n739 = case shown="\"MainProgram\"" w2055 {
      tunnel: [w2062 w2205 w2280 T11."Erase ATR Table"] -> w2036
      tunnel: [FALSE w2191 FALSE FALSE] -> w2038
      tunnel: [w2058 w2196 w2274 w3232] -> w2053
      tunnel: w2054 -> [_ w2216 w2278 _]
      tunnel: [w2098 refnum<visa-resource-name> refnum ("VISA resource name") w2275 w3236] -> w2052
      tunnel: w2051 -> [w2098 w2224 w2276 _]
      tunnel: [w2089 w2185 w2270 w3230] -> w2050
      tunnel: [w2088 refnum<vi> refnum ("Config_CANAT") w2271 w3233] -> w2049
      tunnel: w2048 -> [w2089 w2226 w2273 w3230]
      tunnel: w2047 -> [w2088 w2208 w2272 _]
      tunnel: w2046 -> [w2087 w2219 w2269 w3229]
      tunnel: [w2087 w2184 w2268 w3229] -> w2045
      tunnel: w2044 -> [_ _ w2267 _]
      tunnel: w2043 -> [_ _ w2266 _]
      tunnel: w2042 -> [w2084 w2210 w2265 w3226]
      tunnel: [w2084 w2210 w2264 w3226] -> w2041
      tunnel: w2040 -> [w2074 _ w2263 _]
      tunnel: w2039 -> [_ _ w2262 _]
      tunnel: w2037 -> [_ _ w2261 _]
      tunnel: w2035 -> [_ _ w2260 _]
      tunnel: [w2056 w2183 w2259 w3217] -> w2034
      tunnel: w2033 -> [_ _ w2258 _]
      tunnel: [w2056 w2183 w2257 w3217] -> w2032
      frame "Erase ATR Table", Default {
        w2056 = 0
        w2066 = T21."Enabled" ("Disabled")
        w2078 = "Marvin" ("section")
        w2085 = refnum<visa-resource-name> "COM4" ("VISA resource name")
        w2094 = FALSE ("Visible")
        n740 = property on="Serial Com" class="Bool"(error in=errorcluster {"status"=FALSE, "code"=0, "source"=""} ("error out"), "Visible"=TRUE) -> (error out=w2086:errorcluster)  [unwired: 1 in, 1 out]
        n741 = property on="VISA Marvin" class="VISAName"(error in=w2086, "Visible"=w2094, "Value"=w2085) -> (error out=w2096:errorcluster)  [unwired: 1 in, 1 out]
        n742 = property on="VISA Marvin" class="VISAName"(error in=w2086, "Value"=w2085) -> ()  [unwired: 1 in, 2 out]
        n743 = property on="Status" class="Bool (strict)"(error in=w2096, "Value"=w2094) -> (error out=w2069:errorcluster)  [unwired: 1 in, 1 out]
        n744 = call "Select UUT"("error in (no error)"=w2069) -> ("EBAY"=w2067:bool, "error out"=w2068:errorcluster)  [unwired: 17 in]
        n745 = case shown="True" w2067 {
          tunnel: [string[][] [["1", "Communication Test", "", "", "", "", ""], ["1.1", "Serial RS-232", "N/A", "-", "", "", ""], ["1.2", "CAN Bus", "N/A", "-", "", "", ""], ["", "", "", "", "", "", ""], ["2", "Temperature Sensor Calibration", "", "", "", "", ""], ["2.1", "Sensor Reading Analog Offset", "0", "+/-0.100", ".", "", ""], ["", "", "", "", "", "", ""], ["3", "Motor Termistor Input Test", "", "", "", "", ""], ["3.1", "60 Degree", "60", "+/-3.00", "°C", "", ""], ["3.2", "90 Degree", "90", "+/-3.00", "°C", "", ""], ["3.3", "120 Degree", "120", "+/-3.00", "°C", "", ""], ["", "", "", "", "", "", ""], ["4", "Enable Test", "", "", "", "", ""], ["4.1", "Fan Speed at Opened Enable ", "5000", "+/-200.0", "rpm", "", ""], ["4.2", "Fan Speed at Opened Enable ", "0", "+/-200.0", "rpm", "", ""], ["4.3", "Fan Speed at Closed Enable ", "5000", "+/-200.0", "rpm", "", ""], ["4.4", "Motor Rotation Direction", "CCW", "-", "", "", ""], ["", "", "", "", "", "", ""], ["5", "Speed Command Test", "", "", "", "", ""], ["5.1", "Fan  Speed", "6000", "+/-200.0", "rpm", "", ""], ["5.2", "Fan  Speed", "9000", "+/-200.0", "rpm", "", ""], ["5.3", "Fan  Speed", "12100", "+/-200.0", "rpm", "", ""], ["", "", "", "", "", "", ""], ["6", "Motor Stop time", "< 50", "-", "sec", "", ""], ["", "", "", "", "", "", ""], ["7", "Burn-in Test", "", "", "", "", ""], ["7.1", "DC Input Current", "28", "+/-5.000", "A", "", ""], ["7.2", "Fan speed", "12100", "+/-200.0", "rpm", "", ""], ["7.3", "Ambient Temperature", "25", "+/-13.00", "°C", "", ""], ["7.4", "After 10 min of operation", "", "-", "°C", "", ""], ["7.5", "After 20 min of operation", "", "-", "°C", "", ""], ["7.6", "After 30 min of operation", "", "-", "°C", "", ""], ["", "", "", "", "", "", ""], ["8", "Visual Inspection", "", "", "", "", ""], ["8.1", "Verification of Components Not Installed", "N/A", "-", "", "", ""], ["8.2", "Manufacturing Defects", "N/A", "-", "", "", ""], ["", "", "", "", "", "", ""], ["9", "Power Supply Testing", "", "", "", "", ""], ["9.1", "DC Input Current Drawn", "150", "+/-10.00", "mA", "", ""], ["", "", "", "", "", "", ""], ["10", "Power Supply Voltages", "", "", "", "", ""], ["10.1", "12V", "12.0", "+/-0.500", "V", "", ""], ["10.2", "5V", "5.0", "+/-0.200", "V", "", ""], ["10.3", "3.3V", "3.3", "+/-0.100", "V", "", ""], ["10.4", "1.8V", "1.8", "+/-0.100", "V", "", ""], ["", "", "", "", "", "", ""], ["11", "Reverse Polarity Test - DC Input Current", "< 1", "-", "mA", "", ""], ["", "", "", "", "", "", ""], ["12", "Functional Test Procedure", "", "", "", "", ""], ["12.1", "Weight Check", "3800", "+/-100.0", "gr", "", ""], ["", "", "", "", "", "", ""], ["13", "Insulation Resistance Test", "", "", "", "", ""], ["13.1", "J3.B to Chassis", "> 1M", "-", "ohms", "", ""], ["13.2", "J1.16 to Chassis", "> 100K", "-", "ohms", "", ""], ["", "", "", "", "", "", ""], ["14", "Bonding Resistance", "", "", "", "", ""], ["14.1", "J1 Body to Chassis", "< 2m", "-", "ohms", "", ""], ["14.2", "J2  Body to Chassis", "< 2m", "-", "ohms", "", ""], ["14.3", "J3  Body to Chassis", "< 2m", "-", "ohms", "", ""], ["", "", "", "", "", "", ""], ["15", "CANbus Resistance Test", "", "", "", "", ""], ["15.1", "J1.17 to J1.18", "> 10K", "-", "ohms", "", ""], ["", "", "", "", "", "", ""], ["16", "Sealing Test", "N/A", "-", "", "", ""], ["", "", "", "", "", "", ""], ["17", "Mounting Holes Test - Jig Fit", "214", "-", "mm", "", ""]] ("ArrAHU 2") string[][] [["1", "Communication Test", "", "", "", "", ""], ["1.1", "Serial RS-232", "N/A", "-", "", "", ""], ["1.2", "CAN Bus", "N/A", "-", "", "", ""], ["", "", "", "", "", "", ""], ["2", "Auxiliary Fan Test", "", "", "", "", ""], ["2.1", "Fan status-ON", "ON", "-", "-", "", ""], ["2.2", "Fan status-OFF", "OFF", "-", "-", "", ""], ["", "", "", "", "", "", ""], ["3", "Temperature Sensor Calibration", "", "", "", "", ""], ["3.1", "Sensor Reading Analog Offset", "0", "+/-0.100", ".", "", ""], ["", "", "", "", "", "", ""], ["4", "Motor Termistor Input Test", "", "", "", "", ""], ["4.1", "60 Degree", "60", "+/-3.00", "°C", "", ""], ["4.2", "90 Degree", "90", "+/-3.00", "°C", "", ""], ["4.3", "120 Degree", "120", "+/-3.00", "°C", "", ""], ["", "", "", "", "", "", ""], ["5", "Enable Test", "", "", "", "", ""], ["5.1", "Fan Speed at Opened Enable ", "5000", "+/-200.0", "rpm", "", ""], ["5.2", "Fan Speed at Opened Enable ", "0", "+/-200.0", "rpm", "", ""], ["5.3", "Fan Speed at Closed Enable ", "5000", "+/-200.0", "rpm", "", ""], ["5.4", "Motor Rotation Direction", "CCW", "-", "", "", ""], ["", "", "", "", "", "", ""], ["6", "Speed Command Test", "", "", "", "", ""], ["6.1", "Fan  Speed", "11500", "+/-200.0", "rpm", "", ""], ["6.2", "Fan  Speed", "12700", "+/-200.0", "rpm", "", ""], ["6.3", "Fan  Speed", "14700", "+/-200.0", "rpm", "", ""], ["", "", "", "", "", "", ""], ["7", "Motor Stop time", "< 50", "-", "sec", "", ""], ["", "", "", "", "", "", ""], ["8", "Temperature Control Algorithm Test", "", "", "", "", ""], ["8.1", "Tair <   67 ± 3 °C", "11500", "+/-200.0", "rpm", "", ""], ["8.2", "Measured Temp.", "", "", "°C", "", ""], ["8.3", "Tair >= 67 ± 3 °C", "12700", "+/-200.0", "rpm", "", ""], ["8.4", "Transition Temp.", "", "", "°C", "", ""], ["8.5", "Tair >= 83 ± 3 °C", "14700", "+/-400.0", "rpm", "", ""], ["8.6", "Transition Temp.", "", "", "°C", "", ""], ["8.7", "Tair <= 80 ± 3 °C", "12700", "+/-200.0", "rpm", "", ""], ["8.8", "Transition Temp.", "", "", "°C", "", ""], ["8.9", "Tair <= 64 ± 3 °C", "11500", "+/-200.0", "rpm", "", ""], ["8.10", "Transition Temp.", "", "", "°C", "", ""], ["", "", "", "", "", "", ""], ["9", "Burn-in Test", "", "", "", "", ""], ["9.1", "DC Input Current", "45", "+/-5.000", "A", "", ""], ["9.2", "Fan speed", "14700", "+/-200.0", "rpm", "", ""], ["9.3", "Ambient Temperature", "25", "+/-13.00", "°C", "", ""], ["9.4", "After 10 min of operation", "", "-", "°C", "", ""], ["9.5", "After 20 min of operation", "", "-", "°C", "", ""], ["9.6", "After 30 min of operation", "", "-", "°C", "", ""], ["", "", "", "", "", "", ""], ["10", "Visual Inspection", "", "", "", "", ""], ["10.1", "Verification of Components Not Installed", "N/A", "-", "", "", ""], ["10.2", "Manufacturing Defects", "N/A", "-", "", "", ""], ["", "", "", "", "", "", ""], ["11", "Power Supply Testing", "", "", "", "", ""], ["11.1", "DC Input Current Drawn", "150", "+/-10.00", "mA", "", ""], ["", "", "", "", "", "", ""], ["12", "Power Supply Voltages", "", "", "", "", ""], ["12.1", "12V", "12.0", "+/-0.500", "V", "", ""], ["12.2", "5V", "5.0", "+/-0.200", "V", "", ""], ["12.3", "3.3V", "3.3", "+/-0.100", "V", "", ""], ["12.4", "1.8V", "1.8", "+/-0.100", "V", "", ""], ["", "", "", "", "", "", ""], ["13", "Reverse Polarity Test - DC Input Current", "< 1", "-", "mA", "", ""], ["", "", "", "", "", "", ""], ["14", "Functional Test Procedure", "", "", "", "", ""], ["14.1", "Weight Check", "4180", "+/-100.0", "gr", "", ""], ["", "", "", "", "", "", ""], ["15", "Insulation Resistance Test", "", "", "", "", ""], ["15.1", "J3.B to Chassis", "> 1M", "-", "ohms", "", ""], ["15.2", "J1.16 to Chassis", "> 100K", "-", "ohms", "", ""], ["", "", "", "", "", "", ""], ["16", "Bonding Resistance", "", "", "", "", ""], ["16.1", "J1 Body to Chassis", "< 2m", "-", "ohms", "", ""], ["16.2", "J2  Body to Chassis", "< 2m", "-", "ohms", "", ""], ["16.3", "J3  Body to Chassis", "< 2m", "-", "ohms", "", ""], ["", "", "", "", "", "", ""], ["17", "CANbus Resistance Test", "", "", "", "", ""], ["17.1", "J1.17 to J1.18", "> 10K", "-", "ohms", "", ""], ["", "", "", "", "", "", ""], ["18", "Sealing Test", "N/A", "-", "", "", ""], ["", "", "", "", "", "", ""], ["19", "Mounting Holes Test - Jig Fit", "214", "-", "mm", "", ""]] ("ArrEbay 3")] -> w2092
          tunnel: ["AHU" "EBAY"] -> w2091
          tunnel: [w2155 w2167] -> w2090
          tunnel: w2068 -> [w2156 w2167]
          tunnel: [w2151 u8 95] -> w2063
          frame False {
            (unwired) string[][] [["6.1", "Visual Inspection", "", "", "", "", ""], ["6.1.1", "Verification of Components Not Installed", "N/A", "-", "", "", ""], ["", "", "", "", "", "", ""], ["6.1.2", "Manufacturing Defects", "N/A", "-", "", "", ""], ["", "", "", "", "", "", ""], ["6.2", "Power Supply Testing", "", "", "", "", ""], ["6.2.1", "Input Current Drawn", "", "", "", "", ""], ["6.2.1.1", "DC Input Current", "< 150", "-", "mA", "", ""], ["", "", "", "", "", "", ""], ["6.2.2", "Power Supply Voltages", "", "", "", "", ""], ["6.2.2.1", "12V", "12.0", "+/-0.500", "V", "", ""], ["6.2.2.2", "5V", "5.0", "+/-0.200", "V", "", ""], ["6.2.2.3", "3.3V", "3.3", "+/-0.100", "V", "", ""], ["6.2.2.4", "1.8V", "1.8", "+/-0.100", "V", "", ""], ["", "", "", "", "", "", ""], ["7", "Functional Test Procedure", "", "", "", "", ""], ["7.1", "Weight Check", "3800", "+/-100.0", "gr", "", ""], ["", "", "", "", "", "", ""], ["7.2", "Insulation Resistance Test", "", "", "", "", ""], ["7.2.1", "J3.B to Chassis", "> 1M", "-", "W", "", ""], ["7.2.2", "J1.16 to Chassis", "> 100K", "-", "W", "", ""], ["", "", "", "", "", "", ""], ["7.2", "Bonding Resistance", "", "", "", "", ""], ["7.2.3", "J1 Body to Chassis", "< 2m", "-", "W", "", ""], ["7.2.4", "J2  Body to Chassis", "< 2m", "-", "W", "", ""], ["7.2.5", "J3  Body to Chassis", "< 2m", "-", "W", "", ""], ["", "", "", "", "", "", ""], ["7.2.1", "CANbus Resistance Test", "", "", "", "", ""], ["7.2.1.1", "J1.17 to J1.18", "> 10K", "-", "W", "", ""], ["", "", "", "", "", "", ""], ["7.3", "Sealing Test", "N/A", "-", "", "", ""], ["", "", "", "", "", "", ""], ["7.4", "Communication Test", "", "", "", "", ""], ["7.4.1", "Serial RS-232", "N/A", "-", "", "", ""], ["7.4.2", "CAN Bus", "N/A", "-", "", "", ""], ["", "", "", "", "", "", ""], ["7.5", "Performances Tests", "", "", "", "", ""], ["7.5.1", "Reverse Polarity Test", "", "", "", "", ""], ["7.5.1.1", "DC Input Current", "< 1", "-", "mA", "", ""], ["", "", "", "", "", "", ""], ["7.5.2", "Enable Test", "", "", "", "", ""], ["7.5.2.1", "Fan Speed at Opened Enable ", "5000", "+/-200.0", "rpm", "", ""], ["7.5.2.2", "Fan Speed at Opened Enable ", "0", "+/-200.0", "rpm", "", ""], ["7.5.2.3", "Fan Speed at Closed Enable ", "5000", "+/-200.0", "rpm", "", ""], ["7.5.2.4", "Motor Rotation Direction", "Counter-clockwise (Inlet)", "-", "", "", ""], ["", "", "", "", "", "", ""], ["7.5.3", "Stop Time Test ", "", "", "", "", ""], ["7.5.3.1", "Motor Stop time", "< 50", "-", "sec", "", ""], ["", "", "", "", "", "", ""], ["7.5.4", "Speed Command Test", "", "", "", "", ""], ["7.5.4.1", "Fan Speed", "6000", "+/-200.0", "rpm", "", ""], ["7.5.4.2", "Fan Speed", "9000", "+/-200.0", "rpm", "", ""], ["7.5.4.3", "Fan Speed", "12100", "+/-200.0", "rpm", "", ""], ["", "", "", "", "", "", ""], ["7.5.5", "Temperature Sensor Calibration Test", "", "", "", "", ""], ["7.5.5.1", "Sensor Reading Analog Offset", "0", "+/-0.100", ".", "", ""], ["", "", "", "", "", "", ""], ["7.5.6", "Burn-in Test", "", "", "", "", ""], ["7.5.6.1", "DC Input Current", "28", "+/-3.000", "A", "", ""], ["7.5.6.2", "Fan Speed", "12100", "+/-200.000", "rpm", "", ""], ["7.5.6.3", "Ambient Temperature", "25", "+/-13.00", "C", "", ""], ["7.5.6.4", "After 10 min of operation", "", "", "C", "", ""], ["7.5.6.5", "After 20 min of operation", "", "", "C", "", ""], ["7.5.6.6", "After 30 min of operation", "", "", "C", "", ""], ["", "", "", "", "", "", ""], ["9", "Motor Temp Test", "", "", "", "", ""], ["9.1", "60 C", "60", "+/-3.000", "C", "", ""], ["9.2", "90 C", "90", "+/-3.000", "C", "", ""], ["9.3", "120 C", "120", "+/-3.000", "C", "", ""]] ("data")
            n746 = while {
              shift-right: [w2163] -> w2155
              shift-left: w2156 -> [w2164]
              tunnel: [w2158] -> w2154
              stop <- w2162 stop-if-true
              n747 = call "AHU UUT (subVI).vi"("error in (no error)"=w2164) -> ("AHU 47"=w2159:bool, "AHU 63"=w2158:bool, "OK"=w2161:bool, "error out"=w2163:errorcluster)  [unwired: 15 in]
              n748 = Exclusive Or(1:w2159, 2:w2158) -> (0:w2160:bool)
              n749 = And(x=w2161, y=w2160) -> (x .and. y?=w2162:bool)
            }
            n750 = Select(t=u8 63, s=w2154, f=u8 47) -> (s? t:f=w2151:u8)
          }
          frame True {
            (unwired) string[][] [["1", "Communication Test", "", "", "", "", ""], ["1.1", "Serial RS-232", "N/A", "-", "", "", ""], ["1.2", "CAN Bus", "N/A", "-", "", "", ""], ["", "", "", "", "", "", ""], ["2", "Temperature Sensor Calibration", "", "", "", "", ""], ["2.1", "Sensor Reading Analog Offset", "0", "+/-0.100", ".", "", ""], ["", "", "", "", "", "", ""], ["3", "Motor Termistor Input Test", "", "", "", "", ""], ["3.1", "60 Degree", "60", "+/-3.00", "°C", "", ""], ["3.2", "90 Degree", "90", "+/-3.00", "°C", "", ""], ["3.3", "120 Degree", "120", "+/-3.00", "°C", "", ""], ["", "", "", "", "", "", ""], ["4", "Enable Test", "", "", "", "", ""], ["4.1", "Fan Speed at Opened Enable ", "5000", "+/-200.0", "rpm", "", ""], ["4.2", "Fan Speed at Opened Enable ", "0", "+/-200.0", "rpm", "", ""], ["4.3", "Fan Speed at Closed Enable ", "5000", "+/-200.0", "rpm", "", ""], ["4.4", "Motor Rotation Direction", "CCW", "-", "", "", ""], ["", "", "", "", "", "", ""], ["5", "Speed Command Test", "", "", "", "", ""], ["5.1", "Fan Speed", "11500", "+/-200.0", "rpm", "", ""], ["5.2", "Fan Speed", "12700", "+/-200.0", "rpm", "", ""], ["5.3", "Fan Speed", "14700", "+/-200.0", "rpm", "", ""], ["", "", "", "", "", "", ""], ["6", "Motor Stop time", "< 50", "-", "sec", "", ""], ["", "", "", "", "", "", ""], ["7", "Temperature Control Algorithm Test", "", "", "", "", ""], ["7.1", "Tair <   67 ± 3 °C", "11500", "+/-200.0", "rpm", "", ""], ["7.2", "Measured Temp.", "", "", "°C", "", ""], ["7.3", "Tair >= 67 ± 3 °C", "12700", "+/-200.0", "rpm", "", ""], ["7.4", "Transition Temp.", "", "", "°C", "", ""], ["7.5", "Tair >= 83 ± 3 °C", "14700", "+/-400.0", "rpm", "", ""], ["7.6", "Transition Temp.", "", "", "°C", "", ""], ["7.7", "Tair <= 80 ± 3 °C", "12700", "+/-200.0", "rpm", "", ""], ["7.8", "Transition Temp.", "", "", "°C", "", ""], ["7.9", "Tair <= 64 ± 3 °C", "11500", "+/-200.0", "rpm", "", ""], ["7.10", "Transition Temp.", "", "", "°C", "", ""], ["", "", "", "", "", "", ""], ["8", "Burn-in Test", "", "", "", "", ""], ["8.1", "DC Input Current", "50", "+/-5.000", "A", "", ""], ["8.2", "Fan Speed", "14700", "+/-200.0", "rpm", "", ""], ["8.3", "Ambient Temperature", "25", "+/-13.00", "°C", "", ""], ["8.4", "After 10 min of operation", "", "-", "°C", "", ""], ["8.5", "After 20 min of operation", "", "-", "°C", "", ""], ["8.6", "After 30 min of operation", "", "-", "°C", "", ""], ["", "", "", "", "", "", ""], ["9", "Auxiliary Fan Test", "", "", "", "", ""], ["9.1", "Fan status-ON", "ON", "-", "-", "", ""], ["9.2", "Fan status-OFF", "OFF", "-", "-", "", ""], ["", "", "", "", "", "", ""], ["10", "Visual Inspection", "", "", "", "", ""], ["10.1", "Verification of Components Not Installed", "N/A", "-", "", "", ""], ["10.2", "Manufacturing Defects", "N/A", "-", "", "", ""], ["", "", "", "", "", "", ""], ["11", "Power Supply Testing", "", "", "", "", ""], ["11.1", "DC Input Current Drawn", "150", "+/-10.00", "mA", "", ""], ["", "", "", "", "", "", ""], ["12", "Power Supply Voltages", "", "", "", "", ""], ["12.1", "12V", "12.0", "+/-0.500", "V", "", ""], ["12.2", "5V", "5.0", "+/-0.200", "V", "", ""], ["12.3", "3.3V", "3.3", "+/-0.100", "V", "", ""], ["12.4", "1.8V", "1.8", "+/-0.100", "V", "", ""], ["", "", "", "", "", "", ""], ["13", "Reverse Polarity Test - DC Input Current", "< 1", "-", "mA", "", ""], ["", "", "", "", "", "", ""], ["14", "Functional Test Procedure", "", "", "", "", ""], ["14.1", "Weight Check", "4180", "+/-100.0", "gr", "", ""], ["", "", "", "", "", "", ""], ["15", "Insulation Resistance Test", "", "", "", "", ""], ["15.1", "J3.B to Chassis", "> 1M", "-", "ohms", "", ""], ["15.2", "J1.16 to Chassis", "> 100K", "-", "ohms", "", ""], ["", "", "", "", "", "", ""], ["16", "Bonding Resistance", "", "", "", "", ""], ["16.1", "J1 Body to Chassis", "< 2m", "-", "ohms", "", ""], ["16.2", "J2  Body to Chassis", "< 2m", "-", "ohms", "", ""], ["16.3", "J3  Body to Chassis", "< 2m", "-", "ohms", "", ""], ["", "", "", "", "", "", ""], ["17", "CANbus Resistance Test", "", "", "", "", ""], ["17.1", "J1.17 to J1.18", "> 10K", "-", "ohms", "", ""], ["", "", "", "", "", "", ""], ["18", "Sealing Test", "N/A", "-", "", "", ""], ["", "", "", "", "", "", ""], ["19", "Mounting Holes Test - Jig Fit", "214", "-", "mm", "", ""]] ("ArrEbay 2")
          }
        }
        "UUT" <- w2091
        "UUT" <- w2063
        n751 = for {
          tunnel: w2092 -> [w2173] mode=indexing
          tunnel: w2090 -> [w2171]
          tunnel: [w2170] -> w2060
          tunnel: w2092 -> [w2169]
          i -> [w2172]
          n752 = for {
            tunnel: w2173 -> [_] mode=indexing
            tunnel: w2172 -> [w2179]
            tunnel: w2171 -> [w2176]
            tunnel: [w2175] -> w2170
            tunnel: w2169 -> [w2174]
            i -> [w2180]
            n753 = Bundle By Name(cluster=T22 {"Row"=0, "Column"=0} ("Active Cell:Active Cell"), "Row"=w2179, "Column"=w2180) -> (w2178:T22)
            n754 = control-ref of="ATR"() -> (w2177:refnum<vi>)
            n755 = property class="Tbl (strict)"(reference=w2177, error in=w2176, "Active Cell"=w2178, "Cell BG Color"=u32 16777226, "Value"=w2174) -> (error out=w2175:errorcluster)  [unwired: 1 out]
          }
        }
        n756 = case shown="95" w2063 {
          tunnel: ["AHU Software Version" ("key") "AHU Software Version" ("key") "EBAY Software Version" ("key")] -> w2080
          tunnel: ["AHU R Serial Number" ("key") "AHU L Serial Number" ("key") "EBAY Serial Number" ("key")] -> w2081
          tunnel: [2 2 1] -> w2065
          frame 63, Default {
          }
          frame 47 {
          }
          frame 95 {
          }
        }
        n757 = call <vilib>:"Open Config Data.vi"("error in (no error)"=w2060, "create file if necessary (T)"=FALSE, "configuration file path"=w2074) -> ("error out"=w2075:errorcluster, "refnum"=w2076:T12)  [unwired: 7 out]
        n758 = call-poly <vilib>:"Read Key.vi"("section"=w2078, "error in (no error)"=w2075, "key"=w2080, "refnum"=w2076) -> ("error out"=w2082:errorcluster, "value"=→"UUT SoftwareVer":string, "refnum out"=w2079:T12)  [unwired: 2 in, 3 out]
        n759 = property on="Start" class="Bool (strict)"("DisabledEnum"=w2066) -> ()  [unwired: 2 in, 2 out]
        n760 = property on="Report" class="Bool (strict)"("DisabledEnum"=w2066) -> ()  [unwired: 2 in, 2 out]
        n761 = call-poly <vilib>:"Read Key.vi"("section"=w2078, "error in (no error)"=w2082, "key"=w2081, "refnum"=w2079) -> ("error out"=w2072:errorcluster, "value"=w2070:string, "refnum out"=w2071:T12)  [unwired: 2 in, 3 out]
        n762 = call <vilib>:"Close Config Data.vi"("error in (no error)"=w2072, "refnum"=w2071) -> ("error out"=w2061:errorcluster)  [unwired: 8 in, 1 out]
        n763 = Decimal String To Number(string=w2070) -> (number=w2064:i32)  [unwired: 2 in, 1 out]
        n764 = case shown="47" w2063 {
          tunnel: w2064 -> [w2118 w2131 _]
          tunnel: [w2114 w2127 T11."MainProgram"] -> w2062
          tunnel: w2061 -> [w2113 w2126 w2139]
          tunnel: [w2113 w2126 w2139] -> w2059
          tunnel: [w2112 w2125 FALSE] -> w2057
          frame 63, Default {
            n765 = Quotient & Remainder(x=w2118, y=2) -> (x-y*floor(x/y)=w2116:i32)  [unwired: 1 out]
            n766 = Equal To 0?(x=w2116) -> (x = 0?=w2115:bool)
            n767 = case shown="True" w2115 {
              tunnel: [T11."MainProgram" w2122] -> w2114
              tunnel: [FALSE w2121] -> w2112
              frame False {
              }
              frame True {
                n768 = flat-sequence {
                  tunnel: [T11."Stop"] -> w2122
                  tunnel: [TRUE] -> w2121
                  frame #0 {
                    n769 = call "Display Message to User11"() -> ()  [unwired: 10 in, 2 out]
                  }
                  frame #1 {
                  }
                }
              }
            }
          }
          frame 47 {
            n770 = Quotient & Remainder(x=w2131, y=2) -> (x-y*floor(x/y)=w2129:i32)  [unwired: 1 out]
            n771 = Not Equal To 0?(x=w2129) -> (x != 0?=w2128:bool)
            n772 = case shown="True" w2128 {
              tunnel: [T11."MainProgram" w2135] -> w2127
              tunnel: [FALSE w2134] -> w2125
              frame False {
              }
              frame True {
                n773 = flat-sequence {
                  tunnel: [T11."Stop"] -> w2135
                  tunnel: [TRUE] -> w2134
                  frame #0 {
                    n774 = call "Display Message to User13"() -> ()  [unwired: 10 in, 2 out]
                  }
                  frame #1 {
                  }
                }
              }
            }
          }
          frame 95 {
          }
        }
        n775 = case shown="False" w2057 {
          tunnel: w2059 -> [w2103 w2111]
          tunnel: [w2102 w2111] -> w2058
          frame False {
            n776 = call "Boards S/N"("error in (no error)"=w2103) -> ("POWER Board S/N"=→"POWER Board S/N":string, "DSP Board S/N"=→"DSP Board S/N":string, "error out"=w2101:errorcluster)  [unwired: 15 in, 1 out]
            n777 = call "COM EvolutionBoard.vi"("error in (no error)"=w2101, "VISA resource name 2"=refnum<visa-resource-name> "COM1" ("VISA resource name")) -> ("error out"=w2109:errorcluster, "VISA resource name out"=w2108:refnum<visa-resource-name>)  [unwired: 8 in]
            n778 = call "TesterOption (SubVI).vi"("2 Options"=FALSE, "error in (no error)"=w2109, "On/Off"=FALSE, "Tester Option"=T13."Venable", "VISA Refnum in"=w2108) -> ("error out"=w2102:errorcluster, "VISA Refnum out"=→"VISA Tester":refnum<visa-resource-name>)  [unwired: 5 in]
          }
          frame True {
          }
        }
        n779 = Add(x=w2064, y=w2065) -> (x+y=→"Next SN":i32)
      }
      frame "Stop" {
        w2183 = 0
        n780 = flat-sequence {
          tunnel: w2216 -> [w2254]
          tunnel: [w2253] -> w2209
          frame #0 {
            n781 = control-ref of="Pannel User Message"() -> (w2256:refnum<vi>)
            n782 = property class="Str"(reference=w2256, error in=w2254, "Value"="Program Stopped...\r\nPlease turn OFF All Power sinks") -> (error out=w2253:errorcluster)  [unwired: 1 out]
          }
        }
        n783 = control-ref of="VISA Tester"() -> (w2217:refnum<vi>)
        n784 = property class="VISAName"(reference=w2217, error in=w2209) -> ("Value"=w2215:refnum<visa-resource-name>)  [unwired: 2 out]
        n785 = disable-structure shown="Enabled" {
          disable-tunnel: w2209 -> [w2241 w2242]
          disable-tunnel: w2208 -> [w2239 _]
          disable-tunnel: [w2238 w2242] -> w2195
          frame Disabled {
            n786 = call "Clear CAN Buffer.vi"("error in (no error)"=w2241, "Cluster in"=w2239) -> ("error out"=w2240:errorcluster)  [unwired: 8 in, 1 out]
            n787 = call "Close CAN Device.vi"("error in (no error)"=w2240, "Cluster in"=w2239) -> ("error out"=w2238:errorcluster)  [unwired: 8 in, 1 out]
          }
          frame Enabled {
          }
        }
        n788 = VISA Close(VISA resource name=w2224, error in (no error)=w2209) -> (error out=w2218:errorcluster)
        n789 = property on="Stop Button" class="Bool (strict)"() -> ("Value"=w2187:bool)  [unwired: 2 in, 2 out]
        n790 = call "TesterOption (SubVI).vi"("2 Options"=FALSE, "On/Off"=FALSE, "Tester Option"=T13."Power", "VISA Refnum in"=w2215) -> ("error out"=w2204:errorcluster, "VISA Refnum out"=w2214:refnum<visa-resource-name>)  [unwired: 6 in]
        n791 = property on="ClosePanel" class="Bool (strict)"() -> ("Value"=w2188:bool)  [unwired: 2 in, 2 out]
        n792 = VISA Close(VISA resource name=w2214, error in (no error)=w2204) -> (error out=w2201:errorcluster)
        n793 = Or(x=w2188, y=w2187) -> (x .or. y?=w2186:bool)
        n794 = Flush Queue(queue=w2219, error in (no error)=w2218) -> (queue out=w2221:refnum<queue>, error out=w2220:errorcluster)  [unwired: 1 out]
        n795 = Flush Queue(queue=w2226, error in (no error)=w2218) -> (queue out=w2225:refnum<queue>, error out=w2227:errorcluster)  [unwired: 1 out]
        n796 = case shown="False" w2186 {
          tunnel: w2227 -> [w2229 w2237]
          tunnel: w2225 -> [w2231 w2233]
          tunnel: w2221 -> [w2230 w2232]
          tunnel: w2220 -> [w2228 w2236]
          tunnel: [w2229 w2235] -> w2203
          tunnel: [w2228 w2234] -> w2202
          tunnel: [w2231 w2233] -> w2185
          tunnel: [w2230 w2232] -> w2184
          frame False {
          }
          frame True {
            n797 = Release Queue(queue=w2232, error in (no error)=w2236) -> (error out=w2234:errorcluster)  [unwired: 1 in, 2 out]
            n798 = Release Queue(queue=w2233, error in (no error)=w2237) -> (error out=w2235:errorcluster)  [unwired: 1 in, 2 out]
          }
        }
        n799 = Merge Errors(w2203, w2202, w2201, w2195) -> (w2200:errorcluster)
        n800 = property on="Refresh Button" class="Bool (strict)"() -> ("Value"=w2189:bool)  [unwired: 2 in, 2 out]
        n801 = call <vilib>:"Clear Errors.vi"("error in (no error)"=w2200) -> ("error out"=w2199:errorcluster)  [unwired: 5 in, 1 out]
        n802 = property on="Stop Button" class="Bool (strict)"() -> ("Value"=w2193:bool)  [unwired: 2 in, 2 out]
        n803 = property on="ClosePanel" class="Bool (strict)"(error in=w2199) -> (error out=w2197:errorcluster, "Value"=w2198:bool)  [unwired: 1 in, 1 out]
        n804 = Not(x=w2189) -> (.not. x?=w2190:bool)
        n805 = Select(t=T11."Initialize", s=w2189, f=T11."Stop") -> (s? t:f=w2205:T11)
        n806 = Not(x=w2193) -> (.not. x?=w2192:bool)
        n807 = Compound Arithmetic op=AND(w2198, w2192, w2190) -> (w2194:bool)
        n808 = case shown="False" w2194 {
          tunnel: w2197 -> [w2245 w2249]
          tunnel: [w2245 w2249] -> w2196
          tunnel: [w2244 w2248] -> w2191
          tunnel: w2189 -> [w2243 _]
          frame False {
            n809 = case shown="False" w2243 {
              tunnel: [TRUE FALSE] -> w2244
              frame False {
              }
              frame True {
              }
            }
          }
          frame True {
            n810 = flat-sequence {
              tunnel: [TRUE] -> w2248
              frame #0 {
              }
              frame #1 {
                n811 = control-ref of="This VI"() -> (w2252:refnum<vi>)
                n812 = property class="VI"(reference=w2252, "FP.State"=T23."Closed" ("Front Panel Window:State")) -> ()  [unwired: 1 in, 2 out]
              }
            }
          }
        }
      }
      frame "MainProgram" {
        n813 = event shown="[0] Timeout" {
          selector: w2267 -> [_ _ _ _ _ _ _ _ _ _ _ _ _]
          dyn-events: _ -> [_ _ _ _ _ _ _ _ _ _ _ _ _]
          timeout: 70 -> [_ _ _ _ _ _ _ _ _ _ _ _ _]
          tunnel: [T11."MainProgram" T11."MainProgram" T11."MainProgram" T11."MainProgram" T11."MainProgram" T11."Stop" T11."MainProgram" w2957 T11."MainProgram" T11."MainProgram" T11."MainProgram" T11."Stop" T11."MainProgram"] -> w2280
          tunnel: [w2287 w2433 w2505 w2514 w2525 w2545 w2572 w3005 w3076 w3091 w3103 w3191 w3199] -> w2274
          tunnel: w2278 -> [w2312 w2433 w2504 w2516 w2525 w2545 w2579 w3005 w3077 w3090 w3099 w3191 w3204]
          tunnel: [w2320 w2427 w2506 w2515 w2526 w2543 w2568 w2962 w3074 w3088 w3104 w3189 w3197] -> w2275
          tunnel: w2276 -> [w2320 w2427 w2506 w2515 w2526 w2543 w2568 w2962 w3074 w3088 _ w3189 w3197]
          tunnel: w2273 -> [w2314 w2439 w2500 w2511 w2522 w2542 w2577 w2989 w3073 w3087 w3107 w3188 w3202]
          tunnel: w2272 -> [w2310 w2438 w2501 w2512 w2523 w2541 w2550 w2988 w3072 w3086 w3106 w3187 w3195]
          tunnel: [w2311 w2438 w2501 w2512 w2523 w2541 w2550 w2988 w3072 w3086 w3106 w3187 w3195] -> w2271
          tunnel: [w2313 w2439 w2500 w2511 w2522 w2542 w2577 w2989 w3073 w3087 w3107 w3188 w3202] -> w2270
          tunnel: w2269 -> [w2308 w2437 w2499 w2510 w2521 w2540 w2576 w2987 w3071 w3085 w3105 w3186 w3201]
          tunnel: [w2308 w2437 w2499 w2510 w2521 w2540 w2571 w2987 w3071 w3085 w3105 w3186 w3201] -> w2268
          tunnel: w2266 -> [_ _ _ _ _ _ _ w2933 _ _ _ _ _]
          tunnel: w2265 -> [w2309 w2436 w2498 w2509 w2520 w2538 w2566 w2966 w3070 w3084 w3101 w3185 w3200]
          tunnel: [w2309 w2436 w2498 w2509 w2520 w2538 w2566 w2965 w3070 w3084 w3101 w3185 w3200] -> w2264
          tunnel: w2263 -> [_ w2434 _ _ _ _ _ w2964 _ _ _ _ _]
          tunnel: w2262 -> [_ w2426 _ _ _ _ _ _ _ _ _ _ _]
          tunnel: w2261 -> [_ _ _ _ _ _ _ _ w3069 _ _ _ _]
          tunnel: w2260 -> [w2284 w2407 w2497 w2508 w2519 w2535 w2549 w2935 w3067 w3083 w3096 w3184 w3193]
          tunnel: [w2283 w2407 w2497 w2508 w2519 w2535 w2549 w2935 w3067 w3083 w3096 w3184 w3193] -> w2259
          tunnel: w2258 -> [w2282 w2406 w2496 w2507 w2518 w2534 w2548 w2922 w3066 w3082 w3095 w3183 w3192]
          tunnel: [w2281 w2406 w2496 w2507 w2518 w2534 w2548 w2922 w3066 w3082 w3095 w3183 w3192] -> w2257
          event Timeout {
            n814 = event-data() -> ()  [unwired: 1 in, 3 out]
            n815 = property on="UUT" class="DigNum (strict)"() -> ("Value"=w2285:u8)  [unwired: 2 in, 2 out]
            n816 = property class="Clust (strict)"(reference=w2310, error in=w2312) -> (reference out=w2311:refnum<vi>, error out=w2286:errorcluster, "Value"=w2317:T8)
            n817 = case shown="95" w2285 {
              tunnel: w2286 -> [_ w2325]
              tunnel: w2284 -> [_ w2324]
              tunnel: [0 w2323] -> w2283
              frame 0, Default {
              }
              frame 95 {
                n818 = case shown="12" w2324 {
                  selector: w2324 -> [w2327 _]
                  tunnel: w2325 -> [_ w2331]
                  tunnel: [w2326 0] -> w2323
                  frame 0, Default {
                    n819 = Increment(x=w2327) -> (x+1=w2326:i32)
                  }
                  frame 12 {
                    n820 = property on="CurrentTest" class="Enum (strict)"() -> ("Value"=w2332:T1)  [unwired: 2 in, 2 out]
                    n821 = case shown="\"Temp Sens Cal\"" w2332 {
                      tunnel: [TRUE TRUE TRUE TRUE TRUE TRUE FALSE TRUE TRUE TRUE] -> w2330
                      tunnel: [u16 0 u16 0 u16 0 w2341 w2343 u16 0 u16 0 w2349 u16 0 u16 0] -> w2329
                      frame "Auxiliary", Default {
                      }
                      frame "Temp Sens Cal" {
                      }
                      frame "Com Test" {
                      }
                      frame "Enable Test" {
                        n822 = property on="VenableSpeed" class="DigNum (strict)"() -> ("Value"=w2341:u16)  [unwired: 2 in, 2 out]
                      }
                      frame "Speed Command" {
                        n823 = property on="SpeedCommandSpeed" class="DigNum (strict)"() -> ("Value"=w2343:u16)  [unwired: 2 in, 2 out]
                      }
                      frame "Stop Time" {
                      }
                      frame "Temp Control" {
                      }
                      frame "Burn in" {
                        n824 = property on="BurnInSpeed" class="DigNum (strict)"() -> ("Value"=w2349:u16)  [unwired: 2 in, 2 out]
                      }
                      frame "Visual Inspec" {
                      }
                      frame "Empty" {
                      }
                    }
                    n825 = control-ref of="Config_CANAT"() -> (w2334:refnum<vi>)
                    n826 = control-ref of="UUT"() -> (w2333:refnum<vi>)
                    n827 = call "CANSendMotorSpeed.vi"("Remote"=w2330, "error in (no error)"=w2331, "Motor Speed RPM"=w2329, "UUT"=w2333, "CAN Cluster in"=w2334) -> ()  [unwired: 6 in, 1 out]
                  }
                }
              }
            }
            n828 = Unbundle By Name(w2317) -> ("DevType"=w2318:T3, "CanIndex"=w2316:T2)
            n829 = property on="ClosePanel" class="Bool (strict)"("Value"=FALSE ("ClosePanel")) -> ()  [unwired: 2 in, 2 out]
            n830 = call "VCI_Receive.vi"("CANIndex"=w2316, "DevIndex"=u32 0, "DevType"=w2318) -> ("Recieve"=w2315:T26[])  [unwired: 3 in, 5 out]
            n831 = Empty Array?(array=w2315) -> (empty?=w2303:bool)
            n832 = case shown="False" w2303 {
              tunnel: w2316 -> [w2368 _]
              tunnel: w2311 -> [w2366 _]
              tunnel: w2314 -> [w2365 w2405]
              tunnel: w2286 -> [w2364 w2404]
              tunnel: w2315 -> [w2369 _]
              tunnel: [w2359 w2404] -> w2287
              tunnel: [w2358 w2405] -> w2313
              tunnel: [TRUE w2399] -> w2301
              tunnel: w2282 -> [_ w2403]
              tunnel: [0 w2402] -> w2281
              frame False {
                n833 = call "Demo_MakeDispBuff.vi"("Channel"=w2368, "Type"=enum16{"接收", "发送"}."接收", "OBJs"=w2369) -> ("Buffer"=w2367:T27)
                n834 = for {
                  N: 3 -> [_]
                  tunnel: w2367 -> [w2383]
                  tunnel: w2366 -> [w2382]
                  tunnel: w2365 -> [w2373]
                  tunnel: w2364 -> [w2372]
                  tunnel: [w2375] -> w2362 mode=indexing
                  tunnel: [w2373] -> w2361
                  tunnel: [w2372] -> w2360
                  i -> [w2371]
                  n835 = property class="Clust (strict)"(reference=w2382) -> ("Value"=w2380:T8)  [unwired: 1 in, 2 out]
                  n836 = Index Array(array=w2383, index=w2371) -> (element=w2376:T28)
                  n837 = Unbundle By Name(w2376) -> ("Channel"=w2378:T2, "VCI_CAN_OBJ"=w2381:T26)  [unwired: 2 out]
                  n838 = Unbundle By Name(w2380) -> ("CanIndex"=w2379:T2)
                  n839 = Equal?(x=w2379, y=w2378) -> (x = y?=w2377:bool)
                  n840 = case shown="True" w2377 {
                    tunnel: w2381 -> [_ w2394]
                    tunnel: [w2384 w2390] -> w2375
                    tunnel: T24 {"ID"=0, "MSGTYPE"=0, "LEN"=0, "aDATA"=[]} ("Msg") -> [w2384 w2389]
                    frame False {
                    }
                    frame True {
                      n841 = Unbundle By Name(w2394) -> ("ID"=w2388:u32, "DataLen"=w2393:u8, "Data"=w2391:u8[])
                      n842 = Bundle By Name(cluster=w2389, "ID"=w2388, "MSGTYPE"=u8 0, "LEN"=w2393, "aDATA"=w2391) -> (w2390:T24)
                      n843 = Unbundle By Name(w2390) -> ("ID"=w2386:u32)
                      n844 = Split Number(x=w2386) -> (lo(x)=w2387:u16)  [unwired: 1 out]
                      n845 = Split Number(x=w2387) -> (lo(x)=w2385:u8)  [unwired: 1 out]
                      n846 = case shown="63" w2385 {
                        tunnel: ["EBAY 5F" "" "AHU 3F" "AHU 2F"] -> _
                        frame 95 {
                        }
                        frame Default {
                        }
                        frame 63 {
                        }
                        frame 47 {
                        }
                      }
                    }
                  }
                }
                n847 = Enqueue Element(queue=w2361, element=w2362, error in (no error)=w2360) -> (queue out=w2358:refnum<queue>, error out=w2359:errorcluster)  [unwired: 2 out]
              }
              frame True {
                n848 = Increment(x=w2403) -> (x+1=w2402:i32)
                n849 = Greater Or Equal?(x=w2402, y=7) -> (x >= y?=w2400:bool)
                n850 = Not(x=w2400) -> (.not. x?=w2399:bool)
              }
            }
            n851 = property on="CAN Status" class="Bool (strict)"("Value"=w2301) -> ()  [unwired: 2 in, 2 out]
            n852 = control-ref of="ATR"() -> (w2302:refnum<vi>)
            n853 = call <vilib>:"Application Directory.vi"() -> ("Application Directory"=w2295:path)
            n854 = call "PassFailUUT (SubVI).vi"("error in (no error)"=w2287, "Table in"=w2302) -> ("PassFaileUUTresult"=w2291:bool)  [unwired: 7 in, 2 out]
            n855 = Select(t="PASS" ("name or relative path"), s=w2291, f="FAIL" ("name or relative path")) -> (s? t:f=w2288:string)
            n856 = Build Path(base path=w2295, name or relative path="data\\TestResult.ini") -> (appended path=w2299:path)
            n857 = property on="Test Failed" class="Bool (strict)"("Value"=w2291) -> ()  [unwired: 2 in, 2 out]
            n858 = call <vilib>:"Open Config Data.vi"("configuration file path"=w2299) -> ("error out"=w2297:errorcluster, "refnum"=w2298:T12)  [unwired: 2 in, 7 out]
            n859 = property on="Automation" class="Bool (strict)"() -> ("Value"=w2305:bool)  [unwired: 2 in, 2 out]
            n860 = call-poly <vilib>:"Write Key.vi"("section"="Marvin", "error in (no error)"=w2297, "value"=w2288, "key"="Result", "refnum"=w2298) -> ("error out"=w2294:errorcluster, "refnum out"=w2293:T12)  [unwired: 4 in, 1 out]
            n861 = property on="Start" class="Bool (strict)"() -> ("Value"=w2307:bool)  [unwired: 2 in, 2 out]
            n862 = Or(x=w2305, y=w2307) -> (x .or. y?=w2306:bool)
            n863 = call <vilib>:"Close Config Data.vi"("error in (no error)"=w2294, "refnum"=w2293) -> ()  [unwired: 8 in, 2 out]
            n864 = case shown="False" w2306 {
              frame False {
                n865 = property on="Pannel User Message" class="Str"("Value"="You can press start to execute(s) test(s).") -> ()  [unwired: 2 in, 2 out]
              }
              frame True {
              }
            }
          }
          event "SetSN": Value Change {
            n866 = event-data() -> ()  [unwired: 1 in, 6 out]
            n867 = property on="UUT" class="DigNum (strict)"() -> ("Value"=w2417:u8)  [unwired: 2 in, 2 out]
            n868 = Equal?(x=w2417, y=u8 95) -> (x = y?=w2415:bool)
            n869 = control-ref of="ATR"() -> (w2418:refnum<vi>)
            n870 = Select(t=u8 50 ("y"), s=w2415, f=u8 36 ("y")) -> (s? t:f=w2410:u8)
            n871 = property on="Current SN" class="DigNum (strict)"(error in=w2433) -> (error out=w2412:errorcluster, "Value"=w2432:i32)  [unwired: 1 in, 1 out]
            n872 = call "PassFailUUT (SubVI).vi"("error in (no error)"=w2412, "Table in"=w2418) -> ("Total Pass"=w2411:u8)  [unwired: 7 in, 2 out]
            n873 = Equal To 0?(x=w2432) -> (x = 0?=w2429:bool)
            n874 = Equal?(x=w2432, y=-1) -> (x = y?=w2430:bool)
            n875 = Equal?(x=w2411, y=w2410) -> (x = y?=w2409:bool)
            n876 = Or(x=w2430, y=w2429) -> (x .or. y?=w2428:bool)
            n877 = property on="CAN Status" class="Bool (strict)"() -> ("Value"=w2419:bool)  [unwired: 2 in, 2 out]
            n878 = property on="Status" class="Bool (strict)"() -> ("Value"=w2424:bool)  [unwired: 2 in, 2 out]
            n879 = And(x=w2424, y=w2419) -> (x .and. y?=w2420:bool)
            n880 = case shown="True" w2420 {
              tunnel: w2434 -> [_ w2453]
              tunnel: w2428 -> [_ w2442]
              tunnel: w2427 -> [_ w2452]
              tunnel: w2426 -> [_ w2451]
              tunnel: [errorcluster {"status"=FALSE, "code"=0, "source"=""} ("error out") w2450] -> w2423
              tunnel: [w2440 w2449] -> w2425
              tunnel: w2409 -> [_ w2443]
              frame False {
                w2440 = FALSE ("Value")
                n881 = property on="SetSN" class="Bool (strict)"("Value"=w2440) -> ()  [unwired: 2 in, 2 out]
                n882 = call "Display Message to User10"() -> ()  [unwired: 10 in, 2 out]
              }
              frame True {
                n883 = property on="Test Failed" class="Bool (strict)"() -> ("Value"=w2447:bool)  [unwired: 2 in, 2 out]
                n884 = property on="Automation" class="Bool (strict)"() -> ("Value"=w2449:bool)  [unwired: 2 in, 2 out]
                n885 = Not(x=w2447) -> (.not. x?=w2448:bool)
                n886 = Select(t=w2448, s=w2449, f=w2451) -> (s? t:f=w2445:bool)
                n887 = Or(x=w2443, y=w2445) -> (x .or. y?=w2444:bool)
                n888 = And(x=w2442, y=w2444) -> (x .and. y?=w2446:bool)
                n889 = case shown="True" w2446 {
                  tunnel: w2453 -> [_ w2484]
                  tunnel: w2452 -> [_ w2477]
                  tunnel: [w2455 w2469] -> w2450
                  tunnel: w2442 -> [w2454 _]
                  frame False {
                    n890 = case shown="True" w2454 {
                      tunnel: [w2457 w2458] -> w2455
                      frame False {
                        n891 = call "Display Message to User9"() -> ("error out"=w2457:errorcluster)  [unwired: 10 in, 1 out]
                      }
                      frame True {
                        n892 = call "Display Message to User3"() -> ("error out"=w2458:errorcluster)  [unwired: 10 in, 1 out]
                      }
                    }
                    n893 = property on="Automation" class="Bool (strict)"(error in=w2455, "Value"=FALSE ("Automation")) -> ()  [unwired: 1 in, 2 out]
                  }
                  frame True {
                    w2476 = FALSE ("SetSN")
                    n894 = property on="Next SN" class="DigNum (strict)"() -> ("Value"=w2460:i32)  [unwired: 2 in, 2 out]
                    n895 = property on="VISA Tester" class="VISAName"() -> ("Value"=w2467:refnum<visa-resource-name>)  [unwired: 2 in, 2 out]
                    n896 = call "TesterOption (SubVI).vi"("2 Options"=FALSE, "On/Off"=FALSE, "Tester Option"=T13."Venable", "VISA Refnum in"=w2467) -> ("error out"=w2462:errorcluster)  [unwired: 6 in, 1 out]
                    n897 = call <vilib>:"Clear Errors.vi"("error in (no error)"=w2462) -> ("error out"=w2463:errorcluster)  [unwired: 5 in, 1 out]
                    n898 = Number To Decimal String(number=w2460) -> (decimal integer string=w2461:string)  [unwired: 1 in]
                    "UUT SN Report" <- w2461
                    n899 = Search and Replace String(input string="EP=1\r\nSN=0\r\n" ("write buffer"), search string="0", replace string=w2461) -> (result string=w2479:string)  [unwired: 5 in, 3 out]
                    n900 = call "SerialMarvinSendGet.vi"("error in (no error)"=w2463, "Clear Log"=FALSE, "write buffer"=w2479, "VISA resource name"=w2477) -> ("error out"=w2468:errorcluster)  [unwired: 6 in, 1 out]
                    n901 = property on="UUT" class="DigNum (strict)"(error in=w2468) -> ("Value"=w2485:u8)  [unwired: 1 in, 2 out]
                    n902 = case shown="47" w2485 {
                      tunnel: ["AHU R Serial Number" ("key") "AHU L Serial Number" ("key") "EBAY Serial Number" ("key")] -> w2488
                      tunnel: [2 2 1] -> w2459
                      frame 63, Default {
                      }
                      frame 47 {
                      }
                      frame 95 {
                      }
                    }
                    n903 = call <vilib>:"Open Config Data.vi"("create file if necessary (T)"=FALSE, "configuration file path"=w2484) -> ("error out"=w2482:errorcluster, "refnum"=w2483:T12)  [unwired: 1 in, 7 out]
                    n904 = call-poly <vilib>:"Write Key.vi"("section"="Marvin", "error in (no error)"=w2482, "value"=w2461, "key"=w2488, "refnum"=w2483) -> ("error out"=w2472:errorcluster, "refnum out"=w2471:T12)  [unwired: 4 in, 1 out]
                    n905 = call <vilib>:"Close Config Data.vi"("error in (no error)"=w2472, "refnum"=w2471) -> ("error out"=w2470:errorcluster)  [unwired: 8 in, 1 out]
                    n906 = property on="Current SN" class="DigNum (strict)"("Value"=w2460) -> ()  [unwired: 2 in, 2 out]
                    n907 = property on="SetSN" class="Bool (strict)"(error in=w2470, "Value"=w2476) -> (error out=w2475:errorcluster)  [unwired: 1 in, 1 out]
                    n908 = property on="Automation" class="Bool (strict)"(error in=w2475, "Value"=w2476) -> (error out=w2474:errorcluster)  [unwired: 1 in, 1 out]
                    n909 = Add(x=w2460, y=w2459) -> (x+y=w2473:i32)
                    n910 = property on="Next SN" class="DigNum (strict)"(error in=w2474, "Value"=w2473) -> (error out=w2469:errorcluster)  [unwired: 1 in, 1 out]
                  }
                }
              }
            }
            n911 = call <vilib>:"Clear Errors.vi"("error in (no error)"=w2423) -> ("error out"=w2408:errorcluster)  [unwired: 5 in, 1 out]
            n912 = property on="SetSN" class="Bool (strict)"(error in=w2408, "Value"=FALSE ("SetSN")) -> (error out=w2422:errorcluster)  [unwired: 1 in, 1 out]
            n913 = case shown="True" w2425 {
              tunnel: w2422 -> [_ _]
              frame False {
              }
              frame True {
                w2495 = TRUE ("Value (Signaling)")
                n914 = property on="Report" class="Bool (strict)"("Val(Sgnl)"=w2495, "Value"=w2495) -> ()  [unwired: 2 in, 2 out]
              }
            }
          }
          event "ATR": Mouse Enter {
            n915 = event-data() -> ()  [unwired: 1 in, 4 out]
            n916 = call-poly <vilib>:"Set Cursor.vi"("error in (no error)"=w2504, "icon"=u16 1) -> ("error out"=w2505:errorcluster)  [unwired: 8 in, 1 out]
          }
          event "ATR": Mouse Leave {
            n917 = event-data() -> ()  [unwired: 1 in, 4 out]
            n918 = call-poly <vilib>:"Set Cursor.vi"("error in (no error)"=w2516, "icon"=u16 0) -> ("error out"=w2514:errorcluster)  [unwired: 8 in, 1 out]
          }
          event "ATR": Mouse Down? {
            n919 = event-data() -> ("Coords"=w2533:T29)  [unwired: 1 in, 4 out]
            n920 = invoke on="ATR" class="Tbl (strict)" method="Point To Row Column"("Point"=w2533) -> ("InBounds"=w2529:bool, "CellPosition"=w2528:T22)  [unwired: 5 in, 4 out]
            n921 = Greater Than 0?(x=w2528) -> (x > 0?=w2532:cluster{"Row":bool, "Column":bool})
            n922 = Cluster To Array(cluster=w2532) -> (array=w2531:bool[])
            n923 = Or Array Elements(Boolean array=w2531) -> (logical OR=w2530:bool)
            n924 = Or(x=w2529, y=w2530) -> (x .or. y?=w2527:bool)
            n925 = event-data("Discard?"=w2527) -> ()  [unwired: 1 in, 1 out]
          }
          event Panel Close? {
            n926 = event-data() -> ("VIRef"=w2539:refnum<vi>)  [unwired: 1 in, 3 out]
            n927 = Close Reference(reference=w2539) -> ()  [unwired: 1 in, 1 out]
            n928 = disable-structure shown="Disabled" {
              frame Disabled {
                n929 = property on="Stop Button" class="Bool (strict)"("Val(Sgnl)"=TRUE ("Stop Button"), "Value"=FALSE ("Stop Button")) -> ()  [unwired: 2 in, 2 out]
              }
              frame Enabled {
              }
            }
            n930 = event-data("Discard?"=TRUE) -> ()  [unwired: 1 in, 1 out]
            "ClosePanel" <- TRUE ("ClosePanel")
          }
          event "Start": Value Change {
            w2567 = T18 [] items=["Auxiliary", "Temp Sens Cal", "Com Test", "Enable Test", "Speed Command", "Stop Time", "Temp Control", "Burn in", "Visual Inspec", "Empty"]
            n931 = event-data() -> ()  [unwired: 1 in, 2 out]
            n932 = property on="VISA Tester" class="VISAName"() -> ("Value"=w2565:refnum<visa-resource-name>)  [unwired: 2 in, 2 out]
            n933 = property on="UUT" class="Str"(error in=w2579) -> (error out=w2561:errorcluster, "Value"=w2578:string)  [unwired: 1 in, 1 out]
            n934 = control-ref of="Pannel User Message"() -> (w2558:refnum<vi>)
            n935 = control-ref of="Motor Speed RPM"() -> (w2553:refnum<vi>)
            n936 = call "TesterOption (SubVI).vi"("2 Options"=FALSE, "error in (no error)"=w2561, "On/Off"=FALSE, "Tester Option"=T13."Venable", "VISA Refnum in"=w2565) -> ("error out"=w2560:errorcluster)  [unwired: 5 in, 1 out]
            n937 = control-ref of="Stop Burn-in"() -> (w2556:refnum<vi>)
            n938 = control-ref of="Stop Button"() -> (w2557:refnum<vi>)
            n939 = call "Write panel message (SubVI).vi"("Stop BurnIn"=w2556, 4:"rpm"=w2553, 5:"rpm"=FALSE ("rpm"), "PrintTime"=TRUE, "Stop"=w2557, "error in (no error)"=w2560, "Time to wait"=5.0, "Strin"="TESTER BIT TEST OPERATION IN PROCESS", "String in"=w2558) -> ("error out"=w2559:errorcluster)  [unwired: 2 in]
            n940 = while {
              tunnel: w2578 -> [w2607]
              tunnel: [w2606] -> w2574
              tunnel: [w2605] -> w2573
              shift-right: [w2602] -> _
              shift-left: enum16{"Stop", "Tests", "Bit test", "Start"}."Start" -> [w2604]
              tunnel: w2568 -> [w2603]
              tunnel: w2567 -> [w2601]
              tunnel: w2559 -> [w2586]
              tunnel: w2557 -> [w2595]
              tunnel: w2556 -> [w2594]
              tunnel: w2558 -> [w2593]
              tunnel: w2553 -> [w2592]
              tunnel: w2550 -> [w2585]
              stop <- w2600 stop-if-true
              n941 = property class="Clust (strict)"(reference=w2585, error in=w2586) -> ("Value"=w2588:T8)  [unwired: 2 out]
              n942 = Unbundle By Name(w2588) -> ("DevType"=w2590:T3, "CanIndex"=w2589:T2)
              n943 = property on="VISA Tester" class="VISAName"() -> ("Value"=w2598:refnum<visa-resource-name>)  [unwired: 2 in, 2 out]
              n944 = call "VCI_Receive.vi"("CANIndex"=w2589, "DevIndex"=u32 0, "DevType"=w2590) -> ("Recieve"=w2591:T26[])  [unwired: 3 in, 5 out]
              n945 = Empty Array?(array=w2591) -> (empty?=w2584:bool)
              n946 = Not(x=w2584) -> (.not. x?=w2583:bool)
              n947 = property on="CAN Status" class="Bool (strict)"("Value"=w2583) -> (error out=w2582:errorcluster)  [unwired: 2 in, 1 out]
              n948 = property on="CAN Status" class="Bool (strict)"(error in=w2582) -> (error out=w2581:errorcluster, "Value"=w2596:bool)  [unwired: 1 in, 1 out]
              n949 = property on="Status" class="Bool (strict)"(error in=w2581) -> (error out=w2597:errorcluster, "Value"=w2599:bool)  [unwired: 1 in, 1 out]
              n950 = case shown="\"Start\"" w2604 {
                tunnel: w2607 -> [_ w2623 w2756 _]
                tunnel: [w2612 w2622 w2780 w2888] -> w2606
                tunnel: [w2608 w2621 w2754 w2880] -> w2605
                tunnel: w2603 -> [_ _ w2767 w2893]
                tunnel: w2593 -> [_ _ _ w2892]
                tunnel: w2595 -> [_ _ _ w2891]
                tunnel: w2594 -> [_ _ _ w2890]
                tunnel: w2592 -> [_ _ _ w2889]
                tunnel: [w2611 w2620 w2759 w2884] -> w2602
                tunnel: w2601 -> [w2612 _ w2780 w2888]
                tunnel: [w2610 w2619 FALSE FALSE] -> w2600
                tunnel: w2599 -> [_ _ _ w2886]
                tunnel: w2598 -> [_ _ w2750 _]
                tunnel: w2597 -> [w2608 _ _ _]
                tunnel: w2596 -> [_ _ _ w2881]
                frame "Stop", Default {
                  n951 = property on="Start" class="Bool (strict)"(error in=w2608, "Value"=FALSE ("Start")) -> ()  [unwired: 1 in, 2 out]
                  n952 = flat-sequence {
                    tunnel: [enum16{"Stop", "Tests", "Bit test", "Start"}."Stop"] -> w2611
                    tunnel: w2608 -> [_]
                    tunnel: [TRUE] -> w2610
                    frame #0 {
                    }
                  }
                }
                frame "Tests" {
                  w2617 = FALSE ("Stop Burn-in")
                  w2618 = T21."Disabled and Grayed Out" ("Disabled")
                  n953 = case shown="\"EBAY\"" w2623 {
                    tunnel: [w2639 w2688] -> w2622
                    tunnel: [w2638 w2687] -> w2621
                    tunnel: [w2627 w2675] -> w2615
                    frame "AHU", Default {
                      n954 = call "Load Program Process AHU.vi"() -> ("Speed Command Test"=w2632:bool, "Enable Test"=w2633:bool, "Burn-in Test"=w2630:bool, "Auxiliary"=w2628:bool, "Temperature Sensor Calibration Test"=w2635:bool, "Communication Test"=w2634:bool, "Stop Time Test"=w2631:bool, "Visual Inspection"=w2629:bool, "OK"=w2636:bool, "Automation"=w2627:bool, "error out"=w2638:errorcluster)  [unwired: 8 in, 9 out]
                      n955 = Or(x=w2636, y=w2627) -> (x .or. y?=w2637:bool)
                      n956 = case shown="True" w2637 {
                        tunnel: [w2640 w2650] -> w2639
                        tunnel: w2627 -> [_ w2649]
                        tunnel: w2635 -> [_ w2648]
                        tunnel: w2634 -> [_ w2647]
                        tunnel: w2633 -> [_ w2646]
                        tunnel: w2632 -> [_ w2645]
                        tunnel: w2631 -> [_ w2644]
                        tunnel: w2630 -> [_ w2643]
                        tunnel: w2629 -> [_ w2642]
                        tunnel: w2628 -> [_ w2641]
                        frame False {
                          w2640 = T18 [] items=["Auxiliary", "Temp Sens Cal", "Com Test", "Enable Test", "Speed Command", "Stop Time", "Temp Control", "Burn in", "Visual Inspec", "Empty"]
                        }
                        frame True {
                          n957 = case shown="False" w2649 {
                            tunnel: [w2673 w2674] -> w2650
                            tunnel: w2648 -> [w2655 _]
                            tunnel: w2647 -> [w2654 _]
                            tunnel: w2646 -> [w2656 _]
                            tunnel: w2645 -> [w2653 _]
                            tunnel: w2644 -> [w2652 _]
                            tunnel: w2643 -> [w2666 _]
                            tunnel: w2642 -> [w2651 _]
                            tunnel: w2641 -> [_ _]
                            frame False {
                              w2659 = T1."Empty" ("f")
                              n958 = Select(t=T1."Com Test" ("f"), s=w2654, f=w2659) -> (s? t:f=w2665:T1)
                              n959 = Select(t=T1."Temp Sens Cal" ("f"), s=w2655, f=w2659) -> (s? t:f=w2664:T1)
                              n960 = Select(t=T1."Stop Time" ("f"), s=w2652, f=w2659) -> (s? t:f=w2663:T1)
                              n961 = Select(t=T1."Enable Test" ("f"), s=w2656, f=w2659) -> (s? t:f=w2662:T1)
                              n962 = Select(t=T1."Speed Command" ("f"), s=w2653, f=w2659) -> (s? t:f=w2661:T1)
                              n963 = Select(t=T1."Burn in" ("f"), s=w2666, f=w2659) -> (s? t:f=w2660:T1)
                              n964 = Select(t=T1."Visual Inspec" ("f"), s=w2651, f=w2659) -> (s? t:f=w2657:T1)
                              n965 = Build Array(w2665, w2664, w2663, w2662, w2661, w2660, w2657) -> (w2673:T18)
                            }
                            frame True {
                              w2674 = T18 [enum."Com Test", enum."Temp Sens Cal", enum."Stop Time", enum."Enable Test", enum."Speed Command", enum."Burn in", enum."Visual Inspec"] items=["Auxiliary", "Temp Sens Cal", "Com Test", "Enable Test", "Speed Command", "Stop Time", "Temp Control", "Burn in", "Visual Inspec", "Empty"]
                            }
                          }
                        }
                      }
                    }
                    frame "EBAY" {
                      n966 = call "Load Program Process EBAY.vi"() -> ("Speed Command Test"=w2681:bool, "Enable Test"=w2682:bool, "Burn-in Test"=w2679:bool, "Temperature Control Algorithm Test"=w2678:bool, "Auxiliary"=w2676:bool, "Temperature Sensor Calibration Test"=w2684:bool, "Communication Test"=w2683:bool, "Stop Time Test"=w2680:bool, "Visual Inspection"=w2677:bool, "OK"=w2685:bool, "Automation"=w2675:bool, "error out"=w2687:errorcluster)  [unwired: 8 in, 8 out]
                      n967 = Or(x=w2685, y=w2675) -> (x .or. y?=w2686:bool)
                      n968 = case shown="True" w2686 {
                        tunnel: [w2689 w2700] -> w2688
                        tunnel: w2675 -> [_ w2699]
                        tunnel: w2684 -> [_ w2698]
                        tunnel: w2683 -> [_ w2697]
                        tunnel: w2682 -> [_ w2696]
                        tunnel: w2681 -> [_ w2695]
                        tunnel: w2680 -> [_ w2694]
                        tunnel: w2679 -> [_ w2693]
                        tunnel: w2678 -> [_ w2692]
                        tunnel: w2677 -> [_ w2691]
                        tunnel: w2676 -> [_ w2690]
                        frame False {
                          w2689 = T18 [] items=["Auxiliary", "Temp Sens Cal", "Com Test", "Enable Test", "Speed Command", "Stop Time", "Temp Control", "Burn in", "Visual Inspec", "Empty"]
                        }
                        frame True {
                          n969 = case shown="False" w2699 {
                            tunnel: [w2729 w2730] -> w2700
                            tunnel: w2698 -> [w2706 _]
                            tunnel: w2697 -> [w2705 _]
                            tunnel: w2696 -> [w2704 _]
                            tunnel: w2695 -> [w2703 _]
                            tunnel: w2694 -> [w2702 _]
                            tunnel: w2693 -> [w2708 _]
                            tunnel: w2692 -> [w2707 _]
                            tunnel: w2691 -> [w2720 _]
                            tunnel: w2690 -> [w2711 _]
                            frame False {
                              w2709 = T1."Empty" ("f")
                              n970 = Select(t=T1."Com Test" ("f"), s=w2705, f=w2709) -> (s? t:f=w2719:T1)
                              n971 = Select(t=T1."Temp Sens Cal" ("f"), s=w2706, f=w2709) -> (s? t:f=w2718:T1)
                              n972 = Select(t=T1."Stop Time" ("f"), s=w2702, f=w2709) -> (s? t:f=w2717:T1)
                              n973 = Select(t=T1."Enable Test" ("f"), s=w2704, f=w2709) -> (s? t:f=w2716:T1)
                              n974 = Select(t=T1."Speed Command" ("f"), s=w2703, f=w2709) -> (s? t:f=w2715:T1)
                              n975 = Select(t=T1."Temp Control" ("f"), s=w2707, f=w2709) -> (s? t:f=w2714:T1)
                              n976 = Select(t=T1."Burn in" ("f"), s=w2708, f=w2709) -> (s? t:f=w2713:T1)
                              n977 = Select(t=T1."Visual Inspec" ("f"), s=w2720, f=w2709) -> (s? t:f=w2712:T1)
                              n978 = Select(t=T1."Auxiliary" ("f"), s=w2711, f=w2709) -> (s? t:f=w2701:T1)
                              n979 = Build Array(w2719, w2701, w2718, w2717, w2716, w2715, w2714, w2713, w2712) -> (w2729:T18)
                            }
                            frame True {
                              w2730 = T18 [enum."Com Test", enum."Auxiliary", enum."Temp Sens Cal", enum."Stop Time", enum."Enable Test", enum."Speed Command", enum."Temp Control", enum."Burn in", enum."Visual Inspec"] items=["Auxiliary", "Temp Sens Cal", "Com Test", "Enable Test", "Speed Command", "Stop Time", "Temp Control", "Burn in", "Visual Inspec", "Empty"]
                            }
                          }
                        }
                      }
                    }
                  }
                  "Automation" <- w2615
                  n980 = control-ref of="ATR"() -> (w2616:refnum<vi>)
                  n981 = flat-sequence {
                    tunnel: [enum16{"Stop", "Tests", "Bit test", "Start"}."Tests"] -> w2620
                    tunnel: [TRUE] -> w2619
                    frame #0 {
                    }
                  }
                  n982 = case shown="True" w2615 {
                    tunnel: w2616 -> [_ w2624]
                    frame False {
                    }
                    frame True {
                      n983 = call "ResetTable Result (SubVI).vi"("Table in"=w2624) -> ()  [unwired: 11 in]
                    }
                  }
                  n984 = property on="Stop Button" class="Bool (strict)"("Value"=w2617) -> ()  [unwired: 2 in, 2 out]
                  n985 = property on="Stop Burn-in" class="Bool (strict)"("Value"=w2617) -> ()  [unwired: 2 in, 2 out]
                  n986 = property on="Start" class="Bool (strict)"("DisabledEnum"=w2618) -> ()  [unwired: 2 in, 2 out]
                  n987 = property on="Report" class="Bool (strict)"("DisabledEnum"=w2618) -> ()  [unwired: 2 in, 2 out]
                }
                frame "Bit test" {
                  # "Stop"
                  n988 = call "SerialMarvinSendGet.vi"("write buffer"="TA[1]\r\n", "VISA resource name"=w2767) -> ("error out"=w2741:errorcluster, "read buffer"=w2777:string)  [unwired: 8 in]
                  n989 = Fract/Exp String To Number(string=w2777) -> (number=w2740:dbl)  [unwired: 3 in, 1 out]
                  n990 = call "TAs StartTest (SubVI).vi"("error in"=w2741, "Numeric"=w2740, "Enum"=enum16{"TA3", "TA2", "TA1"}."TA1") -> ("error out"=w2739:errorcluster, "String Out"=w2738:string, "Result"=w2737:bool)  [unwired: 6 in]
                  n991 = call "TesterOption (SubVI).vi"("On/Off 2"=FALSE, "Tester Option 2"=T13."Venable", "2 Options"=TRUE, "error in (no error)"=w2739, "On/Off"=TRUE, "Tester Option"=T13."25C", "VISA Refnum in"=w2750) -> ("error out"=w2769:errorcluster)  [unwired: 3 in, 1 out]
                  n992 = call "Time Delay5"("error in (no error)"=w2769) -> ("error out"=w2768:errorcluster)  [unwired: 10 in]
                  n993 = call "SerialMarvinSendGet.vi"("error in (no error)"=w2768, "write buffer"="TA[2]\r\n", "VISA resource name"=w2767) -> ("error out"=w2735:errorcluster, "read buffer"=w2771:string)  [unwired: 7 in]
                  n994 = Fract/Exp String To Number(string=w2771) -> (number=w2734:dbl)  [unwired: 3 in, 1 out]
                  n995 = call "TAs StartTest (SubVI).vi"("error in"=w2735, "Numeric"=w2734, "Enum"=enum16{"TA3", "TA2", "TA1"}."TA2") -> ("error out"=w2733:errorcluster, "String Out"=w2732:string, "Result"=w2731:bool)  [unwired: 6 in]
                  n996 = call "GetADCTester (SubVI).vi"("error in (no error)"=w2733, "GetADCTester"=T15."Term1", "TimeToGet"=5, "VISA Refnum in"=w2750) -> ("error out"=w2749:errorcluster, "ADCValOutput Single"=w2747:dbl)  [unwired: 5 in, 1 out]
                  n997 = case shown="\"EBAY\"" w2756 {
                    tunnel: w2750 -> [w2810 _ w2842]
                    tunnel: w2767 -> [_ _ w2845]
                    tunnel: w2749 -> [w2811 w2828 w2844]
                    tunnel: [w2804 w2828 w2841] -> w2758
                    tunnel: [w2801 "" w2838] -> w2764
                    tunnel: [w2800 bool[] [] w2837] -> w2748
                    frame "AHU" {
                      n998 = call "TesterOption (SubVI).vi"("On/Off 2"=FALSE, "Tester Option 2"=T13."Venable", "2 Options"=TRUE, "error in (no error)"=w2811, "On/Off"=TRUE, "Tester Option"=T13."K17", "VISA Refnum in"=w2810) -> ("error out"=w2813:errorcluster)  [unwired: 3 in, 1 out]
                      n999 = call "Time Delay7"("error in (no error)"=w2813) -> ("error out"=w2812:errorcluster)  [unwired: 10 in]
                      n1000 = call "GetADCTester (SubVI).vi"("error in (no error)"=w2812, "GetADCTester"=T15."Current", "TimeToGet"=5, "VISA Refnum in"=w2810) -> ("error out"=w2804:errorcluster, "ADCValOutput Single"=w2806:dbl)  [unwired: 5 in, 1 out]
                      n1001 = Less Or Equal?(x=w2806, y=10.0) -> (x <= y?=w2805:bool)
                      n1002 = Build Array(w2805) -> (w2800:bool[])
                      n1003 = for {
                        tunnel: w2800 -> [w2825] mode=indexing
                        tunnel: string[] ["Current sensor not connected!"] -> [w2822] mode=indexing
                        shift-right: [w2823] -> w2801
                        shift-left: "" -> [w2820]
                        n1004 = Concatenate Strings(w2822, "\r\n") -> (w2819:string)
                        n1005 = Select(t=w2820, s=w2825, f=w2819) -> (s? t:f=w2824:string)
                        n1006 = Concatenate Strings(w2820, w2824) -> (w2823:string)
                      }
                    }
                    frame Default {
                    }
                    frame "EBAY" {
                      w2843 = T30 [enum."Fan", enum."Current"] items=["Term1", "Term2", "Current", "Fan", "TempCPU"]
                      n1007 = call "TesterOption (SubVI).vi"("On/Off 2"=FALSE, "Tester Option 2"=T13."Venable", "2 Options"=TRUE, "error in (no error)"=w2844, "On/Off"=TRUE, "Tester Option"=T13."K17", "VISA Refnum in"=w2842) -> ("error out"=w2847:errorcluster)  [unwired: 3 in, 1 out]
                      n1008 = call "Time Delay6"("error in (no error)"=w2847) -> ("error out"=w2846:errorcluster)  [unwired: 10 in]
                      n1009 = call "SerialMarvinSendGet.vi"("error in (no error)"=w2846, "write buffer"="TA[3]\r\n", "VISA resource name"=w2845) -> ("error out"=w2832:errorcluster, "read buffer"=w2849:string)  [unwired: 7 in]
                      n1010 = Fract/Exp String To Number(string=w2849) -> (number=w2833:dbl)  [unwired: 3 in, 1 out]
                      n1011 = call "TAs StartTest (SubVI).vi"("error in"=w2832, "Numeric"=w2833, "Enum"=enum16{"TA3", "TA2", "TA1"}."TA3") -> ("error out"=w2829:errorcluster, "String Out"=w2831:string, "Result"=w2830:bool)  [unwired: 6 in]
                      n1012 = for {
                        tunnel: w2843 -> [w2872] mode=indexing
                        tunnel: w2842 -> [w2871]
                        tunnel: w2829 -> [w2869]
                        tunnel: [w2868] -> w2841
                        tunnel: [w2865] -> w2840 mode=indexing
                        i -> [w2866]
                        n1013 = call "GetADCTester (SubVI).vi"("error in (no error)"=w2869, "GetADCTester"=w2872, "TimeToGet"=5, "VISA Refnum in"=w2871) -> ("error out"=w2868:errorcluster, "ADCValOutput Single"=w2867:dbl)  [unwired: 5 in, 1 out]
                        n1014 = case shown="1" w2866 {
                          tunnel: w2867 -> [w2875 w2878 _]
                          tunnel: [w2873 w2876 FALSE] -> w2865
                          frame 1 {
                            n1015 = Less Or Equal?(x=w2875, y=10.0) -> (x <= y?=w2873:bool)
                          }
                          frame 0 {
                            n1016 = Greater Or Equal?(x=w2878, y=2200.0) -> (x >= y?=w2876:bool)
                          }
                          frame Default {
                          }
                        }
                      }
                      n1017 = Build Array (concatenate)(w2830, w2840) -> (w2837:bool[])
                      n1018 = Build Array (concatenate)(w2831, string[] ["AUX Fan not connected!", "Current sensor not connected!"]) -> (w2835:string[])
                      n1019 = for {
                        tunnel: w2837 -> [w2855] mode=indexing
                        tunnel: w2835 -> [w2858] mode=indexing
                        shift-right: [w2860] -> w2838
                        shift-left: "" -> [w2859]
                        n1020 = Concatenate Strings(w2858, "\r\n") -> (w2856:string)
                        n1021 = case shown="False" w2855 {
                          tunnel: [w2863 w2864] -> w2860
                          tunnel: w2859 -> [w2862 w2864]
                          tunnel: w2856 -> [w2861 _]
                          frame False {
                            n1022 = Concatenate Strings(w2862, w2861) -> (w2863:string)
                          }
                          frame True {
                          }
                        }
                      }
                    }
                  }
                  n1023 = Less Or Equal?(x=w2747, y=100.0) -> (x <= y?=w2745:bool)
                  n1024 = Build Array(w2738, w2732, "Failure - check 28V or GND signals. Pin28 or Pin2") -> (w2744:string[])
                  n1025 = Build Array(w2737, w2731, w2745) -> (w2763:bool[])
                  n1026 = for {
                    tunnel: w2763 -> [w2789] mode=indexing
                    tunnel: w2744 -> [w2793] mode=indexing
                    shift-right: [w2795] -> w2765
                    shift-left: "" -> [w2794]
                    tunnel: w2758 -> [w2790]
                    tunnel: [w2790] -> w2757
                    n1027 = Concatenate Strings(w2793, "\r\n") -> (w2791:string)
                    n1028 = case shown="False" w2789 {
                      tunnel: [w2798 w2799] -> w2795
                      tunnel: w2794 -> [w2797 w2799]
                      tunnel: w2791 -> [w2796 _]
                      frame False {
                        n1029 = Concatenate Strings(w2797, w2796) -> (w2798:string)
                      }
                      frame True {
                      }
                    }
                  }
                  n1030 = Build Array (concatenate)(w2763, w2748) -> (w2762:bool[])
                  n1031 = And Array Elements(Boolean array=w2762) -> (logical AND=w2753:bool)
                  n1032 = case shown="False" w2753 {
                    tunnel: w2765 -> [w2787 _]
                    tunnel: w2764 -> [w2786 _]
                    tunnel: w2757 -> [w2784 w2788]
                    tunnel: [w2784 w2788] -> w2755
                    frame False {
                      n1033 = Concatenate Strings(w2787, w2786) -> (w2785:string)
                      n1034 = One Button Dialog(message=w2785) -> ()  [unwired: 1 in, 1 out]
                    }
                    frame True {
                    }
                  }
                  n1035 = case shown="False" w2753 {
                    tunnel: w2755 -> [w2782 w2783]
                    tunnel: [w2781 w2783] -> w2754
                    frame False {
                      n1036 = call "Display Message to User6"("error in (no error)"=w2782) -> ("error out"=w2781:errorcluster)  [unwired: 9 in, 1 out]
                    }
                    frame True {
                    }
                  }
                  n1037 = Select(t=enum16{"Stop", "Tests", "Bit test", "Start"}."Tests", s=w2753, f=enum16{"Stop", "Tests", "Bit test", "Start"}."Stop") -> (s? t:f=w2759:enum16{"Stop", "Tests", "Bit test", "Start"})
                }
                frame "Start" {
                  n1038 = And(x=w2881, y=w2886) -> (x .and. y?=w2882:bool)
                  n1039 = case shown="True" w2882 {
                    tunnel: w2893 -> [_ w2920]
                    tunnel: w2892 -> [_ w2911]
                    tunnel: w2891 -> [_ w2907]
                    tunnel: w2890 -> [_ w2905]
                    tunnel: w2889 -> [_ w2904]
                    tunnel: [FALSE w2903] -> w2885
                    tunnel: [w2899 w2902] -> w2880
                    tunnel: [FALSE TRUE] -> w2883
                    frame False {
                      n1040 = call "Display Message to User5"() -> ("error out"=w2899:errorcluster)  [unwired: 10 in, 1 out]
                    }
                    frame True {
                      n1041 = property on="VISA Tester" class="VISAName"() -> (error out=w2918:errorcluster, "Value"=w2917:refnum<visa-resource-name>)  [unwired: 2 in, 1 out]
                      n1042 = call "TesterOption (SubVI).vi"("2 Options"=FALSE, "error in (no error)"=w2918, "On/Off"=FALSE, "Tester Option"=T13."Venable", "VISA Refnum in"=w2917) -> ("error out"=w2913:errorcluster)  [unwired: 5 in, 1 out]
                      n1043 = call "Write panel message (SubVI).vi"("Stop BurnIn"=w2905, 4:"rpm"=w2904, 5:"rpm"=FALSE ("rpm"), "PrintTime"=FALSE, "Stop"=w2907, "error in (no error)"=w2913, "Time to wait"=3.0, "Strin"="TESTER BIT TEST OPERATION IN PROCESS\nPlease wait...", "String in"=w2911) -> ("error out"=w2912:errorcluster)  [unwired: 2 in]
                      n1044 = property on="UUT SoftwareVer" class="Str"() -> ("Value"=w2901:string)  [unwired: 2 in, 2 out]
                      n1045 = call "SerialMarvinSendGet.vi"("error in (no error)"=w2912, "write buffer"="VR\r\n", "VISA resource name"=w2920) -> ("error out"=w2902:errorcluster, "read buffer"=w2919:string)  [unwired: 7 in]
                      n1046 = Equal?(x=w2919, y=w2901) -> (x = y?=w2903:bool)
                    }
                  }
                  n1047 = case shown="False" w2885 {
                    tunnel: [enum16{"Stop", "Tests", "Bit test", "Start"}."Stop" enum16{"Stop", "Tests", "Bit test", "Start"}."Bit test"] -> w2884
                    tunnel: w2883 -> [w2894 _]
                    frame False {
                      n1048 = case shown="True" w2894 {
                        frame False {
                        }
                        frame True {
                          n1049 = call "Display Message to User4"() -> ()  [unwired: 10 in, 2 out]
                        }
                      }
                    }
                    frame True {
                    }
                  }
                }
              }
            }
            n1050 = Bundle By Name(cluster=T9 {"VISA"="COM1", "Array Test"=[]}, "VISA"=w2568, "Array Test"=w2574) -> (w2570:T9)
            n1051 = Enqueue Element(queue=w2576, element=w2570, error in (no error)=w2573) -> (queue out=w2571:refnum<queue>, error out=w2572:errorcluster)  [unwired: 2 out]
          }
          event "Report", "Stop Button": Value Change {
            w2937 = T31 1 items=["User Home"=0, "User Desktop"=1, "User Documents"=2, "User Application Data"=3, "User Preferences"=4, "User Temporary"=5, "Public Documents"=6, "Public Application Data"=7, "Public Preferences"=8, "Public Cache"=13, "System Core Libraries"=9, "System Installed Libraries"=10, "Application Files"=11, "Boot Volume Root"=12] ("system directory type")
            w2969 = "Marvin" ("section")
            n1052 = event-data() -> ("CtlRef"=w2961:refnum<vi>)  [unwired: 1 in]
            n1053 = local read "UUT"() -> (w2934:string)
            n1054 = call <vilib>:"Get System Directory.vi"("system directory type"=w2937) -> ("system directory"=w2936:path)  [unwired: 10 in]
            n1055 = Build Path(base path=w2936, name or relative path="MarvinReports") -> (appended path=w2998:path)
            n1056 = property on="CAN Status" class="Bool (strict)"() -> ("Value"=w2940:bool)  [unwired: 2 in, 2 out]
            n1057 = property on="Status" class="Bool (strict)"() -> ("Value"=w2941:bool)  [unwired: 2 in, 2 out]
            n1058 = case shown="\"AHU\"" w2934 {
              tunnel: ["REV EBAY" ("key") "REV AHU" ("key")] -> w2967
              frame "EBAY", Default {
              }
              frame "AHU" {
              }
            }
            n1059 = call <vilib>:"Check if File or Folder Exists.vi"("path"=w2998) -> ("error out"=w2996:errorcluster, "file or folder exists?"=w2999:bool, "dup path"=w2997:path)  [unwired: 8 in]
            n1060 = And(x=w2941, y=w2940) -> (x .and. y?=w2942:bool)
            n1061 = case shown="False" w2999 {
              tunnel: w2996 -> [w3063 w3064]
              tunnel: w2997 -> [w3062 w3065]
              tunnel: [w3061 w3065] -> w2939
              tunnel: [w3060 w3064] -> w3001
              frame False {
                n1062 = Create Folder(path (use dialog)=w3062, error in=w3063) -> (created path=w3061:path, error out=w3060:errorcluster)  [unwired: 1 in, 1 out]
              }
              frame True {
              }
            }
            n1063 = case shown="True" w2942 {
              tunnel: [w3008 w3028] -> w2985
              tunnel: [w3008 w3027] -> w2927
              tunnel: w2962 -> [_ w3016]
              tunnel: [w3008 w3021] -> w2932
              tunnel: [w3008 w3020] -> w2929
              tunnel: [w3008 w3024] -> w2955
              tunnel: [w3008 w3023] -> w2931
              tunnel: [w3008 w3012] -> w2928
              frame False {
                (unwired) "47"
                (unwired) " 413-8005_47_AHU"
                (unwired) "413-8005-1-47"
                (unwired) "5.3.9" ("read buffer")
                (unwired) "95"
                (unwired) "414-8005_95_EBAY_"
                (unwired) "414-8005-95"
                (unwired) "414-8005-95   "
                w3008 = "N_A" ("read buffer")
                n1064 = disable-structure shown="Disabled" {
                  frame Disabled {
                    n1065 = call "Display Message to User7"() -> ()  [unwired: 10 in, 2 out]
                  }
                  frame Enabled {
                  }
                }
                n1066 = Decimal String To Number(string="1" ("Value")) -> (number=w3009:i32)  [unwired: 2 in, 1 out]
                n1067 = Number To Decimal String(number=w3009, width (-)=i16 4) -> ()  [unwired: 1 out]
              }
              frame True {
                n1068 = call "SerialMarvinSendGet.vi"("write buffer"="SN\r\n", "VISA resource name"=w3016) -> ("error out"=w3015:errorcluster, "read buffer"=w3018:string)  [unwired: 8 in]
                n1069 = call "Time Delay2"("error in (no error)"=w3015) -> ("error out"=w3014:errorcluster)  [unwired: 10 in]
                n1070 = Decimal String To Number(string=w3018) -> (number=w3017:i32)  [unwired: 2 in, 1 out]
                n1071 = Number To Decimal String(number=w3017, width (-)=i16 4) -> (decimal integer string=w3021:string)
                n1072 = call "SerialMarvinSendGet.vi"("error in (no error)"=w3014, "write buffer"="VR\r\n", "VISA resource name"=w3016) -> ("error out"=w3025:errorcluster, "read buffer"=w3020:string)  [unwired: 7 in]
                n1073 = property on="UUT" class="DigNum (strict)"(error in=w3025) -> ("Value"=w3013:u8)  [unwired: 1 in, 2 out]
                n1074 = call "SentenceFromFile (SubVI).vi"("UUT"=w3013) -> ("Sentence"=w3012:string)  [unwired: 9 in, 1 out]
                n1075 = case shown="95, Default" w3013 {
                  tunnel: ["414-8005_95_EBAY_" " 413-8005_47_AHU" " 413-8005_63_AHU"] -> w3028
                  tunnel: ["414-8005-95   " w3034 w3037] -> w3027
                  tunnel: ["414-8005-95" w3034 w3037] -> w3024
                  tunnel: ["95" "47" "63"] -> w3023
                  frame 95, Default {
                  }
                  frame 47 {
                    w3034 = "413-8005-1-47"
                    (unwired) "AHU-L (47) 413-8005-1"
                  }
                  frame 63 {
                    w3037 = "413-8005-2-63"
                    (unwired) "AHU-R (63) 413-8005-2"
                  }
                }
              }
            }
            n1076 = Get Date/Time String(want seconds? (F)=TRUE) -> (date string=w3000:string)  [unwired: 2 in, 1 out]
            n1077 = call <vilib>:"Open Config Data.vi"("create file if necessary (T)"=FALSE, "configuration file path"=w2964) -> ("refnum"=w2976:T12)  [unwired: 1 in, 8 out]
            n1078 = property on="POWER Board S/N" class="Str"() -> ("Value"=w2926:string)  [unwired: 2 in, 2 out]
            n1079 = property on="Logger Path" class="Path"(error in=w3001, "Value"=w2939, "StartPath"=w2939) -> (error out=w2979:errorcluster)  [unwired: 1 in, 1 out]
            n1080 = Search and Replace String(replace all?=TRUE ("replace all? (F)"), input string=w3000, search string="/") -> (result string=w2982:string)  [unwired: 5 in, 3 out]
            n1081 = call-poly <vilib>:"Read Key.vi"("section"=w2969, "key"=w2967, "refnum"=w2976) -> ("error out"=w2971:errorcluster, "value"=w2974:string, "refnum out"=w2973:T12)  [unwired: 5 in, 1 out]
            n1082 = property on="DSP Board S/N" class="Str"() -> ("Value"=w2925:string)  [unwired: 2 in, 2 out]
            n1083 = call-poly <vilib>:"Read Key.vi"("section"=w2969, "error in (no error)"=w2971, "key"="Tester Software Ver", "refnum"=w2973) -> ("error out"=w2968:errorcluster, "value"=w2930:string, "refnum out"=w2972:T12)  [unwired: 4 in, 1 out]
            n1084 = Concatenate Strings("ATR" ("string"), w2985, w2932, "_", w2982, ".docx" ("string")) -> (w2980:string)
            n1085 = call <vilib>:"Close Config Data.vi"("error in (no error)"=w2968, "refnum"=w2972) -> ()  [unwired: 8 in, 2 out]
            n1086 = Build Path(base path=w2939, name or relative path=w2980) -> (appended path=w2981:path)
            n1087 = Concatenate Strings("  Rev-" ("string"), w2974) -> (w2963:string)
            n1088 = while {
              tunnel: w2980 -> [w3045]
              tunnel: w2939 -> [w3042]
              shift-right: [w3044] -> w2978
              shift-left: w2981 -> [w3043]
              shift-right: [w3040] -> w2965
              shift-left: w2966 -> [w3041]
              tunnel: w2979 -> [w3046]
              tunnel: [w3047] -> w2938
              stop <- w3039 continue-if-true
              n1089 = call <vilib>:"Check if File or Folder Exists.vi"("error in (no error)"=w3046, "path"=w3043) -> ("error out"=w3047:errorcluster, "file or folder exists?"=w3039:bool)  [unwired: 7 in, 1 out]
              n1090 = case shown="True" w3039 {
                tunnel: w3045 -> [_ w3059]
                tunnel: w3041 -> [_ w3051]
                tunnel: [w3049 w3056] -> w3044
                tunnel: w3043 -> [w3049 _]
                tunnel: w3042 -> [_ w3057]
                tunnel: [1 w3050] -> w3040
                frame False {
                }
                frame True {
                  w3052 = ".docx" ("search string")
                  n1091 = Search and Replace String(input string=w3059, search string=w3052) -> (result string=w3058:string)  [unwired: 6 in, 3 out]
                  n1092 = Number To Decimal String(number=w3051) -> (decimal integer string=w3054:string)  [unwired: 1 in]
                  n1093 = call <vilib>:"Space Constant.vi"() -> ("String"=w3053:string)
                  n1094 = Concatenate Strings(w3058, w3053, w3054, w3052) -> (w3055:string)
                  n1095 = Build Path(base path=w3057, name or relative path=w3055) -> (appended path=w3056:path)
                  n1096 = Increment(x=w3051) -> (x+1=w3050:i32)
                }
              }
            }
            n1097 = call "HeaderBis.vi"("UUTHeader"=w2934, "UA"=w2931, "POWER SN"=w2926, "Revision Param"=w2928, "P/N UUT"=w2927, "DSP SN"=w2925, "Driver S/N"=w2932, "VR"=w2929, "Oper."=w2933, "Tester Software Ver"=w2930) -> ("table header"=w2924:string, "Array"=w2923:string[][])  [unwired: 3 in, 1 out]
            n1098 = Open/Create/Replace File(file path (use dialog)=w2978, error in=w2938, operation (0:open)=T25."create") -> (error out=w2991:errorcluster)  [unwired: 3 in, 2 out]
            n1099 = control-ref of="ATR"() -> (w3003:refnum<vi>)
            n1100 = property class="Tbl (strict)"(reference=w3003, error in=w2991) -> ("Value"=w3004:string[][])  [unwired: 2 out]
            n1101 = call "MarvinReport.vi"("HEADER1"=w2924, "ATR Or"=w3003, "Steps   pfull"=w3004, "Footer UUT"=w2955, "pageNum"=3, "InputHeaderArray"=w2923, "FILE NAME"=w2980, "Report Folder"=w2978, "REV"=w2963, "Test-Conductor"=w2933) -> ("error out"=w2950:errorcluster)  [unwired: 4 in, 1 out]
            n1102 = call <vilib>:"Clear Errors.vi"("error in (no error)"=w2950) -> ("error out"=w2949:errorcluster)  [unwired: 5 in, 1 out]
            n1103 = property class="Bool (strict)"(reference=w2961, error in=w2949) -> ("BoolText.Text"=w2960:string)  [unwired: 2 out]
            n1104 = Equal?(x=w2960, y="Report") -> (x = y?=w2954:bool)
            n1105 = Select(t=T11."MainProgram", s=w2954, f=T11."Stop") -> (s? t:f=w2957:T11)
            n1106 = Select(t="Save Report...", s=w2954, f="Program Stopped...\r\nPlease turn OFF All Power sinks") -> (s? t:f=w2952:string)
            n1107 = property on="Report" class="Bool (strict)"(error in=w2949, "Value"=FALSE ("Report")) -> (error out=w2943:errorcluster)  [unwired: 1 in, 1 out]
            n1108 = property on="VISA Tester" class="VISAName"() -> ("Value"=w2947:refnum<visa-resource-name>)  [unwired: 2 in, 2 out]
            n1109 = property on="Pannel User Message" class="Str"("Value"=w2952) -> ()  [unwired: 2 in, 2 out]
            n1110 = call "TesterOption (SubVI).vi"("2 Options"=FALSE, "error in (no error)"=w2943, "On/Off"=FALSE, "Tester Option"=T13."Venable", "VISA Refnum in"=w2947) -> ()  [unwired: 5 in, 2 out]
          }
          event "Help Button": Value Change {
            n1111 = event-data() -> ()  [unwired: 1 in, 6 out]
            n1112 = vi-ref "Help.vi"() -> (w3079:refnum<vi>)
            n1113 = invoke class="VI" method="FP.Open"(reference=w3079, error in=w3077, "Activate"=TRUE ("Activate?"), "State"=T23."Standard") -> (error out=w3078:errorcluster)  [unwired: 1 in, 4 out]
            n1114 = call "Help.vi"("error in"=w3078, "TesterSWVersion"=w3069) -> ("error out"=w3076:errorcluster)  [unwired: 6 in]
            n1115 = property on="Help Button" class="Bool (strict)"("Value"=FALSE ("Help Button")) -> ()  [unwired: 2 in, 2 out]
          }
          event "Serial Com": Value Change {
            n1116 = event-data() -> ()  [unwired: 1 in, 6 out]
            n1117 = property on="Serial Com" class="Bool"(error in=w3090, "Visible"=FALSE) -> (error out=w3094:errorcluster)  [unwired: 1 in, 1 out]
            n1118 = property on="VISA Marvin" class="VISAName"(error in=w3094, "Visible"=TRUE) -> (error out=w3091:errorcluster)  [unwired: 1 in, 1 out]
          }
          event "VISA Marvin": Value Change {
            n1119 = event-data() -> ()  [unwired: 1 in, 6 out]
            n1120 = property on="Serial Com" class="Bool"(error in=w3099, "Visible"=FALSE) -> (error out=w3098:errorcluster)  [unwired: 1 in, 1 out]
            n1121 = control-ref of="This VI"() -> (w3110:refnum<vi>)
            n1122 = property on="Pannel User Message" class="Str"(error in=w3099, "Value"="Serial connection in process" ("Pannel User Message")) -> ()  [unwired: 1 in, 2 out]
            n1123 = call "Serial InitMarvin.vi"("error in (no error)"=w3098, "VI reference (current VI)"=w3110, "VISA Refnum in"="VISA Marvin") -> ("error out"=w3102:errorcluster, "Boolean"=w3100:bool)  [unwired: 7 in]
            n1124 = property on="VISA Marvin" class="VISAName"(error in=w3102, "Visible"=FALSE) -> (error out=w3113:errorcluster)  [unwired: 1 in, 1 out]
            n1125 = property on="Serial Com" class="Bool"(error in=w3113, "Visible"=TRUE) -> (error out=w3109:errorcluster)  [unwired: 1 in, 1 out]
            n1126 = case shown="True" w3100 {
              tunnel: w3109 -> [w3116 w3128]
              tunnel: "VISA Marvin" -> [w3117 w3125]
              tunnel: [w3117 w3124] -> w3104
              tunnel: [w3116 w3123] -> w3103
              frame False {
              }
              frame True {
                n1127 = call "SerialMarvinSendGet.vi"("error in (no error)"=w3128, "Clear Log"=FALSE, "write buffer"="VC\r\n", "VISA resource name"=w3125) -> ("error out"=w3127:errorcluster, "read buffer"=w3121:string)  [unwired: 6 in]
                n1128 = Decimal String To Number(string=w3121) -> (number=w3120:i32)  [unwired: 2 in, 1 out]
                n1129 = Less Or Equal?(x=w3120, y=50) -> (x <= y?=w3118:bool)
                n1130 = property on="Status" class="Bool (strict)"("Value"=w3118) -> ()  [unwired: 2 in, 2 out]
                n1131 = case shown="True" w3118 {
                  tunnel: w3127 -> [w3129 w3158]
                  tunnel: w3125 -> [w3130 w3157]
                  tunnel: [w3130 w3148] -> w3124
                  tunnel: [w3129 w3131] -> w3123
                  frame False {
                  }
                  frame True {
                    n1132 = call <vilib>:"Clear Errors.vi"("error in (no error)"=w3158) -> ("error out"=w3159:errorcluster)  [unwired: 5 in, 1 out]
                    n1133 = control-ref of="ATR"() -> (w3145:refnum<vi>)
                    n1134 = VISA Flush I/O Buffer(VISA resource name=w3157, error in (no error)=w3159) -> (VISA resource name out=w3148:refnum<visa-resource-name>, error out=w3156:errorcluster)  [unwired: 1 in]
                    n1135 = call "Display Message to User2"("error in (no error)"=w3156) -> ("error out"=w3155:errorcluster, "Yes"=w3154:bool)  [unwired: 9 in]
                    n1136 = case shown="True" w3154 {
                      tunnel: w3155 -> [w3160 w3182]
                      tunnel: [w3160 w3161] -> w3153
                      tunnel: w3148 -> [_ w3179]
                      frame False {
                      }
                      frame True {
                        w3167 = FALSE ("2 Options")
                        n1137 = property on="UUT" class="DigNum (strict)"() -> ("Value"=w3181:u8)  [unwired: 2 in, 2 out]
                        n1138 = call "SetParam.vi"("RS"=TRUE, "error in (no error)"=w3182, "Param to Set in"=w3181, "Visa"=w3179) -> ("error out"=w3162:errorcluster)  [unwired: 7 in]
                        n1139 = control-ref of="Pannel User Message"() -> (w3178:refnum<vi>)
                        n1140 = control-ref of="Stop Burn-in"() -> (w3176:refnum<vi>)
                        n1141 = control-ref of="Stop Button"() -> (w3177:refnum<vi>)
                        n1142 = control-ref of="Motor Speed RPM"() -> (w3175:refnum<vi>)
                        n1143 = property on="VISA Tester" class="VISAName"() -> ("Value"=w3171:refnum<visa-resource-name>)  [unwired: 2 in, 2 out]
                        n1144 = call "TesterOption (SubVI).vi"("2 Options"=w3167, "error in (no error)"=w3162, "On/Off"=FALSE, "Tester Option"=T13."Power", "VISA Refnum in"=w3171) -> ("error out"=w3172:errorcluster, "VISA Refnum out"=w3174:refnum<visa-resource-name>)  [unwired: 5 in]
                        n1145 = call "Write panel message (SubVI).vi"("Stop BurnIn"=w3176, "rpm"=w3175, "PrintTime"=TRUE, "Stop"=w3177, "error in (no error)"=w3172, "Time to wait"=20.0, "Strin"="Restart the UUT\nPlease wait...", "String in"=w3178) -> ("error out"=w3173:errorcluster)  [unwired: 3 in]
                        n1146 = call "TesterOption (SubVI).vi"("2 Options"=w3167, "error in (no error)"=w3173, "On/Off"=FALSE, "Tester Option"=T13."Venable", "VISA Refnum in"=w3174) -> ("error out"=w3161:errorcluster)  [unwired: 5 in, 1 out]
                      }
                    }
                    n1147 = call "Find_Number_LineMARVIN.vi"("Test Paragraph"="Sensor Reading Analog Offset", "TableIn"=w3145) -> ("Line number"=w3146:i32)  [unwired: 3 in, 3 out]
                    n1148 = call "SerialMarvinSendGet.vi"("error in (no error)"=w3153, "write buffer"="SN\r\n", "VISA resource name"=w3148) -> ("error out"=w3149:errorcluster, "read buffer"=w3138:string)  [unwired: 7 in]
                    n1149 = call "SerialMarvinSendGet.vi"("error in (no error)"=w3149, "write buffer"="AO[1]\r\n", "VISA resource name"=w3148) -> ("error out"=w3143:errorcluster, "read buffer"=w3144:string)  [unwired: 7 in]
                    n1150 = Fract/Exp String To Number(string=w3144) -> (number=w3140:dbl)  [unwired: 3 in, 1 out]
                    n1151 = In Range and Coerce(upper limit=0.1 ("x"), x=w3140, lower limit=-0.1) -> (In Range?=w3139:bool)  [unwired: 1 out]
                    n1152 = call "PassOrFail (SubVI).vi"("Test#"="2", "index (row)"=w3146, "error in (no error)"=w3143, "Data in"=w3140, "Pass?Fail"=w3139, "Table in"=w3145) -> ("error out"=w3132:errorcluster)  [unwired: 5 in]
                    n1153 = property on="VISA Marvin" class="VISAName"(error in=w3132) -> (error out=w3135:errorcluster, "Value"=w3136:refnum<visa-resource-name>)  [unwired: 1 in, 1 out]
                    n1154 = call "SerialMarvinSendGet.vi"("error in (no error)"=w3135, "Clear Log"=FALSE, "write buffer"="EP=1\r\nMD[1]=1\r\n", "VISA resource name"=w3136) -> ("error out"=w3131:errorcluster)  [unwired: 6 in, 1 out]
                    n1155 = property on="UUT SN Report" class="Str"("Value"=w3138) -> ()  [unwired: 2 in, 2 out]
                    n1156 = Decimal String To Number(string=w3138) -> (number=→"Current SN":i32)  [unwired: 2 in, 1 out]
                  }
                }
              }
            }
          }
          event "Refresh Button": Value Change {
            n1157 = event-data() -> ()  [unwired: 1 in, 6 out]
          }
          event "Settings": Value Change {
            n1158 = event-data() -> ()  [unwired: 1 in, 6 out]
            n1159 = control-ref of="VISA Tester"() -> (w3196:refnum<vi>)
            n1160 = control-ref of="UUT"() -> (w3194:refnum<vi>)
            n1161 = property on="Status" class="Bool (strict)"() -> ("Value"=w3198:bool)  [unwired: 2 in, 2 out]
            n1162 = case shown="True" w3198 {
              tunnel: w3204 -> [_ w3216]
              tunnel: [w3205 w3211] -> w3199
              tunnel: w3197 -> [_ w3210]
              tunnel: w3196 -> [_ w3209]
              tunnel: w3195 -> [_ w3208]
              tunnel: w3194 -> [_ w3207]
              frame False {
                n1163 = call "Display Message to User8"() -> ("error out"=w3205:errorcluster)  [unwired: 10 in, 1 out]
              }
              frame True {
                n1164 = vi-ref "Calibration (SubVI).vi"() -> (w3215:refnum<vi>)
                n1165 = invoke class="VI" method="FP.Open"(reference=w3215, error in=w3216, "Activate"=TRUE ("Activate?"), "State"=T23."Standard") -> (error out=w3212:errorcluster)  [unwired: 1 in, 4 out]
                n1166 = call "Calibration (SubVI).vi"("VISA UUT"=w3210, "error constant"=w3212, "UUT"=w3207, "CAN Cluster in"=w3208, "Visa Tester"=w3209) -> ("error constant 2"=w3211:errorcluster, "AO[1]Meas"=→"Cal":dbl)  [unwired: 5 in]
              }
            }
          }
        }
      }
      frame "Initialize" {
        w3217 = 0
        w3222 = FALSE ("Visible")
        w3223 = FALSE ("Visible")
        w3224 = FALSE ("Visible")
        w3225 = FALSE ("Visible")
        w3236 = refnum<visa-resource-name> "COM1" ("VISA resource name")
        w3227 = FALSE ("Visible")
        w3220 = FALSE ("Serial Status")
        n1167 = property on="ComTestResult" class="Bool (strict)"("Value"=w3225) -> ()  [unwired: 2 in, 2 out]
        n1168 = property on="VenableResult" class="Bool (strict)"("Value"=w3225) -> ()  [unwired: 2 in, 2 out]
        n1169 = property on="VenableDirectionResult" class="Bool (strict)"("Value"=w3225) -> ()  [unwired: 2 in, 2 out]
        n1170 = property on="SpeedResult" class="Bool (strict)"("Value"=w3225) -> ()  [unwired: 2 in, 2 out]
        n1171 = property on="Serial Com" class="Bool"(error in=errorcluster {"status"=FALSE, "code"=0, "source"=""} ("error out"), "Visible"=TRUE) -> (error out=w3238:errorcluster)  [unwired: 1 in, 1 out]
        n1172 = property on="AuxiOFFResult" class="Bool (strict)"("Value"=w3224) -> ()  [unwired: 2 in, 2 out]
        n1173 = property on="AuxiONResult" class="Bool (strict)"("Value"=w3224) -> ()  [unwired: 2 in, 2 out]
        n1174 = property on="VisualInspectionResult" class="Bool (strict)"("Value"=w3224) -> ()  [unwired: 2 in, 2 out]
        n1175 = property on="SensCalResult" class="Bool (strict)"("Value"=w3224) -> ()  [unwired: 2 in, 2 out]
        n1176 = property on="VISA Marvin" class="VISAName"(error in=w3238, "Visible"=w3227, "Value"=w3236) -> (error out=w3228:errorcluster)  [unwired: 1 in, 1 out]
        n1177 = property on="Stop Burn-in" class="Bool (strict)"(error in=w3228, "Visible"=w3227) -> (error out=w3221:errorcluster)  [unwired: 1 in, 1 out]
        n1178 = property on="BurnDC" class="Bool (strict)"("Value"=w3223) -> ()  [unwired: 2 in, 2 out]
        n1179 = property on="BurnTemp" class="Bool (strict)"("Value"=w3223) -> ()  [unwired: 2 in, 2 out]
        n1180 = property on="BurnSpeed" class="Bool (strict)"("Value"=w3223) -> ()  [unwired: 2 in, 2 out]
        n1181 = property on="BurnResult" class="Bool (strict)"("Value"=w3223) -> ()  [unwired: 2 in, 2 out]
        n1182 = property on="Refresh Button" class="Bool (strict)"(error in=w3221, "Value"=FALSE ("Refresh Button")) -> ()  [unwired: 1 in, 2 out]
        n1183 = property on="StopTimeResult" class="Bool (strict)"("Value"=w3222) -> ()  [unwired: 2 in, 2 out]
        n1184 = property on="MotorTempResult" class="Bool (strict)"("Value"=w3222) -> ()  [unwired: 2 in, 2 out]
        n1185 = property on="TempControlResult" class="Bool (strict)"("Value"=w3222) -> ()  [unwired: 2 in, 2 out]
        n1186 = property on="Automation" class="Bool (strict)"("Value"=w3222) -> ()  [unwired: 2 in, 2 out]
        n1187 = flat-sequence {
          tunnel: w3221 -> [w3240]
          tunnel: [w3240] -> w3218
          tunnel: [w3242] -> w3234
          tunnel: w3218 -> [w3242]
          tunnel: [w3254] -> w3233
          tunnel: w3234 -> [w3255]
          tunnel: [w3255] -> w3232
          frame #0 {
          }
          frame #1 {
            w3245 = u32 4294967295  # AccMask
            w3241 = T5 0 items=["使用Flash参数", "使用界面设置参数"] ("InitFlag")
            w3243 = T7 0 items=["normal operation", "Listen-only mode", "test mode"]  # Mode
            w3244 = T6 3 items=["接收所有类型"=1, "只接收标准帧"=2, "只接收扩展帧"=3] ("Fliter")
            w3249 = u8 10 items=["5k bps"=1, "10k bps"=2, "20k bps"=3, "40k bps"=4, "50k bps"=5, "80k bps"=6, "100k bps"=7, "125k bps"=8, "200k bps"=9, "250k bps"=10, "400k bps"=11, "500k bps"=12, "666k bps"=13, "800k bps"=14, "1000k bps"=15, "33.33k bps"=16, "66.66k bps"=17, "83.33k bps"=18]  # kBaudRate
            w3246 = u32 0  # AccCode
            w3247 = T3 4 items=["USB-CAN"=3, "USB-CAN2"=4] ("DevType")
            w3248 = T8 {"DevType"=3, "DevIndex"=0, "CanIndex"=0, "VCI_INIT_CONFIG"={"AccCode"=0, "AccMask"=0, "InitFlag"=1, "Fliter"=7, "Timing0"=0, "Timing1"=0, "Mode"=0}}  # Config
            # "CANalystII"
            n1188 = call "Demo_GetT0T1.vi"("kBaudRate"=w3249) -> ("Timing0"=w3251:u8, "Timing1"=w3252:u8)
            n1189 = Bundle By Name(cluster=w3248, "DevType"=w3247, "CanIndex"="Channel 2", "VCI_INIT_CONFIG.AccCode"=w3246, "VCI_INIT_CONFIG.AccMask"=w3245, "VCI_INIT_CONFIG.InitFlag"=w3241, "VCI_INIT_CONFIG.Fliter"=w3244, "VCI_INIT_CONFIG.Timing0"=w3251, "VCI_INIT_CONFIG.Timing1"=w3252, "VCI_INIT_CONFIG.Mode"=w3243) -> (→"Config_CANAT":T8)
          }
          frame #2 {
            w3256 = u16 284 items=["1M"=20, "500K"=28, "250K"=284, "125K"=796, "100K"=17199, "50K"=18223, "20K"=21295, "10K"=26415, "5K"=32639] ("baud in")
            n1190 = control-ref of="Config_CANAT"() -> (w3254:refnum<vi>)
            n1191 = call "InitCAN_ATII.vi"("Config"=w3254) -> ("Sts"=→"CAN Status":bool)
            n1192 = call "ChangeCANBaud.vi"("baud in"=w3256, "reference"=w3254) -> ()
          }
        }
        "Status" <- w3220
        "Test Failed" <- w3220
      }
    }
  }
  n1193 = property on="Settings" class="Bool (strict)"("Visible"=w20) -> ()  [unwired: 2 in, 2 out]
  n1194 = property on="Cal" class="DigNum (strict)"("Visible"=w20) -> ()  [unwired: 2 in, 2 out]
  n1195 = disable-structure shown="Disabled" {
    frame Disabled {
      w3258 = T21."Disabled and Grayed Out" ("Disabled")
      w3259 = FALSE ("Start")
      n1196 = property on="VISA Tester" class="VISAName" props=["Value"]() -> ()  [unwired: 2 in, 3 out]
      n1197 = property on="Current SN" class="DigNum (strict)" props=["Value"]() -> ()  [unwired: 2 in, 3 out]
      n1198 = property on="UUT" class="DigNum (strict)" props=["Value"]() -> ()  [unwired: 2 in, 3 out]
      n1199 = property on="Status" class="Bool (strict)" props=["Value"]() -> ()  [unwired: 2 in, 3 out]
      n1200 = property on="UUT SoftwareVer" class="Str" props=["Value"]() -> ()  [unwired: 2 in, 3 out]
      n1201 = property on="Next SN" class="DigNum (strict)" props=["Value"]() -> ()  [unwired: 3 in, 2 out]
      n1202 = property on="Start" class="Bool (strict)"("Value"=w3259, "DisabledEnum"=w3258) -> ()  [unwired: 2 in, 2 out]
      n1203 = property on="Report" class="Bool (strict)"("Value"=w3259, "DisabledEnum"=w3258) -> ()  [unwired: 2 in, 2 out]
    }
    frame Enabled {
    }
  }
  n1204 = disable-structure shown="Disabled" {
    frame Disabled {
      (unwired) 0.02003173828125 ("x")
      n1205 = control-ref of="Stop Burn-in"() -> ()  [unwired: 1 out]
      n1206 = control-ref of="Stop Button"() -> ()  [unwired: 1 out]
      n1207 = control-ref of="Motor Speed RPM"() -> ()  [unwired: 1 out]
      n1208 = control-ref of="Config_CANAT"() -> ()  [unwired: 1 out]
      n1209 = control-ref of="UUT"() -> ()  [unwired: 1 out]
      n1210 = call "GetADCTester (SubVI).vi"() -> ()  [unwired: 9 in, 3 out]
      n1211 = call "CANSendMotorSpeed.vi"() -> ()  [unwired: 11 in, 1 out]
      n1212 = control-ref of="Config_CANAT"() -> ()  [unwired: 1 out]
      n1213 = call "Find_Number_LineMARVIN.vi"() -> ()  [unwired: 5 in, 4 out]
      n1214 = property on="UUT" class="DigNum (strict)" props=["Value"]() -> ()  [unwired: 2 in, 3 out]
      n1215 = control-ref of="UUT"() -> ()  [unwired: 1 out]
      n1216 = call "DegToDAC (SubVI).vi"() -> ()  [unwired: 10 in, 2 out]
      n1217 = call "Write panel message (SubVI).vi"() -> ()  [unwired: 11 in, 1 out]
      n1218 = property on="VISA Tester" class="VISAName" props=["Value"]() -> ()  [unwired: 2 in, 3 out]
      n1219 = control-ref of="ATR"() -> ()  [unwired: 1 out]
      n1220 = call "TesterOption (SubVI).vi"() -> ()  [unwired: 10 in, 2 out]
      n1221 = call "TesterOption (SubVI).vi"() -> ()  [unwired: 10 in, 2 out]
      n1222 = call "PassOrFail (SubVI).vi"() -> ()  [unwired: 11 in, 1 out]
    }
    frame Enabled {
    }
  }
  n1223 = disable-structure shown="Disabled" {
    frame Disabled {
      n1224 = flat-sequence {
        frame #0 {
          n1225 = call "CANSendMotorSpeed.vi"("Remote"=TRUE, "Motor Speed RPM"=u16 0) -> ("error out"=w3261:errorcluster, "UUT"=w3264:refnum<vi>)  [unwired: 8 in]
          n1226 = property on="VISA Tester" class="VISAName"() -> ("Value"=w3260:refnum<visa-resource-name>)  [unwired: 2 in, 2 out]
          n1227 = call "TesterOption (SubVI).vi"("error in (no error)"=w3261, "On/Off"=FALSE, "Tester Option"=T13."Power", "VISA Refnum in"=w3260) -> ()  [unwired: 6 in, 2 out]
        }
      }
    }
    frame Enabled {
    }
  }
  "Pannel User Message" <- w19
